vi "AO_master_DM_WFS_v3.vi"() -> ()   [LabVIEW 2018]
uses:
  <userlib>/WaveKit.lib/Controls/Image information.ctl
  <userlib>/WaveKit.lib/Controls/Image general information.ctl
  <userlib>/WaveKit.lib/Controls/Image acquisition information.ctl
  <userlib>/WaveKit.lib/Controls/Point2D.ctl
  <userlib>/WaveKit.lib/Controls/Data alignment enum.ctl
  <userlib>/WaveKit.lib/Controls/StatisticsData.ctl
  <userlib>/WaveKit.lib/Controls/Wavefront Corrector states - ONE.ctl
  Drivers and controls/ASI/ASI_VIs/ASI Library/Shared_Serial/Axis Name.ctl
  <userlib>/WaveKit.lib/Classes/Camera/Camera.lvclass
  <userlib>/WaveKit.lib/Classes/CameraSet/CameraSet.lvclass
  <userlib>/WaveKit.lib/Classes/Image/Image.lvclass
  <userlib>/WaveKit.lib/Classes/Phase/Phase.lvclass
  <userlib>/WaveKit.lib/Controls/HasoSlopes.lvclass
  <userlib>/WaveKit.lib/Controls/Pupil.lvclass
  <userlib>/WaveKit.lib/Classes/WavefrontCorrector/WavefrontCorrector.lvclass
  <userlib>/WaveKit.lib/Classes/WavefrontCorrectorSet/WavefrontCorrectorSet.lvclass
  <userlib>/WaveKit.lib/Classes/HasoEngine/HasoEngine.lvclass
  <userlib>/WaveKit.lib/Controls/SlopesEngineSetup.ctl
  <userlib>/WaveKit.lib/Controls/WavefrontReconstructionMode.ctl
  <vilib>/Utility/file.llb/Read From Spreadsheet File (DBL).vi
  <vilib>/Analysis/1siggen.llb/Ramp Pattern by Delta.vi
  <userlib>/WaveKit.lib/Classes/ModalCoef/ModalCoef.lvclass
  <vilib>/Analysis/NI_AALBase.lvlib
panel:
  in  "Device Status":enum32{"DM", "WFS", "Camera", "Others"}(tab)=enum."Camera"
  out "DM Actuator Values":sgl[](graph)
  out "Initial State":T1[](array[typedef])
  out "ActuatorsNumber":i32
  out "Initial Positions":sgl[](array[numeric])
  out "Final Positions":sgl[](array[numeric])
  in  "Coef Min":dbl=-0.5 min=1.0
  in  "Coef Max":dbl=0.5 min=1.0
  out "Zernike Measured":dbl[](graph)
  out "Phase statistics":T2
  out "Phase values":sgl[][](graph)=[[nan, nan, nan, nan, nan, nan, nan, nan, nan, nan, nan, nan, nan, nan, nan, nan, nan, nan, nan, nan, nan, nan, nan, nan, nan, nan, nan, nan, nan, nan, nan, nan, nan, nan, nan, nan, nan, nan, nan, nan], [nan, nan, nan, nan, nan, nan, nan, nan, nan, nan, nan, nan, nan, nan, nan, nan, nan, nan, nan, nan, nan, nan, nan, nan, nan, nan, nan, nan, nan, nan, nan, nan, nan, nan, nan, nan, nan, nan, nan, nan], [nan, nan, nan, nan, nan, nan, nan, nan, nan, nan, nan, nan, nan, nan, nan, nan, nan, nan, nan, nan, nan, nan, nan, nan, nan, nan, nan, nan, nan, nan, nan, nan, nan, nan, nan, nan, nan, nan, nan, nan], [nan, nan, nan, nan, nan, nan, nan, nan, nan, nan, nan, nan, nan, nan, nan, nan, nan, nan, nan, nan, nan, nan, nan, nan, nan, nan, nan, nan, nan, nan, nan, nan, nan, nan, nan, nan, nan, nan, nan, nan], [nan, nan, nan, nan, nan, nan, nan, nan, nan, nan, nan, nan, nan, nan, -0.14441992, nan, 0.1501734, 0.22490476, 0.2674259, 0.28415325, 0.2792031, 0.2552752, 0.21375881, 0.15405469, nan, nan, nan, nan, nan, nan, nan, nan, nan, nan, nan, nan, nan, nan, nan, nan], [nan, nan, nan, nan, nan, nan, nan, nan, nan, nan, nan, nan, nan, nan, 0.19143742, 0.2795512, 0.33646506, 0.37099743, 0.3877919, 0.3894302, 0.37774685, 0.35447162, 0.3212538, 0.27904776, 0.22675864, 0.15897867, nan, nan, nan, nan, nan, nan, nan, nan, nan, nan, nan, nan, nan, nan], [nan, nan, nan, nan, nan, nan, nan, nan, nan, nan, nan, nan, nan, 0.22618562, 0.290776, 0.33285964, 0.36044422, 0.3767934, 0.38285175, 0.37884915, 0.3652757, 0.3433441, 0.3149789, 0.28229773, 0.2464756, 0.20580466, 0.15268901, 0.06923797, nan, nan, nan, nan, nan, nan, nan, nan, nan, nan, nan, nan], [nan, nan, nan, nan, nan, nan, nan, nan, nan, nan, nan, nan, 0.19992779, 0.24616541, 0.27565512, 0.29675642, 0.31222007, 0.32191983, 0.32467726, 0.31943765, 0.30597392, 0.2852214, 0.25927368, 0.2309889, 0.20308714, 0.17653626, 0.14795627, 0.10568966, 0.024115691, nan, nan, nan, nan, nan, nan, nan, nan, nan, nan, nan], [nan, nan, nan, nan, nan, nan, nan, nan, nan, nan, nan, 0.14862825, 0.18219855, 0.20114602, 0.21551609, 0.22862102, 0.24014233, 0.24817906, 0.2505626, 0.24567793, 0.23295718, 0.21313797, 0.18829979, 0.16161954, 0.1367108, 0.11633411, 0.10019377, 0.081457645, 0.04156301, -0.057204023, nan, nan, nan, nan, nan, nan, nan, nan, nan, nan], [nan, nan, nan, nan, nan, nan, nan, nan, nan, nan, 0.08899155, 0.117771566, 0.12948777, 0.13732892, 0.14631097, 0.15688494, 0.16728252, 0.17497937, 0.17758016, 0.17335457, 0.16157834, 0.14275661, 0.11873307, 0.09261118, 0.06834036, 0.04974218, 0.038678437, 0.031985473, 0.016725859, -0.03676957, nan, nan, nan, nan, nan, nan, nan, nan, nan, nan], [nan, nan, nan, nan, nan, nan, nan, nan, nan, nan, 0.058377307, 0.069048055, 0.0725615, 0.07683456, 0.0840318, 0.09335055, 0.10271386, 0.1097376, 0.11226265, 0.10867052, 0.09812171, 0.08078306, 0.058033932, 0.032565817, 0.008214329, -0.010712444, -0.020921554, -0.022825297, -0.02489755, -0.05023362, -0.14592764, nan, nan, nan, nan, nan, nan, nan, nan, nan], [nan, nan, nan, nan, nan, nan, nan, nan, nan, -0.0018393314, 0.018310271, 0.023098737, 0.024714457, 0.027986258, 0.033823933, 0.041292578, 0.048749834, 0.054400377, 0.056548227, 0.05374936, 0.04499338, 0.029967438, 0.009379062, -0.014759185, -0.03905803, -0.059140373, -0.070816256, -0.0724436, -0.06894927, -0.07806298, -0.1393881, nan, nan, nan, nan, nan, nan, nan, nan, nan], [nan, nan, nan, nan, nan, nan, nan, nan, nan, -0.03322208, -0.017045017, -0.0123043535, -0.010394985, -0.007970343, -0.0042642877, 0.0003761826, 0.005164365, 0.009095938, 0.010986101, 0.009512841, 0.0033822758, -0.008344227, -0.02579559, -0.047820807, -0.071688615, -0.09321856, -0.107681155, -0.11187886, -0.10789668, -0.10908524, -0.14891545, -0.29341945, nan, nan, nan, nan, nan, nan, nan, nan], [nan, nan, nan, nan, nan, nan, nan, nan, nan, nan, -0.043187555, -0.03622458, -0.033755217, -0.03278728, -0.03198469, -0.030707732, -0.028716512, -0.026208155, -0.023933899, -0.023217455, -0.025771504, -0.03328519, -0.04682974, -0.06620631, -0.08943447, -0.1126552, -0.13079928, -0.13944486, -0.13836564, -0.13734597, -0.16491348, -0.2807172, nan, nan, nan, nan, nan, nan, nan, nan], [nan, nan, nan, nan, nan, nan, nan, nan, -0.13038255, -0.08328184, -0.060542934, -0.050779276, -0.048053104, -0.048984695, -0.05126809, -0.053124577, -0.05330209, -0.051303368, -0.04760214, -0.04368073, -0.041799206, -0.04448101, -0.05377527, -0.07043236, -0.09320336, -0.118551016, -0.14113419, -0.15550357, -0.15952203, -0.16009864, -0.18189941, -0.27977645, nan, nan, nan, nan, nan, nan, nan, nan], [nan, nan, nan, nan, nan, nan, nan, nan, -0.15416794, -0.09987456, -0.07151361, -0.05893044, -0.056102008, -0.058817875, -0.063637674, -0.067669004, -0.06878706, -0.06599128, -0.059670344, -0.051622536, -0.044753395, -0.042448726, -0.04769562, -0.062100213, -0.08502676, -0.11315687, -0.14084403, -0.16171429, -0.1720384, -0.17647736, -0.19687745, -0.284868, -0.53908885, -1.12795, nan, nan, nan, nan, nan, nan], [nan, nan, nan, nan, nan, nan, nan, nan, -0.17633308, -0.1131372, -0.07876157, -0.06330658, -0.060116876, -0.063924976, -0.07015394, -0.07493687, -0.07548633, -0.07052183, -0.060539607, -0.047784284, -0.035856243, -0.028966732, -0.030924596, -0.044017438, -0.06802279, -0.099662215, -0.13288532, -0.16044727, -0.17731819, -0.18653797, -0.20820689, -0.29237592, -0.5366785, nan, nan, nan, nan, nan, nan, nan], [nan, nan, nan, nan, nan, nan, nan, nan, -0.19826387, -0.12505035, -0.08430402, -0.06564974, -0.061443567, -0.06527472, -0.07152294, -0.07554153, -0.07411167, -0.0658889, -0.05163869, -0.034133032, -0.017655006, -0.0071354215, -0.007018423, -0.020031396, -0.046107426, -0.08178567, -0.12048963, -0.15415914, -0.17678727, -0.19048853, -0.21480094, -0.2999987, -0.54526997, nan, nan, nan, nan, nan, nan, nan], [nan, nan, nan, nan, nan, nan, nan, nan, -0.2214154, -0.13693352, -0.08914254, -0.06661926, -0.06048554, -0.06317037, -0.0681367, -0.07015528, -0.065784656, -0.053790003, -0.035310905, -0.013662348, 0.0062713036, 0.01901285, 0.01972933, 0.005542416, -0.023349542, -0.06307545, -0.10643376, -0.14466219, -0.17119798, -0.18806857, -0.21562657, -0.30642, -0.5640642, nan, nan, nan, nan, nan, nan, nan], [nan, nan, nan, nan, nan, nan, nan, nan, -0.24718054, -0.14940841, -0.093277775, -0.0658183, -0.056708053, -0.05720259, -0.059951056, -0.05929426, -0.051715773, -0.036192447, -0.014265999, 0.010266874, 0.032073133, 0.04536258, 0.04520398, 0.028878966, -0.0030008797, -0.045963787, -0.092160165, -0.13235793, -0.16002774, -0.17817038, -0.20961209, -0.31157303, -0.5953845, nan, nan, nan, nan, nan, nan, nan], [nan, nan, nan, nan, nan, nan, nan, nan, -0.27748746, -0.16290864, -0.09610232, -0.062047683, -0.048735943, -0.04617936, -0.046241976, -0.042900223, -0.03261665, -0.014586102, 0.009311387, 0.03494107, 0.05674191, 0.068891875, 0.0666744, 0.04783368, 0.0136316735, -0.030755527, -0.0769404, -0.115639456, -0.14119013, -0.15893419, -0.19620675, -0.31774768, nan, nan, nan, nan, nan, nan, nan, nan], [nan, nan, nan, nan, nan, nan, nan, nan, -0.31623095, -0.17884897, -0.09729818, -0.0539262, -0.03469713, -0.028198741, -0.025418447, -0.019910373, -0.008048305, 0.010862423, 0.034768496, 0.05942371, 0.07931873, 0.0889112, 0.08400761, 0.06307276, 0.028166434, -0.014867521, -0.057410896, -0.09080534, -0.111413695, -0.12868427, -0.17697167, -0.3319423, nan, nan, nan, nan, nan, nan, nan, nan], [nan, nan, nan, nan, nan, nan, nan, nan, nan, -0.20170604, -0.09850275, -0.0411539, -0.0131010795, -0.0011654077, 0.0047943285, 0.01185911, 0.023955166, 0.041901454, 0.06374147, 0.08542206, 0.1018104, 0.10796184, 0.10047772, 0.0787158, 0.04554086, 0.007227666, -0.027947046, -0.052963093, -0.06777905, -0.08820889, -0.15871821, nan, nan, nan, nan, nan, nan, nan, nan, nan], [nan, nan, nan, nan, nan, nan, nan, nan, nan, -0.24239759, -0.10614249, -0.026831074, 0.015322472, 0.03581071, 0.046350636, 0.05505173, 0.06651187, 0.08204405, 0.10016226, 0.11737824, 0.12928592, 0.13183476, 0.12261822, 0.10192663, 0.073240966, 0.042765103, 0.017522467, 0.0014635092, -0.0110412, -0.045025453, -0.15884721, nan, nan, nan, nan, nan, nan, nan, nan, nan], [nan, nan, nan, nan, nan, nan, nan, nan, nan, nan, -0.13597216, -0.021381527, 0.04426403, 0.07956008, 0.09847209, 0.110732496, 0.122154154, 0.13505057, 0.14887714, 0.16113368, 0.16849175, 0.16803522, 0.1584293, 0.14075197, 0.118653886, 0.09743117, 0.0815231, 0.06987105, 0.048498146, -0.020404778, nan, nan, nan, nan, nan, nan, nan, nan, nan, nan], [nan, nan, nan, nan, nan, nan, nan, nan, nan, nan, nan, -0.04876471, 0.05625415, 0.117832564, 0.15310521, 0.17423762, 0.18897903, 0.20128381, 0.21210447, 0.22038196, 0.22418612, 0.221881, 0.21311647, 0.19937092, 0.1836943, 0.16922635, 0.15598845, 0.13537171, 0.081669986, nan, nan, nan, nan, nan, nan, nan, nan, nan, nan, nan], [nan, nan, nan, nan, nan, nan, nan, nan, nan, nan, nan, nan, 0.014031529, 0.121263236, 0.18738765, 0.22803904, 0.25380248, 0.2710389, 0.28282017, 0.2899857, 0.29225817, 0.2892868, 0.28139976, 0.26978248, 0.25571787, 0.23844866, 0.21115, 0.15442081, nan, nan, nan, nan, nan, nan, nan, nan, nan, nan, nan, nan], [nan, nan, nan, nan, nan, nan, nan, nan, nan, nan, nan, nan, nan, nan, 0.15212902, 0.2306162, 0.28129596, 0.31381333, 0.33402625, 0.3450995, 0.34855807, 0.34515002, 0.33529556, 0.31882071, 0.29360068, 0.25266168, nan, nan, nan, nan, nan, nan, nan, nan, nan, nan, nan, nan, nan, nan], [nan, nan, nan, nan, nan, nan, nan, nan, nan, nan, nan, nan, nan, nan, nan, nan, 0.1979487, 0.2623494, 0.30271748, 0.32490522, 0.33223343, 0.3261181, 0.30614072, 0.26925305, nan, nan, nan, nan, nan, nan, nan, nan, nan, nan, nan, nan, nan, nan, nan, nan], [nan, nan, nan, nan, nan, nan, nan, nan, nan, nan, nan, nan, nan, nan, nan, nan, nan, nan, nan, nan, nan, nan, nan, nan, nan, nan, nan, nan, nan, nan, nan, nan, nan, nan, nan, nan, nan, nan, nan, nan], [nan, nan, nan, nan, nan, nan, nan, nan, nan, nan, nan, nan, nan, nan, nan, nan, nan, nan, nan, nan, nan, nan, nan, nan, nan, nan, nan, nan, nan, nan, nan, nan, nan, nan, nan, nan, nan, nan, nan, nan], [nan, nan, nan, nan, nan, nan, nan, nan, nan, nan, nan, nan, nan, nan, nan, nan, nan, nan, nan, nan, nan, nan, nan, nan, nan, nan, nan, nan, nan, nan, nan, nan, nan, nan, nan, nan, nan, nan, nan, nan]] caption="Wavefront"
  out "HASO intensity":u32[][](graph)
  out "Intensity Graph":i32[][](graph)
  in  "Intensity Max":dbl=10000.0 min=1.0
  in  "Intensity Min":dbl=200.0 min=1.0
  in  "Auto Scale":bool=TRUE caption="PD Correction"
  out "Detector X Pixels":i32
  out "Detector Y Pixels":i32
  out "Current Temp":i32
  out "FOV X Pixels":i32
  out "FOV Y Pixels":i32
  out "Running Status":T3(ring) caption="Camera FOV"
  out "EMCCD Status":bool
  out "Return from Start Acquisition":u32
  out "Return from GetAcquiredData":u32
  out "Return from SetSpool":i32=1
  out "Return from GetStatus":u32
  out "Get Exposure Time":sgl format="%.4f"
  out "Return from CheckTimings":u32
  out "Get Accum Time":sgl format="%.4f"
  out "Get Kinetic Time":sgl format="%.4f"
  out "Get EMCCD Gain":i32=1
  out "Get Kinetic Num":i32=1
  out "Return from CheckProcess":u32
  in  "error in (no error)":errorcluster
  out "Current error":errorcluster
  out "AO output":path=path "D:/Data"
  out "nb_images (get)":u32=10
  out "exposure_duration_us (get)":u32
  out "Base Path":path=path "D:/Data"
  out "EMCCD output":path=path "D:/Data"
  out "Current status":string="Test1"
  out "HASO ready":bool
  in  "Live Wavefront":bool
  in  "Update DM":bool
  in  "Tab Control":T4(tab)
  in  "EMCCD trigger port":tag="Dev1/port0/line0"
  in  "strPalette":string="C:\\Program Files\\Andor SOLIS\\GREY.PAL"
  in  "Initial haso file":path=path "D:/SystemAlignment/system_aberration_residual_20220406.has"
  in  "interaction matrix file":path=path "D:/SystemAlignment/IM_20220706_1p5sx2_0p5um.aomi"
  in  "DM configuration file":path=path "C:/Program Files (x86)/Imagine Optic/Configuration Files/WaveFrontCorrector_mirao52-e_0326.dat"
  in  "Haso configuration file":path=path "C:/Program Files (x86)/Imagine Optic/Configuration Files/HASO3_first_7364.dat"
  in  "Main Path":path=path "D:/Data"
  in  "Folder Name":string="Test"
  in  "Z Offset (um)":dbl
  in  "Abort":bool
  in  "Snap":bool
  in  "Acquire":bool
  in  "Enable EMCCD":bool caption="PD Correction"
  in  "TurnOFFCooler":bool caption="PD Correction"
  in  "Shutdown EMCCD when exit":bool caption="PD Correction"
  in  "VISA Stage":refnum<visa-resource-name>="COM5"
  in  "Update FOV":bool
  in  "Yend":i32=1002
  in  "Xend":i32=1004
  in  "Ystart":i32=2
  in  "Xstart":i32=2
  in  "Ybin":i32=1
  in  "Xbin":i32=1
  in  "Camera FOV":T5(ring)=enum."Full FOV"
  in  "Update AcqSetting":bool
  in  "Exposure time (s)":dbl=0.02
  in  "Kinetic Num":u32=1
  in  "Accum Num":u32=1
  in  "Aquisition Mode":T6(ring)=enum."Single Scan" caption="Camera FOV"
  in  "Trigger Mode":enum16{"Internal", "External"}(ring) caption="Camera FOV"
  in  "Gain Value":sgl=20.0 format="%.2f"
  in  "Gain On":bool=TRUE caption="Cameras Live Display"
  in  "488 shutter":refnum<k7>(container)
  in  "Live EMCCD":bool
  in  "Initialize EMCCD":bool=TRUE caption="PD Correction"
  in  "CoolToTargetTemp":bool=TRUE caption="PD Correction"
  in  "Set Temp":i32=-60
  in  "Subfolder EMCCD":string="test"
  in  "File Name":string="test"
  in  "Z Step Num":i32=9
  in  "Z Step Size (um)":dbl=0.4
  in  "right":bool
  in  "left":bool
  in  "front":bool
  in  "back":bool
  in  "XY step":dbl=1.0
  in  "down":bool
  in  "up":bool
  in  "Z step":dbl=1.0
  in  "flip mirror button":bool
  out "Response:":string="0\r"
  out "Position (um)":dbl[](array[numeric])=[0.0, 0.0, 0.0, -92.0, nan, nan] format="%#.1f"
  in  "Axis":T7[](array[typedef])=[enum."X", enum."Y", enum."Z", enum."Z", enum."F", enum."V"]
  in  "Command":string="W X"
  in  "Get Position":bool
  in  "Send":bool
  in  "Record Batch Actuator PD":bool
  in  "Record Batch Actuator":bool
  in  "Coef value":dbl=0.5 min=1.0
  in  "Idx end":u32=20 min=1
  in  "Idx start":u32=1 min=1
  in  "Subfolder":string="Test1"
  in  "Net Rp":bool
  in  "Input type":T8(ring)=enum."Zernike Coef"
  in  "Additional Command":bool=TRUE
  in  "Offset command file":path=path "D:/SystemAlignment/system_aberration_20220720.dat"
  in  "Initial offset":bool=TRUE
  in  "Additional file":path=path "D:/SystemAlignment/system_aberration_20191029.dat"
  out "Coef out":sgl[](array[numeric])
  out "Index out":i32[](array[numeric])
  in  "Zern/DM index in":i32[](array[numeric])
  in  "Zern/DM coef in":sgl[](array[numeric])
  in  "idxType":enum16{"Wyant", "ANSI"}(ring)=enum."ANSI"
  in  "Filter":u8[](array[numeric])
  in  "exposure_duration_s (set)":dbl=1.0 min=1.0
  in  "nb_images (set)":u32=1 min=1
  in  "Save File":bool
  in  "File Base Name":string="Test"
  in  "Record Response":bool
  in  "Record Batch Zern":bool
  out "Acquisition information":T9={"Image general information"={"Camera serial number"="", "Smearing removed"=FALSE, "Background image removed"=FALSE, "Time Stamp"=timestamp(0 s since 1904-01-01), "Comment"="", "Camera_MAX_Level"=0}, "Acquisition information"={"Exposure duration (us)"=0, "Exposure duration specified (us)"=0, "Gain"=0.0, "Number of summed images"=0, "Trigger type"=""}, "Number of pixels"={"X"=0, "Y"=0}, "Number of bits"=enum."16"}
  in  "Init":bool
  in  "Reset error":bool
  in  "Exit":bool
  in  "Stop HASO":bool
  in  "Start HASO":bool
  # "AO_master_DM_WFS_v2.vi: (last update: 20220425)\nControl deformable mirror and wavefront sensor, check DM response, EMCCD preview and acquisition\n1, EMCCD control: stack acquisition (by moving to absolute Z position);\n2,  Current bugs: 1) error --> shut down devices; 2) exit --> next initialization fails\na) DM ocuppied due to last unnormal exit; b) wavefront measure error: no laser, wrong slopes;"
  # "um"
  # "Available only if \"Live Wavefront\" is OFF"
  # "Not work well"
  # "Sample Stage"
  # "It takes some time to cool down the camera before it shutdowns"
  # "Button defined by camera coordinates"
  # "WF switch"
  # "x: +"
  # "z: +"
  # "C"
  # "y: -"
  # "1um = 10"
  # "Acquisition Settings"
  # "WFS no tilt: X502, Y520 @EMCCD"
  # "HASO Parameters"
  # "Check DM Response"
  # "Need to turn OFF live wavefront"
  # "Batch Range"
  # "Show in Wyant convention"
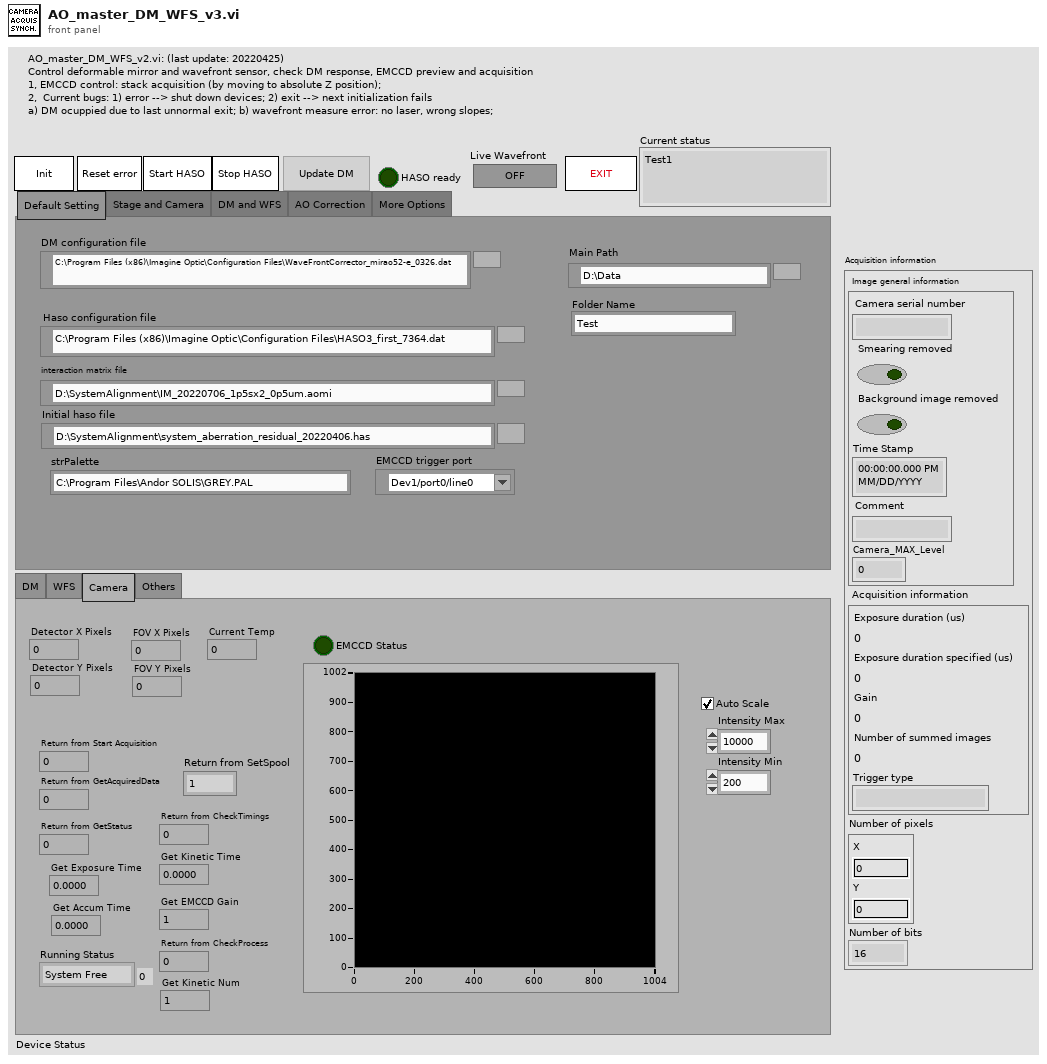
[diagram p1: front panel]
types:
  T1 = typedef "Wavefront Corrector states - ONE.ctl" = cluster{"Max":sgl, "Min":sgl, "Validity":enum16{"valid", "fixed", "invalid"}, "Fixed_Position":sgl}
  T2 = typedef "StatisticsData.ctl" = cluster{"PV":sgl, "RMS":dbl, "Max":sgl, "Min":sgl}
  T3 = enum16{"System Free", "Live Preview", "Snap", " Acquisition", ""}
  T4 = enum32{"Default Setting", "Stage and Camera", "DM and WFS", "AO Correction", "More Options"}
  T5 = enum16{"Custom FOV", "Full FOV", "FOV: 768x768", "FOV: 512x512", "FOV: 320x320", "FOV: 256x256", ""}
  T6 = enum16{"None", "Single Scan", "Accumulate", "Kinetics", "Fast Kinetics", "Run till abort"}
  T7 = typedef "Axis Name.ctl" = enum8{"undefined", "A", "B", "C", "D", "E", "F", "G", "H", "I", "J", "K", "L", "M", "N", "O", "P", "Q", "R", "S", "T", "U", "V", "W", "X", "Y", "Z"}
  T8 = enum16{"Zero Input", "Command File", "Zernike Coef", "Zernike File", "DM actuators"}
  T9 = typedef "Image information.ctl" = cluster{"Image general information":T10, "Acquisition information":T11, "Number of pixels":T12, "Number of bits":T13}
  T10 = typedef "Image general information.ctl" = cluster{"Camera serial number":string, "Smearing removed":bool, "Background image removed":bool, "Time Stamp":timestamp, "Comment":string, "Camera_MAX_Level":i32}
  T11 = typedef "Image acquisition information.ctl" = cluster{"Exposure duration (us)":i32, "Exposure duration specified (us)":i32, "Gain":sgl, "Number of summed images":i32, "Trigger type":string}
  T12 = typedef "Point2D.ctl" = cluster{"X":u32, "Y":u32}
  T13 = typedef "Data alignment enum.ctl" = enum16{"8", "16", "32"}
  T14 = typedef "SlopesEngineSetup.ctl" = cluster{"Start sub-aperture":T12, "Pupil average":dbl}
  T15 = typedef "CameraSpecifications.ctl" = cluster{"Grabber name":string, "Camera name":string, "Camera sn":string, "Pixels_um":T16, "Maximum level":u32, "Data alignment":T13, "Is signed":bool, "Acquisition start":T12, "Acquisition length":T12, "MaxFrameRate_Hz":sgl, "Chip type":enum16{"Progressive scan", "Frame transfert"}}
  T16 = typedef "General dimensions definition.ctl" = cluster{"Size":T12, "Step":T17}
  T17 = typedef "Point2Df.ctl" = cluster{"X":sgl, "Y":sgl}
  T18 = typedef "Wavefront Corrector Position.ctl" = sgl[]
  T19 = typedef "WavefrontReconstructionMode.ctl" = enum16{"None", "Modal_Legendre", "Modal_Zernike", "Zonal", "Modal_Zonal_Zernike", "Modal_Zonal_Legendre"}
  T20 = typedef "Error Code Enum typedef.ctl" = enum32{"N/A (0)", "DRV_ERROR_CODES", "DRV_SUCCESS", "DRV_VXDNOTINSTALLED", "DRV_ERROR_SCAN", "DRV_ERROR_CHECK_SUM", "DRV_ERROR_FILELOAD", "DRV_UNKNOWN_FUNC", "DRV_ERROR_VXD_INIT", "DRV_ERROR_ADDRESS", "DRV_ERROR_PAGELOCK", "DRV_ERROR_PAGEUNLOCK", "DRV_ERROR_BOARDTEST", "DRV_ERROR_ACK", "DRV_ERROR_UP_FIFO", "DRV_ERROR_PATTERN", "N/A (16)", "DRV_ACQUISITION_ERRORS", "DRV_ACQ_BUFFER", "DRV_ACQ_DOWNFIFO_FULL", "DRV_PROC_UNKONWN_INSTRUCTION", "DRV_ILLEGAL_OP_CODE", "DRV_KINETIC_TIME_NOT_MET", "DRV_ACCUM_TIME_NOT_MET", "DRV_NO_NEW_DATA", "N/A (25)", "DRV_SPOOLERROR", "N/A (27)", "N/A (28)", "N/A (29)", "N/A (30)", "N/A (31)", "N/A (32)", "DRV_TEMPERATURE_CODES", "DRV_TEMPERATURE_OFF", "DRV_TEMPERATURE_NOT_STABILIZED", "DRV_TEMPERATURE_STABILIZED", "DRV_TEMPERATURE_NOT_REACHED", "DRV_TEMPERATURE_OUT_RANGE", "DRV_TEMPERATURE_NOT_SUPPORTED", "DRV_TEMPERATURE_DRIFT", "N/A (41)", "N/A (42)", "N/A (43)", "N/A (44)", "N/A (45)", "N/A (46)", "N/A (47)", "N/A (48)", "DRV_GENERAL_ERRORS", "DRV_INVALID_AUX", "DRV_COF_NOTLOADED", "DRV_FPGAPROG", "DRV_FLEXERROR", "DRV_GPIBERROR", "N/A (55)", "N/A (56)", "N/A (57)", "N/A (58)", "N/A (59)", "N/A (60)", "N/A (61)", "N/A (62)", "N/A (63)", "DRV_DATATYPE", "DRV_DRIVER_ERRORS", "DRV_P1INVALID", "DRV_P2INVALID", "DRV_P3INVALID", "DRV_P4INVALID", "DRV_INIERROR", "DRV_COFERROR", "DRV_ACQUIRING", "DRV_IDLE", "DRV_TEMPCYCLE", "DRV_NOT_INITIALIZED", "DRV_P5INVALID", "DRV_P6INVALID", "DRV_INVALID_MODE", "DRV_INVALID_FILTER", "DRV_I2CERRORS", "DRV_I2CDEVNOTFOUND", "DRV_I2CTIMEOUT", "DRV_P7INVALID", "N/A (84)", "N/A (85)", "N/A (86)", "N/A (87)", "N/A (88)", "N/A (89)", "DRV_IOCERROR", "DRV_VRMVERSIONERROR"}
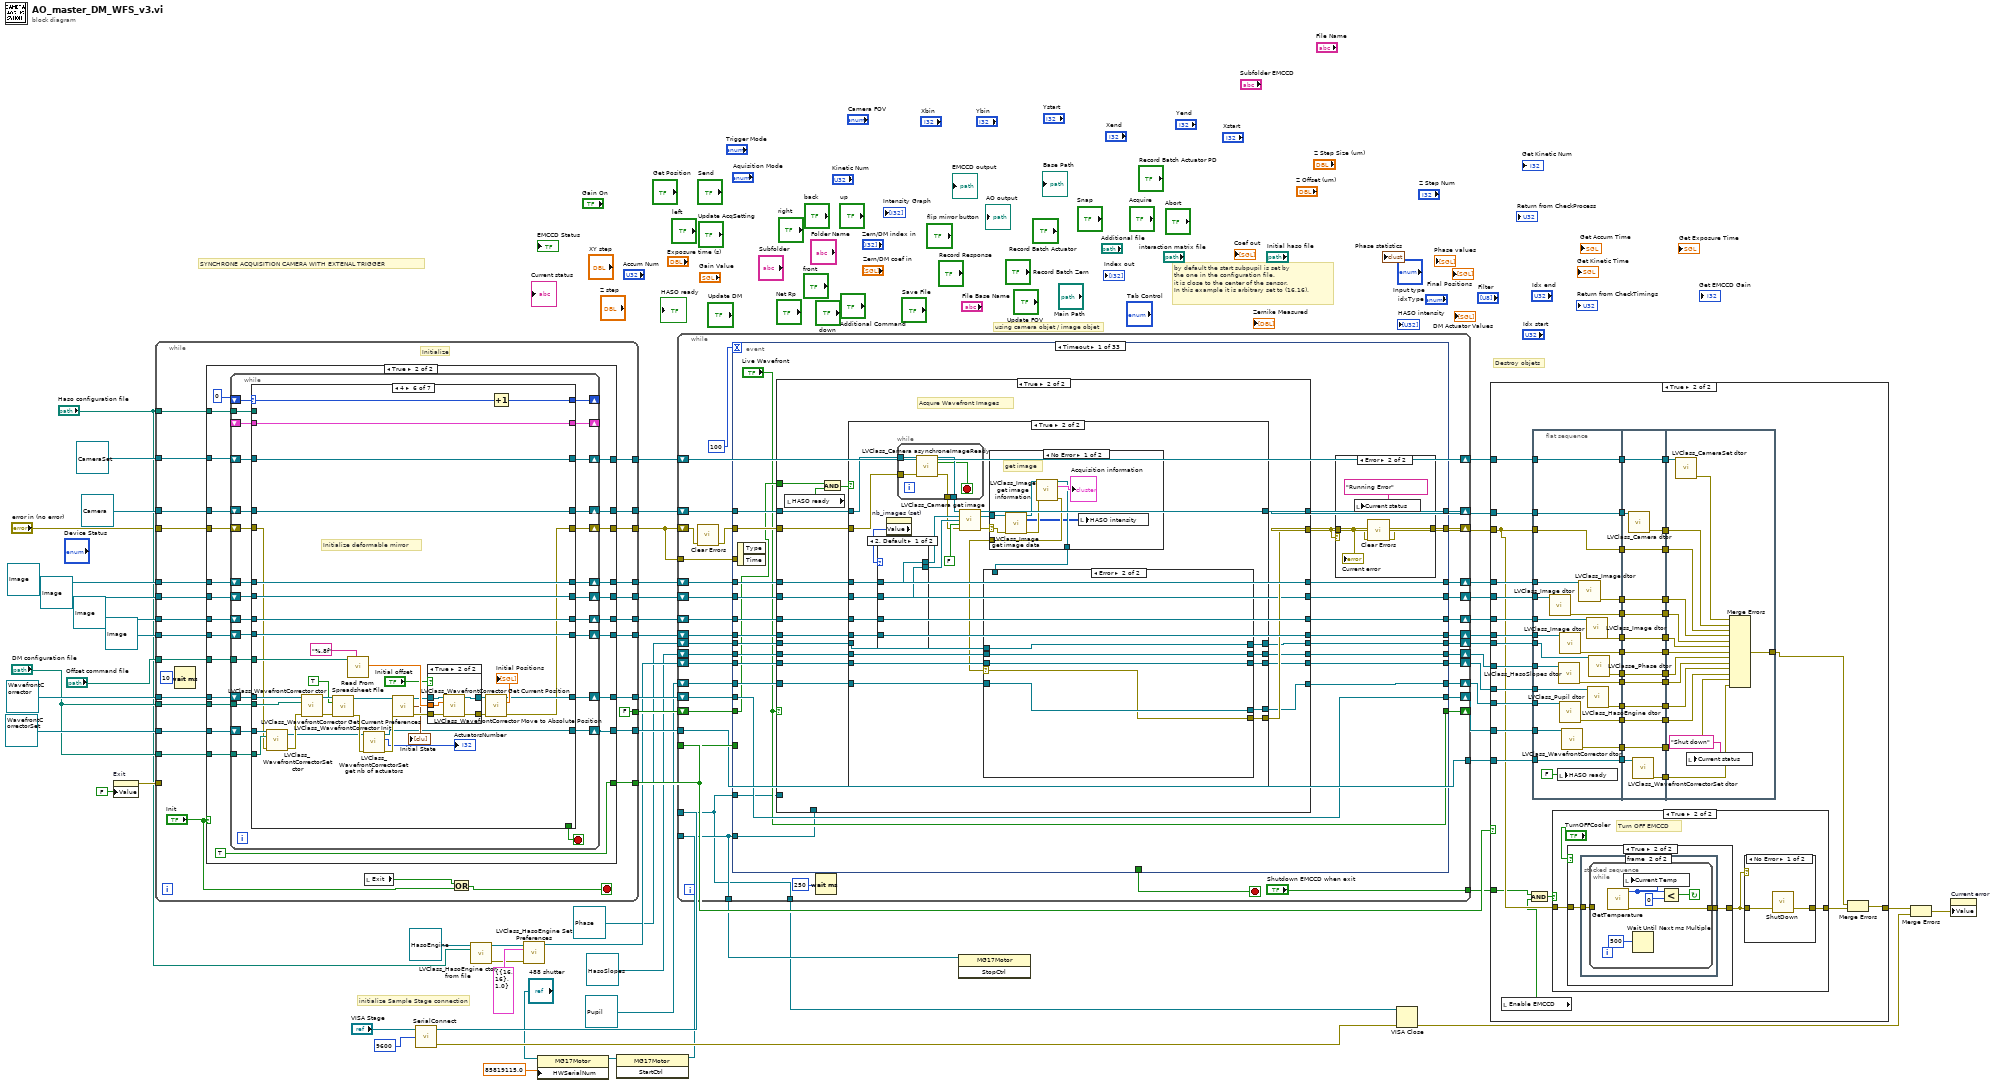
[diagram p0: block diagram]
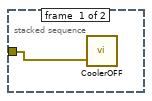
[diagram p5: hidden frame]
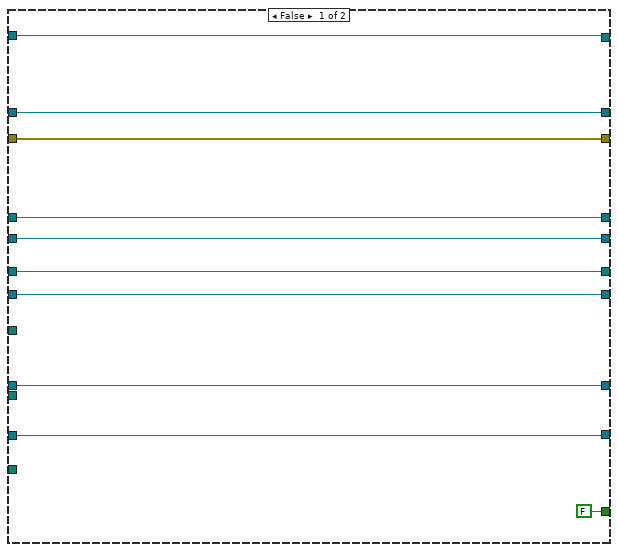
[diagram p7: hidden frame]
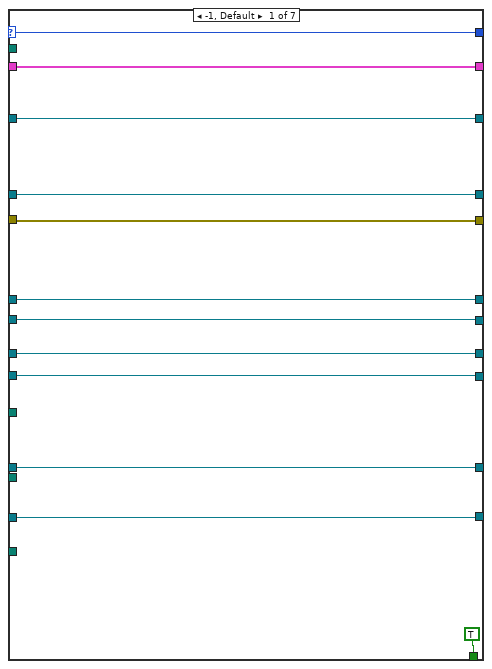
[diagram p8: hidden frame]
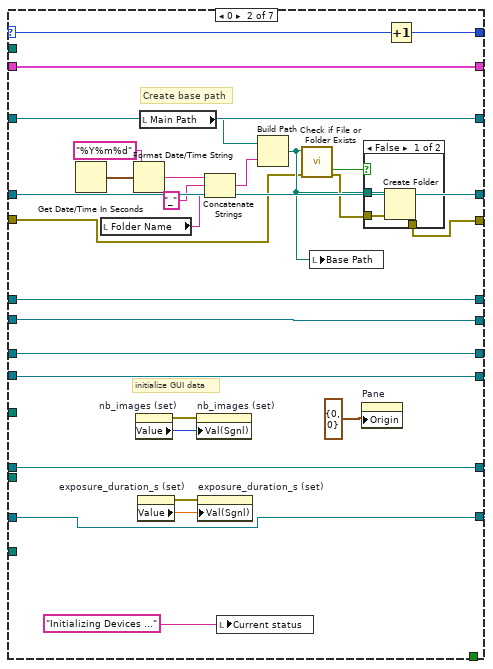
[diagram p9: hidden frame]
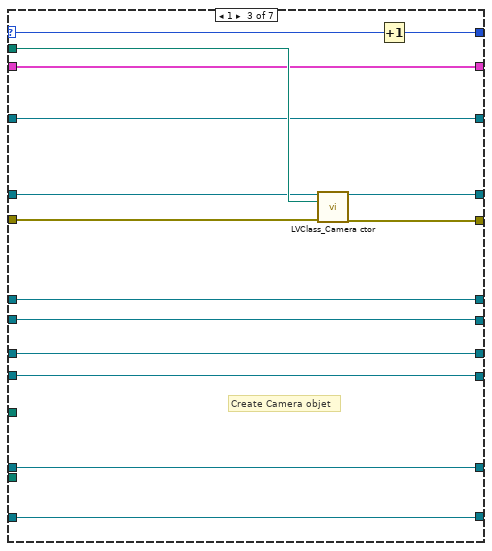
[diagram p11: hidden frame]
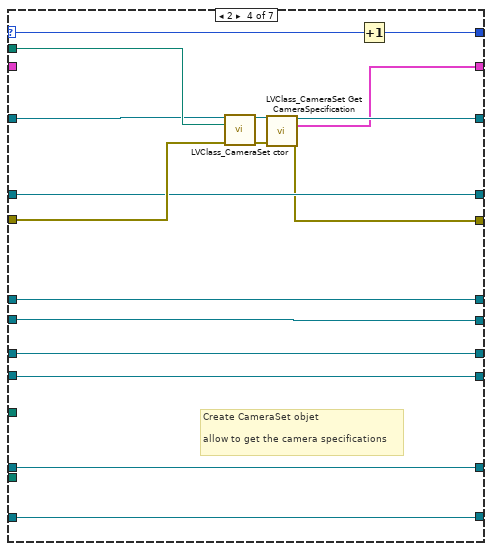
[diagram p12: hidden frame]
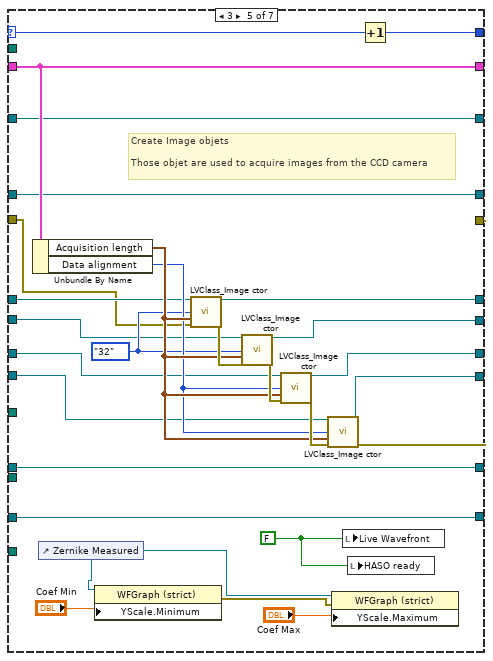
[diagram p13: hidden frame]
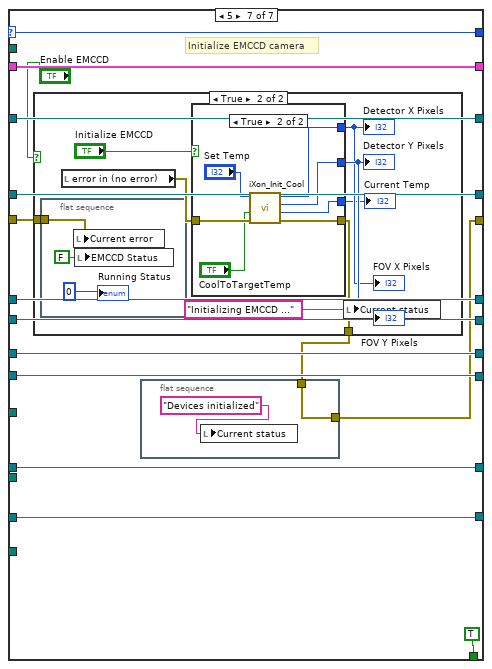
[diagram p15: hidden frame]
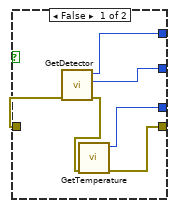
[diagram p17: hidden frame]
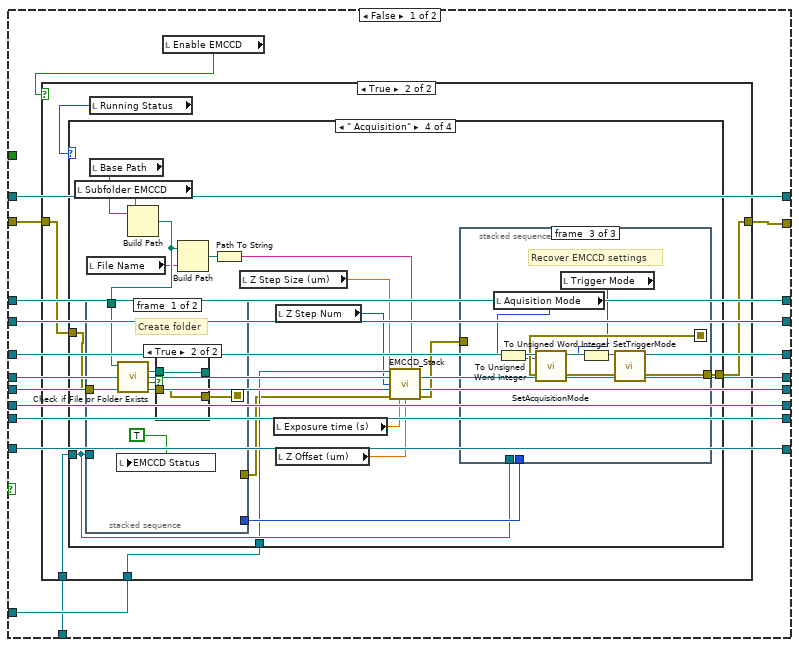
[diagram p19: hidden frame]
diagram:
  # "initialize Sample Stage connection"
  # "by default the start subpupil is set by \nthe one in the configuration file. \nit is close to the center of the sensor.\nIn this example it is arbitrary set to (16,16)."
  # "Destroy objets"
  # "using camera objet / image objet"
  # "SYNCHRONE ACQUISITION CAMERA WITH EXTENAL TRIGGER"
  n1 = property on="Exit" class="Bool (strict)"("Value"=FALSE ("Exit")) -> (error out=w37:errorcluster)  [unwired: 2 in, 1 out]
  n2 = while {
    tunnel: [FALSE] -> w53
    tunnel: [w87] -> w52
    tunnel: [w86] -> w51
    tunnel: [w85] -> w50
    tunnel: [w84] -> w49
    tunnel: [w83] -> w48
    tunnel: [w82] -> w47
    tunnel: refnum<class "Camera.lvclass"> refnum ("Camera.lvclass") -> [w81]
    tunnel: refnum<class "CameraSet.lvclass"> refnum ("CameraSet.lvclass") -> [w80]
    tunnel: refnum<class "Image.lvclass"> refnum ("Image in") -> [w79]
    tunnel: refnum<class "Image.lvclass"> refnum ("Image in") -> [w78]
    tunnel: refnum<class "Image.lvclass"> refnum ("Image in") -> [w77]
    tunnel: refnum<class "Image.lvclass"> refnum ("Image in") -> [w76]
    tunnel: "error in (no error)" -> [w75]
    tunnel: [w74] -> w40
    tunnel: [w72] -> w39
    tunnel: w37 -> [_]
    tunnel: "Haso configuration file" -> [w68]
    tunnel: "Offset command file" -> [w67]
    tunnel: refnum<class "WavefrontCorrectorSet.lvclass"> refnum ("WavefrontCorrectorSet in") -> [w66]
    tunnel: "DM configuration file" -> [w65]
    tunnel: refnum<class "WavefrontCorrector.lvclass"> refnum ("WavefrontCorrector in") -> [w64]
    tunnel: "DM configuration file" -> [w63]
    tunnel: [w62] -> w32
    tunnel: [w61] -> w31
    stop <- w69 stop-if-true
    # "Initialize"
    n3 = Wait (ms)(milliseconds to wait=u32 10) -> ()  [unwired: 1 out]
    n4 = case shown="True" "Init" {
      tunnel: [w98 w122] -> w87
      tunnel: [w97 w121] -> w86
      tunnel: [w95 w120] -> w85
      tunnel: [w94 w119] -> w84
      tunnel: [w93 w118] -> w83
      tunnel: [w92 w117] -> w82
      tunnel: w81 -> [w98 w116]
      tunnel: w80 -> [w97 w114]
      tunnel: w79 -> [w95 w113]
      tunnel: w78 -> [w94 w112]
      tunnel: w77 -> [w93 w111]
      tunnel: w76 -> [w92 w110]
      tunnel: w75 -> [w96 w109]
      tunnel: [w96 w108] -> w74
      tunnel: [FALSE TRUE] -> w72
      tunnel: w68 -> [_ w106]
      tunnel: w67 -> [_ w105]
      tunnel: w66 -> [w89 w99]
      tunnel: w65 -> [_ w104]
      tunnel: w64 -> [w90 w100]
      tunnel: w63 -> [_ w103]
      tunnel: [w90 w102] -> w62
      tunnel: [w89 w101] -> w61
      frame False {
      }
      frame True {
        n5 = while {
          tunnel: w106 -> [w147]
          shift-right: [w149] -> w122
          shift-left: w116 -> [w141]
          shift-right: [w131] -> _
          shift-left: 0 -> [w130]
          shift-right: [w148] -> w121
          shift-left: w114 -> [w140]
          shift-right: [w139] -> _
          shift-left: _ -> [w137]
          shift-right: [w146] -> w120
          shift-left: w113 -> [w138]
          shift-right: [w145] -> w119
          shift-left: w112 -> [w136]
          shift-right: [w144] -> w118
          shift-left: w111 -> [w134]
          shift-right: [w143] -> w117
          shift-left: w110 -> [w135]
          shift-right: [w142] -> w108
          shift-left: w109 -> [w132]
          tunnel: w105 -> [w129]
          tunnel: w104 -> [w128]
          tunnel: w103 -> [w127]
          shift-right: [w126] -> w102
          shift-left: w100 -> [w124]
          shift-right: [w125] -> w101
          shift-left: w99 -> [w123]
          stop <- w133 stop-if-true
          n6 = case shown="4" w130 {
            tunnel: [w161 w177 w209 w219 w241 w290 w312] -> w149
            tunnel: w147 -> [_ _ w208 w223 _ _ _]
            tunnel: [w160 w181 w206 w224 w242 w289 w311] -> w148
            tunnel: [w153 w182 w200 w214 w248 w284 w305] -> w146
            tunnel: [w154 w183 w201 w215 w247 w285 w306] -> w145
            tunnel: [w155 w184 w202 w216 w246 w286 w307] -> w144
            tunnel: [w156 w185 w203 w217 w245 w287 w308] -> w143
            tunnel: [w157 w163 w205 w218 w244 w258 w298] -> w142
            selector: w130 -> [w152 w179 w198 w213 w236 w256 w304]
            tunnel: w141 -> [w161 w177 w207 w219 w241 w290 w312]
            tunnel: w140 -> [w160 w181 w206 w222 w242 w289 w311]
            tunnel: [w158 w178 w204 w221 w243 w288 w309] -> w139
            tunnel: w138 -> [w153 w182 w200 w214 w240 w284 w305]
            tunnel: w137 -> [w158 w178 w204 _ w243 w288 w309]
            tunnel: w136 -> [w154 w183 w201 w215 w239 w285 w306]
            tunnel: w135 -> [w156 w185 w203 w217 w238 w287 w308]
            tunnel: w134 -> [w155 w184 w202 w216 w237 w286 w307]
            tunnel: [TRUE _ _ _ _ _ TRUE] -> w133
            tunnel: w132 -> [w157 w164 w197 w220 w234 w259 w301]
            tunnel: [w152 w180 w199 w212 w235 w255 w304] -> w131
            tunnel: w129 -> [_ _ _ _ _ w266 _]
            tunnel: w123 -> [w150 w175 w195 w210 w232 w264 w302]
            tunnel: w128 -> [_ _ _ _ _ w263 _]
            tunnel: w124 -> [w151 w176 w196 w211 w233 w262 w303]
            tunnel: w127 -> [_ _ _ _ _ w261 _]
            tunnel: [w151 w176 w196 w211 w233 w260 w303] -> w126
            tunnel: [w150 w175 w195 w210 w232 w257 w302] -> w125
            frame -1, Default {
            }
            frame 0 {
              # "Create base path"
              # "initialize GUI data"
              n7 = Get Date/Time In Seconds() -> (seconds since 1Jan1904=w169:timestamp)
              n8 = local read "Folder Name"() -> (w173:string)
              n9 = Format Date/Time String(time format string (%c)="%Y%m%d", seconds (now)=w169) -> (date/time string=w170:string)  [unwired: 1 in]
              n10 = property on="nb_images (set)" class="DigNum (strict)"() -> (error out=w190:errorcluster, "Value"=w189:u32)  [unwired: 2 in, 1 out]
              n11 = property on="exposure_duration_s (set)" class="DigNum (strict)"() -> (error out=w186:errorcluster, "Value"=w188:dbl)  [unwired: 2 in, 1 out]
              n12 = local read "Main Path"() -> (w172:path)
              n13 = property on="nb_images (set)" class="DigNum (strict)"(error in=w190, "Val(Sgnl)"=w189) -> ()  [unwired: 1 in, 2 out]
              n14 = property on="exposure_duration_s (set)" class="DigNum (strict)"(error in=w186, "Val(Sgnl)"=w188) -> ()  [unwired: 1 in, 2 out]
              n15 = Concatenate Strings(w170, "_", w173) -> (w171:string)
              n16 = local write "Current status"("Initializing Devices ...") -> ()
              n17 = Build Path(base path=w172, name or relative path=w171) -> (appended path=w165:path)
              n18 = call <vilib>:"Check if File or Folder Exists.vi"("error in (no error)"=w164, "path"=w165) -> ("error out"=w174:errorcluster, "file or folder exists?"=w168:bool)  [unwired: 7 in, 1 out]
              n19 = local write "Base Path"(w165) -> ()
              n20 = property on="Pane" class="Pane"("Origin"=cluster{"Horizontal":i16, "Vertical":i16} {"Horizontal"=0, "Vertical"=0} ("Front Panel Window:Origin")) -> ()  [unwired: 2 in, 2 out]
              n21 = case shown="False" w168 {
                tunnel: w165 -> [w193 _]
                tunnel: w174 -> [w192 w194]
                tunnel: [w191 w194] -> w163
                frame False {
                  n22 = Create Folder(path (use dialog)=w193, error in=w192) -> (error out=w191:errorcluster)  [unwired: 1 in, 2 out]
                }
                frame True {
                }
              }
              n23 = Increment(x=w179) -> (x+1=w180:i32)
            }
            frame 1 {
              # "Create Camera objet"
              n24 = call <userlib>:"LVClass_Camera ctor.vi"("Camera"=w207, "Configuration file path"=w208, "error in (no error)"=w197) -> ("Camera (new)"=w209:refnum<class "Camera.lvclass">, "error out"=w205:errorcluster)  [unwired: 11 in]
              n25 = Increment(x=w198) -> (x+1=w199:i32)
            }
            frame 2 {
              # "Create CameraSet objet\n\nallow to get the camera specifications"
              n26 = call <userlib>:"LVClass_CameraSet ctor.vi"("CameraSet.lvclass"=w222, "Configuration file path"=w223, "error in (no error)"=w220) -> ("CameraSet.lvclass"=w226:refnum<class "CameraSet.lvclass">, "error out"=w225:errorcluster)  [unwired: 11 in]
              n27 = call <userlib>:"LVClass_CameraSet Get CameraSpecification.vi"("CameraSet.lvclass"=w226, "error in (no error)"=w225) -> ("CameraSet.lvclass"=w224:refnum<class "CameraSet.lvclass">, "Camera Config"=w221:T15, "error out"=w218:errorcluster)  [unwired: 11 in]
              n28 = Increment(x=w213) -> (x+1=w212:i32)
            }
            frame 3 {
              w231 = FALSE
              w249 = Data_alignment_enum."32" ("Data alignment")
              # "Create Image objets\n\nThose objet are used to acquire images from the CCD camera"
              n29 = Unbundle By Name(w243) -> ("Acquisition length"=w251:T12, "Data alignment"=w250:T13)
              n30 = control-ref of="Zernike Measured"() -> (w228:refnum<vi>)
              n31 = property on="Property Node" class="WFGraph (strict)"(reference=w228, "YScale.Minimum"="Coef Min") -> (error out=w227:errorcluster)  [unwired: 1 in, 1 out]
              n32 = call <userlib>:"LVClass_Image ctor.vi"("Image in"=w240, "Data alignment"=w249, "Size"=w251, "error in (no error)"=w234) -> ("Image out"=w248:refnum<class "Image.lvclass">, "error out"=w252:errorcluster)  [unwired: 10 in]
              n33 = call <userlib>:"LVClass_Image ctor.vi"("Image in"=w239, "Data alignment"=w249, "Size"=w251, "error in (no error)"=w252) -> ("Image out"=w247:refnum<class "Image.lvclass">, "error out"=w253:errorcluster)  [unwired: 10 in]
              n34 = call <userlib>:"LVClass_Image ctor.vi"("Image in"=w237, "Data alignment"=w250, "Size"=w251, "error in (no error)"=w253) -> ("Image out"=w246:refnum<class "Image.lvclass">, "error out"=w254:errorcluster)  [unwired: 10 in]
              n35 = call <userlib>:"LVClass_Image ctor.vi"("Image in"=w238, "Data alignment"=w250, "Size"=w251, "error in (no error)"=w254) -> ("Image out"=w245:refnum<class "Image.lvclass">, "error out"=w244:errorcluster)  [unwired: 10 in]
              n36 = property on="Property Node" class="WFGraph (strict)"(reference=w228, error in=w227, "YScale.Maximum"="Coef Max") -> ()  [unwired: 2 out]
              n37 = local write "Live Wavefront"(w231) -> ()
              n38 = local write "HASO ready"(w231) -> ()
              n39 = Increment(x=w236) -> (x+1=w235:i32)
            }
            frame 4 {
              (unwired) "DM "
              (unwired) "DM "
              # "Initialize deformable mirror"
              n40 = call <userlib>:"LVClass_WavefrontCorrectorSet ctor.vi"("WavefrontCorrectorSet in"=w264, "PathToWavefrontCorrectorSetupFile"=w263, "error in (no error)"=w259) -> ("WavefrontCorrectorSet out"=w271:refnum<class "WavefrontCorrectorSet.lvclass">, "error out"=w280:errorcluster)  [unwired: 11 in]
              n41 = call <userlib>:"LVClass_WavefrontCorrector ctor.vi"("WavefrontCorrector in"=w262, "PathToWavefrontCorrectorSetupFile"=w261, "error in (no error)"=w280) -> ("WavefrontCorrector out"=w268:refnum<class "WavefrontCorrector.lvclass">, "error out"=w269:errorcluster)  [unwired: 11 in]
              n42 = call <userlib>:"LVClass_WavefrontCorrector Init.vi"("WavefrontCorrector in"=w268, "set_init_state_from_config_file"=TRUE, "error in (no error)"=w269) -> ("WavefrontCorrector out"=w272:refnum<class "WavefrontCorrector.lvclass">, "error out"=w281:errorcluster)  [unwired: 11 in]
              n43 = call-poly <vilib>:"Read From Spreadsheet File.vi"("format (%.3f)"="%.8f", "file path (dialog if empty)"=w266) -> ("first row"=w283:dbl[])  [unwired: 5 in, 4 out]
              n44 = call <userlib>:"LVClass_WavefrontCorrectorSet get nb of actuators.vi"("WavefrontCorrectorSet in"=w271, "error in (no error)"=w281) -> ("WavefrontCorrectorSet out"=w257:refnum<class "WavefrontCorrectorSet.lvclass">, "ActuatorsNumber"=→"ActuatorsNumber":i32, "error out"=w282:errorcluster)  [unwired: 11 in]
              n45 = call <userlib>:"LVClass_WavefrontCorrector Get Current Preferences.vi"("WavefrontCorrector in"=w272, "error in (no error)"=w282) -> ("WavefrontCorrector out"=w277:refnum<class "WavefrontCorrector.lvclass">, "Mirror preferences.Wavefront Corrector State"=→"Initial State":T1[], "error out"=w278:errorcluster)  [unwired: 10 in, 1 out]
              n46 = case shown="True" "Initial offset" {
                tunnel: w283 -> [_ w297]
                tunnel: [w292 w296] -> w275
                tunnel: [w291 w295] -> w276
                tunnel: w277 -> [w292 w294]
                tunnel: w278 -> [w291 w293]
                frame False {
                }
                frame True {
                  n47 = call <userlib>:"LVClass_WavefrontCorrector Move to Absolute Position.vi"("WavefrontCorrector in"=w294, "Absolute Positions"=w297, "error in (no error)"=w293) -> ("WavefrontCorrector out"=w296:refnum<class "WavefrontCorrector.lvclass">, "error out"=w295:errorcluster)  [unwired: 11 in]
                }
              }
              n48 = call <userlib>:"LVClass_WavefrontCorrector Get Current Position.vi"("WavefrontCorrector in"=w275, "error in (no error)"=w276) -> ("WavefrontCorrector out"=w260:refnum<class "WavefrontCorrector.lvclass">, "Wavefront Corrector Position"=→"Initial Positions":T18, "error out"=w258:errorcluster)  [unwired: 11 in]
              n49 = Increment(x=w256) -> (x+1=w255:i32)
            }
            frame 5 {
              # "Initialize EMCCD camera"
              n50 = case shown="True" "Enable EMCCD" {
                tunnel: w301 -> [w315 w319]
                tunnel: [w315 w317] -> w299
                frame False {
                }
                frame True {
                  n51 = flat-sequence {
                    tunnel: w319 -> [w326]
                    frame #0 {
                      n52 = local write "Current error"(w326) -> ()
                      n53 = local write "EMCCD Status"(FALSE) -> ()
                      "Running Status" <- u16 0
                    }
                  }
                  n54 = local read "error in (no error)"() -> (w316:errorcluster)
                  n55 = case shown="True" "Initialize EMCCD" {
                    tunnel: w316 -> [w331 w338]
                    tunnel: [w329 w336] -> w322
                    tunnel: [w328 w335] -> w323
                    tunnel: [w332 w334] -> w321
                    tunnel: [w327 w333] -> w317
                    frame False {
                      n56 = call <userlib>:"GetDetector.vi"("error in (no error)"=w331) -> ("error out"=w330:errorcluster, "ypixels"=w328:i32, "xpixels"=w329:i32)  [unwired: 3 in, 1 out]
                      n57 = call <userlib>:"GetTemperature.vi"("error in (no error)"=w330) -> ("error out"=w327:errorcluster, "temperature"=w332:i32)  [unwired: 3 in, 2 out]
                    }
                    frame True {
                      n58 = call "iXon_Init_Cool.vi"("error in (no error)"=w338, "CoolToTargetTemp"="CoolToTargetTemp", "Set Temp"="Set Temp") -> ("error out"=w333:errorcluster, "Current Temp"=w334:i32, "Detector Y Pixels"=w335:i32, "Detector X Pixels"=w336:i32)  [unwired: 5 in]
                    }
                  }
                  "Detector X Pixels" <- w322
                  "Detector Y Pixels" <- w323
                  "Current Temp" <- w321
                  "FOV X Pixels" <- w322
                  "FOV Y Pixels" <- w323
                  n59 = local write "Current status"("Initializing EMCCD ...") -> ()
                }
              }
              n60 = flat-sequence {
                tunnel: w299 -> [w313]
                tunnel: [w313] -> w298
                frame #0 {
                  n61 = local write "Current status"("Devices initialized") -> ()
                }
              }
            }
          }
        }
      }
    }
    n62 = local read "Exit"() -> (w71:bool)
    n63 = Or(x=w71, y="Init") -> (x .or. y?=w69:bool)
  }
  n64 = call "SerialConnect.vi"("baud rate (9600)"=9600, "VISA resource name"="VISA Stage") -> ("error out"=w6:errorcluster, "VISA out"=w12:refnum<visa-resource-name>)  [unwired: 1 in, 1 out]
  n65 = call <userlib>:"LVClass_HasoEngine ctor from file.vi"("HasoEngine in"=refnum<class "HasoEngine.lvclass"> refnum, "Configuration file path"="Haso configuration file") -> ("HasoEngine out"=w28:refnum<class "HasoEngine.lvclass">, "error out"=w29:errorcluster)  [unwired: 12 in]
  n66 = call <userlib>:"LVClass_HasoEngine Set Preferences.vi"("HasoEngine in"=w28, "Slopes_HasoEngine_Setup"=T14 {"Start sub-aperture"={"X"=16, "Y"=16}, "Pupil average"=1.0}, "error in (no error)"=w29) -> ("HasoEngine out"=w25:refnum<class "HasoEngine.lvclass">)  [unwired: 11 in, 1 out]
  n67 = property class="MG17Motor"(reference="488 shutter", "HWSerialNum"=85819115.0) -> (reference out=w4:refnum<k7>)  [unwired: 1 in, 1 out]
  n68 = invoke class="MG17Motor" method="StartCtrl"(reference=w4) -> (reference out=w1:refnum<k7>)  [unwired: 2 in, 2 out]
  n69 = while {
    shift-right: [w372] -> w60
    shift-left: w40 -> [w341]
    shift-right: [w370] -> w59
    shift-left: w52 -> [w371]
    shift-right: [w364] -> w58
    shift-left: w50 -> [w369]
    shift-right: [w363] -> w57
    shift-left: w49 -> [w368]
    shift-right: [w362] -> w56
    shift-left: w48 -> [w367]
    shift-right: [w361] -> w55
    shift-left: w47 -> [w366]
    shift-right: [w360] -> _
    shift-left: w53 -> [w365]
    shift-right: [w359] -> w54
    shift-left: w51 -> [w359]
    tunnel: w40 -> [w358]
    tunnel: w39 -> [w357]
    tunnel: w31 -> [w346]
    shift-right: [w354] -> w24
    shift-left: refnum<class "HasoSlopes.lvclass"> refnum ("HasoSlopes in") -> [w353]
    shift-right: [w352] -> w19
    shift-left: w25 -> [w355]
    shift-right: [w349] -> w20
    shift-left: refnum<class "Phase.lvclass"> refnum ("Phase in") -> [w351]
    shift-right: [w348] -> w18
    shift-left: refnum<class "Pupil.lvclass"> refnum ("Pupil in") -> [w350]
    tunnel: [w346] -> w17
    shift-right: [w345] -> w16
    shift-left: w32 -> [w347]
    tunnel: w12 -> [w343]
    tunnel: w1 -> [w344]
    tunnel: [w344] -> w11
    tunnel: [w343] -> w10
    tunnel: ["Shutdown EMCCD when exit"] -> w5
    stop <- w373 stop-if-true
    n70 = call <vilib>:"Clear Errors.vi"("error in (no error)"=w341) -> ("error out"=w340:errorcluster)  [unwired: 5 in, 1 out]
    n71 = event shown="[0] Timeout" {
      selector: _ -> [_ _ _ _ _ _ _ _ _ _ _ _ _ _ _ _ _ _ _ _ _ _ _ _ _ _ _ _ _ _ _ _ _]
      dyn-events: _ -> [_ _ _ _ _ _ _ _ _ _ _ _ _ _ _ _ _ _ _ _ _ _ _ _ _ _ _ _ _ _ _ _ _]
      timeout: 100 -> [_ _ _ _ _ _ _ _ _ _ _ _ _ _ _ _ _ _ _ _ _ _ _ _ _ _ _ _ _ _ _ _ _]
      tunnel: w340 -> [w392 w704 w707 w720 _ w768 w784 w795 w829 w948 w990 w1103 w1124 w1132 w1140 w1148 w1156 w1164 w1173 w1187 w1201 w1215 w1229 w1243 w1256 w1286 w1299 w1327 w1884 w2413 w3167 _ w3482]
      tunnel: [_ _ _ _ _ _ _ _ _ _ _ _ _ _ _ _ _ _ _ _ _ _ _ _ _ _ _ w1328 w1885 w2414 w3168 "Exit" TRUE ("Exit")] -> w373
      tunnel: [w376 w702 w707 w720 w732 w763 w782 w795 w828 w947 w991 w1102 w1124 w1132 w1140 w1148 w1156 w1164 w1172 w1186 w1200 w1214 w1228 w1242 w1255 w1285 w1298 w1326 w1883 w2412 w3166 w3466 w3487] -> w372
      tunnel: w371 -> [w397 w703 w708 w721 w741 w767 w785 w808 w824 w946 w1012 w1101 w1126 w1134 w1142 w1150 w1158 w1166 w1176 w1190 w1204 w1218 w1232 w1246 w1263 w1292 w1305 w1315 w1872 w2401 w3157 w3467 w3489]
      tunnel: [w396 w701 w708 w721 w741 w764 w783 w809 w824 w946 w1012 w1101 w1126 w1134 w1142 w1150 w1158 w1166 w1176 w1190 w1204 w1218 w1232 w1246 w1263 w1292 w1305 w1315 w1872 w2401 w3157 w3465 w3488] -> w370
      tunnel: w369 -> [w400 w694 w715 w728 w743 w757 w781 w804 w839 w971 w1017 w1111 w1130 w1138 w1146 w1154 w1162 w1170 w1184 w1198 w1212 w1226 w1240 w1254 w1267 w1296 w1309 w1322 w1879 w2408 w3162 w3461 w3483]
      tunnel: w368 -> [w399 w695 w716 w729 w744 w758 w780 w805 w838 w970 w1016 w1110 w1129 w1137 w1145 w1153 w1161 w1169 w1183 w1197 w1211 w1225 w1239 w1253 w1266 w1295 w1308 w1321 w1878 w2407 w3161 w3462 w3484]
      tunnel: w367 -> [w398 w696 w717 w730 w745 w759 w779 w806 w837 w969 w1015 w1109 w1128 w1136 w1144 w1152 w1160 w1168 w1182 w1196 w1210 w1224 w1238 w1252 w1265 w1294 w1307 w1320 w1877 w2406 w3160 w3463 w3485]
      tunnel: w366 -> [w393 w697 w718 w731 w746 w760 w778 w807 w836 w968 w1014 w1108 w1127 w1135 w1143 w1151 w1159 w1167 w1181 w1195 w1209 w1223 w1237 w1251 w1264 w1293 w1306 w1319 w1876 w2405 w3159 w3464 w3486]
      tunnel: w365 -> [w380 w693 w714 w727 w742 w756 w770 w796 w825 w945 w1013 w1100 w1125 w1133 w1141 w1149 w1157 w1165 w1174 w1188 w1202 w1216 w1230 w1244 w1262 w1291 w1304 w1324 w1881 w2410 w3164 _ _]
      tunnel: [w395 w694 w715 w728 w743 w757 w781 w804 w839 w971 w1017 w1111 w1130 w1138 w1146 w1154 w1162 w1170 w1184 w1198 w1212 w1226 w1240 w1254 w1267 w1296 w1309 w1322 w1879 w2408 w3162 w3461 w3483] -> w364
      tunnel: [w394 w695 w716 w729 w744 w758 w780 w805 w838 w970 w1016 w1110 w1129 w1137 w1145 w1153 w1161 w1169 w1183 w1197 w1211 w1225 w1239 w1253 w1266 w1295 w1308 w1321 w1878 w2407 w3161 w3462 w3484] -> w363
      tunnel: [w391 w696 w717 w730 w745 w759 w779 w806 w837 w969 w1015 w1109 w1128 w1136 w1144 w1152 w1160 w1168 w1182 w1196 w1210 w1224 w1238 w1252 w1265 w1294 w1307 w1320 w1877 w2406 w3160 w3463 w3485] -> w362
      tunnel: [w390 w697 w718 w731 w746 w760 w778 w807 w836 w968 w1014 w1108 w1127 w1135 w1143 w1151 w1159 w1167 w1181 w1195 w1209 w1223 w1237 w1251 w1264 w1293 w1306 w1319 w1876 w2405 w3159 w3464 w3486] -> w361
      tunnel: ["Live Wavefront" w693 w714 w727 w742 w756 w770 w796 w825 w945 w1013 w1100 w1125 w1133 w1141 w1149 w1157 w1165 w1174 w1188 w1202 w1216 w1230 w1244 w1262 w1291 w1304 w1324 w1881 w2410 w3164 FALSE FALSE] -> w360
      tunnel: w358 -> [_ _ _ _ w739 _ _ _ _ _ _ _ _ _ _ _ _ _ _ _ _ _ _ _ _ _ _ _ _ _ _ _ _]
      tunnel: w357 -> [_ _ _ _ _ _ _ _ _ _ _ _ _ _ _ _ _ _ _ _ _ _ _ _ _ _ _ _ _ _ _ w3459 _]
      tunnel: w353 -> [w389 w691 w712 w725 w737 w750 w776 w802 w821 _ _ _ _ _ _ _ _ _ _ _ _ _ _ _ _ _ _ w1317 w1874 w2403 w3142 w3457 w3479]
      tunnel: w355 -> [w388 w690 w711 w724 w736 w749 w775 w801 w820 _ _ _ _ _ _ _ _ _ _ _ _ _ _ _ _ _ _ w1316 w1873 w2402 w3158 w3456 w3478]
      tunnel: [w387 w691 w712 w725 w737 w750 w776 w802 w821 _ _ _ _ _ _ _ _ _ _ _ _ _ _ _ _ _ _ w1314 w1871 w2400 w3142 w3457 w3479] -> w354
      tunnel: [w386 w690 w711 w724 w736 w749 w775 w801 w820 _ _ _ _ _ _ _ _ _ _ _ _ _ _ _ _ _ _ w1316 w1873 w2402 w3158 w3456 w3478] -> w352
      tunnel: w351 -> [w385 w692 w713 w726 w738 w751 w777 w803 w822 _ _ _ _ _ _ _ _ _ _ _ _ _ _ _ _ _ _ w1318 w1875 w2404 w3143 w3458 w3480]
      tunnel: w350 -> [w384 w689 w710 w723 w735 w748 w774 w800 w819 _ _ _ _ _ _ _ _ _ _ _ _ _ _ _ _ _ _ w1312 w1869 w2398 w3141 w3455 w3477]
      tunnel: [w383 w692 w713 w726 w738 w751 w777 w803 w822 _ _ _ _ _ _ _ _ _ _ _ _ _ _ _ _ _ _ w1313 w1870 w2399 w3143 w3458 w3480] -> w349
      tunnel: [w382 w689 w710 w723 w735 w748 w774 w800 w819 _ _ _ _ _ _ _ _ _ _ _ _ _ _ _ _ _ _ w1311 w1868 w2397 w3141 w3455 w3477] -> w348
      tunnel: w347 -> [w381 w688 w709 w722 w734 w747 w773 w799 w827 _ _ _ _ _ _ _ _ _ _ _ _ _ _ _ _ _ _ w1325 w1882 w2411 w3165 w3454 w3476]
      tunnel: [w381 w688 w709 w722 w734 w747 w773 w799 w823 _ _ _ _ _ _ _ _ _ _ _ _ _ _ _ _ _ _ w1323 w1880 w2409 w3163 w3454 w3476] -> w345
      tunnel: w343 -> [w378 _ _ _ _ _ _ _ _ _ _ _ _ _ _ _ _ _ w1175 w1189 w1203 w1217 w1231 w1245 _ w1284 w1297 _ _ _ w3139 _ _]
      tunnel: w344 -> [w377 _ _ _ _ _ _ _ _ _ _ _ _ _ _ _ _ _ _ _ _ _ _ _ _ _ _ _ _ _ w3140 _ _]
      event Timeout {
        n72 = event-data() -> ()  [unwired: 1 in, 2 out]
        n73 = case shown="True" "Live Wavefront" {
          tunnel: [w407 w588] -> w375
          tunnel: w400 -> [w418 w591]
          tunnel: [w418 w591] -> w395
          tunnel: [w414 w587] -> w394
          tunnel: w398 -> [w417 w590]
          tunnel: w393 -> [w416 w589]
          tunnel: [w417 w590] -> w391
          tunnel: [w416 w589] -> w390
          tunnel: w399 -> [w414 w587]
          tunnel: w397 -> [w415 w585]
          tunnel: [w415 w586] -> w396
          tunnel: w392 -> [w408 w584]
          tunnel: w389 -> [w412 w583]
          tunnel: w388 -> [w411 w582]
          tunnel: [w412 w581] -> w387
          tunnel: [w411 w580] -> w386
          tunnel: w385 -> [w413 w579]
          tunnel: w384 -> [w410 w578]
          tunnel: [w413 w577] -> w383
          tunnel: [w410 w576] -> w382
          tunnel: w380 -> [_ w573]
          tunnel: w378 -> [w406 _]
          tunnel: w377 -> [w405 _]
          frame False {
            n74 = local read "Enable EMCCD"() -> (w409:bool)
            n75 = case shown="True" w409 {
              tunnel: w408 -> [w419 w423]
              tunnel: [w419 w420] -> w407
              tunnel: w406 -> [_ w422]
              tunnel: w405 -> [_ w421]
              frame False {
              }
              frame True {
                n76 = local read "Running Status"() -> (w424:T3)
                n77 = case shown="\" Acquisition\"" w424 {
                  tunnel: w423 -> [w426 w430 w465 w539]
                  tunnel: w422 -> [_ _ _ w532]
                  tunnel: w421 -> [_ _ _ w533]
                  tunnel: [w425 w428 w457 w524] -> w420
                  frame "System Free", Default {
                    n78 = call <userlib>:"GetTemperature.vi"("error in (no error)"=w426) -> ("error out"=w425:errorcluster, "temperature"=w427:i32)  [unwired: 3 in, 2 out]
                    n79 = local write "Current Temp"(w427) -> ()
                  }
                  frame "Live Preview" {
                    n80 = stacked-sequence {
                      seq-local: [w433 _ _] -> [_ w438 _]
                      seq-local: [_ w437 _] -> [_ _ w452]
                      seq-local: [w432 _ _] -> [_ w436 _]
                      tunnel: w430 -> [w434 _ _]
                      tunnel: [_ _ w451] -> w428
                      frame #0 {
                        w435 = 20002  # DRV_SUCCESS
                        n81 = call <userlib>:"StartAcquisition.vi"("error in (no error)"=w434) -> ("error out"=w433:errorcluster, "DLL error code"=w431:u32)  [unwired: 1 in]
                        "Return from Start Acquisition" <- w431
                        n82 = Equal?(x=w435, y=w431) -> (x = y?=w432:bool)
                      }
                      frame #1 {
                        n83 = case shown="False" w436 {
                          tunnel: w438 -> [w439 w441]
                          tunnel: [w439 w440] -> w437
                          frame False {
                          }
                          frame True {
                            n84 = while {
                              tunnel: w441 -> [w443]
                              tunnel: [w442] -> w440
                              stop <- w444 continue-if-true
                              w446 = u16 72  # DRV ACQUIRING
                              n85 = call <userlib>:"GetStatus.vi"("error in (no error)"=w443) -> ("error out"=w442:errorcluster, "status"=w445:T20)  [unwired: 2 in, 1 out]
                              n86 = Equal?(x=w445, y=w446) -> (x = y?=w444:bool)
                            }
                          }
                        }
                      }
                      frame #2 {
                        n87 = local read "FOV X Pixels"() -> (w455:i32)
                        n88 = local read "FOV Y Pixels"() -> (w454:i32)
                        n89 = Multiply(x=w454, y=w455) -> (x*y=w456:i32)
                        n90 = call <userlib>:"GetAcquiredData.vi"("error in (no error)"=w452, "size"=w456) -> ("error out"=w451:errorcluster, "DLL error code"=→"Return from GetAcquiredData":u32, "array"=w447:i32[])  [unwired: 1 in]
                        n91 = Multiply(x=1, y=w447) -> (x*y=w448:i32[])
                        n92 = Reshape Array(w448, w454, w455) -> (w453:i32[][])
                        n93 = local write "Intensity Graph"(w453) -> ()
                      }
                    }
                    n94 = local write "EMCCD Status"(TRUE) -> ()
                  }
                  frame "Snap" {
                    n95 = flat-sequence {
                      tunnel: [w511] -> w467
                      tunnel: w465 -> [w513]
                      tunnel: w466 -> [w514]
                      frame #0 {
                        # "Create folder"
                        n96 = local write "EMCCD Status"(TRUE) -> ()
                        n97 = call <vilib>:"Check if File or Folder Exists.vi"("error in (no error)"=w513, "path"=w514) -> ("error out"=w512:errorcluster, "file or folder exists?"=w516:bool, "dup path"=w515:path)  [unwired: 7 in]
                        n98 = case shown="False" w516 {
                          tunnel: w515 -> [w521 w523]
                          tunnel: [w520 w523] -> _
                          tunnel: w512 -> [w519 w522]
                          tunnel: [w518 w522] -> w511
                          frame False {
                            n99 = Create Folder(path (use dialog)=w521, error in=w519) -> (created path=w520:path, error out=w518:errorcluster)  [unwired: 1 in, 1 out]
                          }
                          frame True {
                          }
                        }
                      }
                    }
                    n100 = local read "File Name"() -> (w458:string)
                    n101 = local read "Base Path"() -> (w460:path)
                    n102 = local read "Subfolder EMCCD"() -> (w459:string)
                    n103 = Build Path(base path=w460, name or relative path=w459) -> (appended path=w466:path)
                    n104 = Build Path(base path=w466, name or relative path=w458) -> (appended path=w464:path)
                    n105 = Path To String(path=w464) -> (string=w463:string)
                    n106 = local read "Kinetic Num"() -> (w462:u32)
                    n107 = stacked-sequence {
                      seq-local: [_ w477 _ _ _] -> [_ _ w480 _ _]
                      seq-local: [_ _ w479 _ _] -> [_ _ _ w486 _]
                      seq-local: [w472 _ _ _ _] -> [_ w476 _ _ _]
                      seq-local: [_ _ _ w487 _] -> [_ _ _ _ w506]
                      tunnel: w467 -> [w473 _ _ _ _]
                      tunnel: w463 -> [w474 _ _ w488 w504]
                      tunnel: w462 -> [_ _ _ _ w507]
                      tunnel: [_ _ _ _ w505] -> w461
                      frame #0 {
                        # "Set Spool"
                        n108 = call <userlib>:"SetSpool.vi"("active"=TRUE, "method"=2, "name"=w474, "framebuffersize (10)"=20, "error in (no error)"=w473) -> ("DLL error code"=→"Return from SetSpool":u32, "error out"=w472:errorcluster)  [unwired: 9 in]
                      }
                      frame #1 {
                        w478 = 20002  # DRV_SUCCESS
                        n109 = call <userlib>:"StartAcquisition.vi"("error in (no error)"=w476) -> ("error out"=w477:errorcluster, "DLL error code"=w475:u32)  [unwired: 1 in]
                        n110 = local write "Return from Start Acquisition"(w475) -> ()
                        n111 = Equal?(x=w478, y=w475) -> ()  [unwired: 1 out]
                      }
                      frame #2 {
                        n112 = while {
                          tunnel: w480 -> [w483]
                          tunnel: [w482] -> w479
                          stop <- w484 continue-if-true
                          w485 = u16 72  # DRV ACQUIRING
                          n113 = call <userlib>:"GetStatus.vi"("error in (no error)"=w483) -> ("error out"=w482:errorcluster, "status"=w481:T20)  [unwired: 2 in, 1 out]
                          "Return from GetStatus" <- w481
                          n114 = Equal?(x=w481, y=w485) -> (x = y?=w484:bool)
                        }
                      }
                      frame #3 {
                        # "Save acquisition"
                        n115 = case shown="\"TIFF\", Default" enum16{"TIFF", "Sif"}."TIFF" ("File Type") {
                          tunnel: "C:\\Program Files\\Andor SOLIS\\GREY.PAL" -> [w494 _]
                          tunnel: w488 -> [w497 w503]
                          tunnel: w486 -> [w495 w500]
                          tunnel: [w496 w499] -> w487
                          frame "TIFF", Default {
                            w491 = 1
                            n116 = Concatenate Strings(w497, ".tif") -> (w493:string)
                            n117 = call <userlib>:"SaveAsTiffEx.vi"("path"=w493, "palette"=w494, "position"=0, "type"=w491, "mode"=w491, "error in (no error)"=w495) -> ("error out"=w496:errorcluster)  [unwired: 12 in, 1 out]
                          }
                          frame "Sif" {
                            n118 = Concatenate Strings(w503, ".sif") -> (w501:string)
                            n119 = call <userlib>:"SaveAsSif.vi"("error in (no error)"=w500, "path"=w501) -> ("error out"=w499:errorcluster)  [unwired: 1 out]
                          }
                        }
                      }
                      frame #4 {
                        # "Clearn Spool Files"
                        n120 = call "cleanSpool.vi"("error in (no error)"=w506, "Total Img Num"=w507, "strPath"=w504) -> ("error out"=w505:errorcluster)  [unwired: 8 in]
                      }
                    }
                    n121 = flat-sequence {
                      tunnel: w461 -> [w508]
                      tunnel: [w508] -> w457
                      frame #0 {
                        n122 = local write "EMCCD Status"(FALSE) -> ()
                        n123 = local write "Running Status"(0) -> ()
                      }
                    }
                  }
                  frame " Acquisition" {
                    n124 = local read "Subfolder EMCCD"() -> (w536:string)
                    n125 = local read "File Name"() -> (w535:string)
                    n126 = local read "Base Path"() -> (w537:path)
                    n127 = Build Path(base path=w537, name or relative path=w536) -> (appended path=w540:path)
                    n128 = stacked-sequence {
                      seq-local: [w554 _] -> [_ w567]
                      tunnel: w539 -> [w556 _]
                      tunnel: w540 -> [w557 _]
                      tunnel: [_ w570] -> w529
                      tunnel: w533 -> [_ w571]
                      tunnel: [_ w569] -> w534
                      frame #0 {
                        # "Create folder"
                        n129 = local write "EMCCD Status"(TRUE) -> ()
                        n130 = call <vilib>:"Check if File or Folder Exists.vi"("error in (no error)"=w556, "path"=w557) -> ("error out"=w555:errorcluster, "file or folder exists?"=w559:bool, "dup path"=w558:path)  [unwired: 7 in]
                        n131 = case shown="True" w559 {
                          tunnel: w558 -> [w564 w566]
                          tunnel: [w563 w566] -> _
                          tunnel: w555 -> [w562 w565]
                          tunnel: [w561 w565] -> w554
                          frame False {
                            n132 = Create Folder(path (use dialog)=w564, error in=w562) -> (created path=w563:path, error out=w561:errorcluster)  [unwired: 1 in, 1 out]
                          }
                          frame True {
                          }
                        }
                      }
                      frame #1 {
                        # "Turn on laser"
                        n133 = invoke class="MG17Motor" method="SC_Enable"(reference=w571, error in=w567, "lChanID"=0) -> (error out=w570:errorcluster, "lChanID"=w569:i32)  [unwired: 1 in, 2 out]
                        n134 = Wait (ms)(milliseconds to wait=u32 1000) -> ()  [unwired: 1 out]
                      }
                    }
                    n135 = Build Path(base path=w540, name or relative path=w535) -> (appended path=w538:path)
                    n136 = Path To String(path=w538) -> (string=w525:string)
                    n137 = local read "Z Step Size (um)"() -> (w531:dbl)
                    n138 = local read "Exposure time (s)"() -> (w527:dbl)
                    n139 = local read "Z Step Num"() -> (w530:i32)
                    n140 = local read "Z Offset (um)"() -> (w526:dbl)
                    n141 = call "EMCCD_Stack.vi"("VISA Stage"=w532, "strPath"=w525, "Z Step Size (um)"=w531, "Step Num"=w530, "error in (no error)"=w529, "Exposure time (s)"=w527, "Offset"=w526) -> ("error out"=w528:errorcluster)  [unwired: 8 in]
                    n142 = stacked-sequence {
                      seq-local: [_ w543 _] -> [_ _ w552]
                      tunnel: w528 -> [_ w544 _]
                      tunnel: w534 -> [_ w546 _]
                      tunnel: w533 -> [_ w545 _]
                      tunnel: [_ _ w547] -> w524
                      frame #0 {
                        n143 = local write "EMCCD Status"(FALSE) -> ()
                        n144 = local write "Running Status"(0) -> ()
                      }
                      frame #1 {
                        # "Turn off laser"
                        n145 = invoke class="MG17Motor" method="SC_Disable"(reference=w545, error in=w544, "lChanID"=w546) -> (error out=w543:errorcluster)  [unwired: 1 in, 3 out]
                      }
                      frame #2 {
                        # "Recover EMCCD settings"
                        n146 = local read "Aquisition Mode"() -> (w550:T6)
                        n147 = To Unsigned Word Integer(number=w550) -> (unsigned 16bit integer=w551:u16)
                        n148 = call <userlib>:"SetAcquisitionMode.vi"("error in (no error)"=w552, "mode"=w551) -> ("error out"=w553:errorcluster)  [unwired: 1 out]
                        n149 = local read "Trigger Mode"() -> (w548:enum16{"Internal", "External"})
                        n150 = To Unsigned Word Integer(number=w548) -> (unsigned 16bit integer=w549:u16)
                        n151 = call <userlib>:"SetTriggerMode.vi"("error in (no error)"=w553, "mode"=w549) -> ("error out"=w547:errorcluster)  [unwired: 1 out]
                      }
                    }
                  }
                }
              }
            }
          }
          frame True {
            # "Acqure Wavefront Images"
            n152 = local read "HASO ready"() -> (w574:bool)
            n153 = And(x=w573, y=w574) -> (x .and. y?=w575:bool)
            n154 = case shown="True" w575 {
              tunnel: w591 -> [_ w621]
              tunnel: w590 -> [_ w620]
              tunnel: w589 -> [_ w619]
              tunnel: [w592 w616] -> w588
              tunnel: w587 -> [_ w613]
              tunnel: [w597 w612] -> w586
              tunnel: w585 -> [w597 w598]
              tunnel: w584 -> [w592 w599]
              tunnel: w583 -> [w595 w611]
              tunnel: w582 -> [w594 w610]
              tunnel: [w595 w609] -> w581
              tunnel: [w594 w608] -> w580
              tunnel: w579 -> [w596 w607]
              tunnel: w578 -> [w593 w606]
              tunnel: [w596 w605] -> w577
              tunnel: [w593 w604] -> w576
              frame False {
              }
              frame True {
                n155 = property on="nb_images (set)" class="DigNum (strict)"() -> ("Value"=w622:u32)  [unwired: 2 in, 2 out]
                n156 = case shown="2, Default" w622 {
                  tunnel: [w685 w687] -> w623
                  tunnel: w613 -> [w684 _]
                  tunnel: w621 -> [w685 _]
                  tunnel: [w684 w686] -> w618
                  tunnel: w620 -> [_ w687]
                  tunnel: w619 -> [_ w686]
                  frame 2, Default {
                  }
                  frame 1 {
                  }
                }
                n157 = while {
                  tunnel: w598 -> [w628]
                  tunnel: [w627] -> w600
                  tunnel: w599 -> [w625]
                  tunnel: [w624] -> w601
                  stop <- w626 stop-if-true
                  n158 = call <userlib>:"LVClass_Camera asynchroneImageReady.vi"("Camera in"=w628, "error in (no error)"=w625) -> ("Camera out"=w627:refnum<class "Camera.lvclass">, "ready"=w626:bool, "error out"=w624:errorcluster)  [unwired: 11 in]
                }
                n159 = call <userlib>:"LVClass_Camera get image.vi"("Camera in"=w600, "Image"=w623, "Image RAW"=w618, "remove_background"=FALSE, "error in (no error)"=w601) -> ("Camera out"=w612:refnum<class "Camera.lvclass">, "Image (dup)"=w617:refnum<class "Image.lvclass">, "error out"=w614:errorcluster)  [unwired: 7 in, 1 out]
                n160 = case shown="No Error" w614 {
                  selector: w614 -> [w681 w682]
                  tunnel: w617 -> [w678 w683]
                  tunnel: [w676 w683] -> w603
                  tunnel: [w675 w682] -> w602
                  frame No Error {
                    # "get image"
                    n161 = call <userlib>:"LVClass_Image get image data.vi"("Image in"=w678, "error in (no error)"=w681) -> ("Image out"=w680:refnum<class "Image.lvclass">, "Image data out"=w674:u32[][], "error out"=w679:errorcluster)  [unwired: 11 in]
                    n162 = call <userlib>:"LVClass_Image get image information.vi"("Image in"=w680, "error in (no error)"=w679) -> ("Image out"=w676:refnum<class "Image.lvclass">, "Acquisition information"=→"Acquisition information":T9, "error out"=w675:errorcluster)  [unwired: 11 in]
                    n163 = local write "HASO intensity"(w674) -> ()
                  }
                  frame Error {
                  }
                }
                n164 = case shown="Error" w602 {
                  selector: w602 -> [w638 w669]
                  tunnel: [w641 w669] -> w616
                  tunnel: w603 -> [w637 _]
                  tunnel: [w640 w670] -> w604
                  tunnel: [w639 w673] -> w605
                  tunnel: w611 -> [w636 w672]
                  tunnel: w610 -> [w635 w671]
                  tunnel: [w630 w672] -> w609
                  tunnel: [w634 w671] -> w608
                  tunnel: w607 -> [w633 w673]
                  tunnel: w606 -> [w632 w670]
                  frame No Error {
                    n165 = call "image2slopes.vi"("error in (no error)"=w638, "Image in"=w637, "HasoEngine in"=w635, "HasoSlopes in"=w636) -> ("error out"=w629:errorcluster, "HasoEngine out"=w634:refnum<class "HasoEngine.lvclass">, "HasoSlopes out"=w631:refnum<class "HasoSlopes.lvclass">)  [unwired: 4 in, 1 out]
                    n166 = case shown="Error" w629 {
                      tunnel: [w663 w665] -> w641
                      tunnel: [w661 w666] -> w640
                      tunnel: [w660 w668] -> w639
                      tunnel: w629 -> [w655 w665]
                      tunnel: w633 -> [w654 w668]
                      tunnel: w632 -> [w652 w666]
                      tunnel: w631 -> [w648 w667]
                      tunnel: [w646 w667] -> w630
                      frame No Error {
                        # "phase display"
                        n167 = local read "Filter"() -> (w651:u8[])
                        n168 = call "slopes2phase.vi"("TypePhase"=WavefrontReconstructionMode."Modal_Zernike", "Number of coefficients"=u8 32, "error in (no error)"=w655, "Filter"=w651, "HasoSlopes in"=w648, "Phase in"=w654) -> ("error out"=w645:errorcluster, "HasoSlopes out"=w647:refnum<class "HasoSlopes.lvclass">, "Phase out"=w653:refnum<class "Phase.lvclass">)  [unwired: 3 in]
                        n169 = local read "idxType"() -> (w642:enum16{"Wyant", "ANSI"})
                        n170 = call "slopes2zern.vi"("HasoSlopes in"=w647, "error in (no error)"=w645, "idxType"=w642) -> ("HasoSlopes out"=w646:refnum<class "HasoSlopes.lvclass">, "Zernike Coefficients"=w643:dbl[], "error out"=w644:errorcluster)  [unwired: 3 in, 2 out]
                        n171 = call <userlib>:"LVClass_Pupil ctor from HasoSlopes.vi"("Pupil in"=w652, "HasoSlopes.lvclass"=w648, "error in (no error)"=w644) -> ("Pupil out"=w658:refnum<class "Pupil.lvclass">, "error out"=w659:errorcluster)  [unwired: 11 in]
                        n172 = call <userlib>:"LVClasse_Phase GetStatisticDatas.vi"("Phase in"=w653, "error in (no error)"=w659) -> ("Phase out"=w664:refnum<class "Phase.lvclass">, "StatisticsData"=w649:T2, "error out"=w662:errorcluster)  [unwired: 11 in]
                        n173 = local write "Phase statistics"(w649) -> ()
                        n174 = local write "Zernike Measured"(w643) -> ()
                        n175 = call <userlib>:"LVClasse_Phase Get Data.vi"("Phase in"=w664, "Pupil"=w658, "error in (no error)"=w662) -> ("Phase out"=w660:refnum<class "Phase.lvclass">, "data"=w650:sgl[][], "Pupil (dup)"=w661:refnum<class "Pupil.lvclass">, "error out"=w663:errorcluster)  [unwired: 9 in]
                        n176 = local write "Phase values"(w650) -> ()
                      }
                      frame Error {
                      }
                    }
                  }
                  frame Error {
                  }
                }
              }
            }
          }
        }
        n177 = case shown="Error" w375 {
          tunnel: [w401 w404] -> w376
          tunnel: w375 -> [w401 w403]
          frame No Error {
          }
          frame Error {
            n178 = local write "Current status"("Running Error") -> ()
            n179 = call <vilib>:"Clear Errors.vi"("error in (no error)"=w403) -> ("error out"=w404:errorcluster)  [unwired: 5 in, 1 out]
            "Current error" <- w403
          }
        }
      }
      event "nb_images (set)": Value Change {
        # "SET IMAGE NUMBER"
        n180 = event-data() -> ("NewVal"=w705:u32)  [unwired: 1 in]
        n181 = call <userlib>:"LVClass_Camera set nbImagesToSum.vi"("Camera in"=w703, "nb_image"=w705, "error in (no error)"=w704) -> ("Camera out"=w700:refnum<class "Camera.lvclass">, "error out"=w699:errorcluster)  [unwired: 11 in]
        n182 = call <userlib>:"LVClass_Camera get nbImagesToSum.vi"("Camera in"=w700, "error in (no error)"=w699) -> ("Camera out"=w701:refnum<class "Camera.lvclass">, "nb_image"=→"nb_images (get)":u32, "error out"=w702:errorcluster)  [unwired: 11 in]
      }
      event "Coef Min": Value Change {
        # "Set coeff display scale: min"
        n183 = event-data() -> ()  [unwired: 1 in, 1 out]
        n184 = local read "Coef Min"() -> (w706:dbl)
        n185 = property on="Zernike Measured" class="WFGraph (strict)"("YScale.Minimum"=w706) -> ()  [unwired: 2 in, 2 out]
      }
      event "Coef Max": Value Change {
        # "Set coeff display scale: min"
        n186 = event-data() -> ()  [unwired: 1 in, 1 out]
        n187 = local read "Coef Max"() -> (w719:dbl)
        n188 = property on="Zernike Measured" class="WFGraph (strict)"("YScale.Maximum"=w719) -> ()  [unwired: 2 in, 2 out]
      }
      event "Reset error": Mouse Up {
        n189 = event-data() -> ()  [unwired: 1 in, 8 out]
        n190 = Select(t=w739, s=w739, f=errorcluster {"status"=FALSE, "code"=0, "source"=""} ("error out")) -> (s? t:f=w732:errorcluster)
        n191 = local write "Current error"(w732) -> ()
        n192 = local write "Current status"("Error cleared") -> ()
      }
      event "exposure_duration_s (set)": Value Change {
        # "CHANGE EXPOSURE DURATION"
        n193 = event-data() -> ()  [unwired: 1 in, 1 out]
        n194 = Multiply(x=1000000.0, y="exposure_duration_s (set)") -> (x*y=w754:dbl)
        n195 = To Unsigned Long Integer(number=w754) -> (unsigned 32bit integer=w753:u32)
        n196 = call <userlib>:"LVClass_Camera set Parameter Int.vi"("Camera in"=w767, "parameter_name"="exposure_duration_us", "value"=w753, "error in (no error)"=w768) -> ("Camera out"=w766:refnum<class "Camera.lvclass">, "error out"=w765:errorcluster)  [unwired: 10 in]
        n197 = call <userlib>:"LVClass_Camera get Parameter Int.vi"("Camera in"=w766, "parameter_name"="exposure_duration_us", "error in (no error)"=w765) -> ("Camera out"=w764:refnum<class "Camera.lvclass">, "value"=→"exposure_duration_us (get)":i32, "error out"=w763:errorcluster)  [unwired: 10 in]
      }
      event "Start HASO": Mouse Up {
        # "Start acquisition in SYNCRHONOUS mode\n\nonly one acquisition mode is available :\nLast image"
        n198 = event-data() -> ()  [unwired: 1 in, 8 out]
        n199 = flat-sequence {
          tunnel: w785 -> [w791]
          tunnel: w784 -> [w790]
          tunnel: [w789] -> w772
          tunnel: [w788] -> w771
          tunnel: [w793] -> w782
          tunnel: [w794] -> w783
          tunnel: w772 -> [w794]
          tunnel: w771 -> [w793]
          frame #0 {
            n200 = call <userlib>:"LVClass_Camera start acquisition.vi"("Camera in"=w791, "synchronisation_mode"=enum16{"synchronous", "asynchronous"}."asynchronous", "acquisition_mode"=enum16{"last_image", "new_image"}."last_image", "error in (no error)"=w790) -> ("Camera out"=w789:refnum<class "Camera.lvclass">, "error out"=w788:errorcluster)  [unwired: 10 in]
          }
          frame #1 {
            n201 = local write "HASO ready"(TRUE) -> ()
          }
        }
      }
      event "Stop HASO": Mouse Up {
        n202 = event-data() -> ()  [unwired: 1 in, 8 out]
        n203 = flat-sequence {
          tunnel: w808 -> [w812]
          tunnel: w795 -> [w810]
          tunnel: [w813] -> w798
          tunnel: [w811] -> w797
          tunnel: [w816] -> w809
          tunnel: w798 -> [w816]
          tunnel: w797 -> [w814]
          frame #0 {
            n204 = call <userlib>:"LVClass_Camera stop acquisition.vi"("Camera in"=w812, "error in (no error)"=w810) -> ("Camera out"=w813:refnum<class "Camera.lvclass">, "error out"=w811:errorcluster)  [unwired: 12 in]
          }
          frame #1 {
            n205 = local write "Current error"(w814) -> ()
            n206 = local write "HASO ready"(FALSE) -> ()
          }
        }
      }
      event "Update DM": Mouse Up {
        n207 = event-data() -> ()  [unwired: 1 in, 8 out]
        n208 = local read "Initial offset"() -> (w826:bool)
        n209 = case shown="True" w826 {
          tunnel: [w840 w845] -> w830
          frame False {
            n210 = Initialize Array(0.0, 52) -> (w840:dbl[])
          }
          frame True {
            n211 = local read "Offset command file"() -> (w844:path)
            n212 = call-poly <vilib>:"Read From Spreadsheet File.vi"("format (%.3f)"="%.8f", "file path (dialog if empty)"=w844) -> ("first row"=w845:dbl[])  [unwired: 5 in, 4 out]
          }
        }
        n213 = local read "Additional Command"() -> (w835:bool)
        n214 = case shown="True" w835 {
          tunnel: [w847 w853] -> w831
          tunnel: [w846 w852] -> w832
          tunnel: w829 -> [w846 w851]
          frame False {
            n215 = Initialize Array(0.0, 52) -> (w847:dbl[])
          }
          frame True {
            n216 = local read "Input type"() -> (w850:T8)
            n217 = case shown="\"DM actuators\"" w850 {
              tunnel: w851 -> [w854 w859 w902 w916 w925]
              tunnel: [w855 w861 w903 w914 w927] -> w853
              tunnel: [w854 w858 w902 w913 w924] -> w852
              frame "Zero Input" {
                n218 = Initialize Array(0.0, 52) -> (w855:dbl[])
              }
              frame "DM actuators" {
                w865 = 1
                w866 = 52
                n219 = local read "Zern/DM index in"() -> (w862:i32[])
                n220 = local read "Zern/DM coef in"() -> (w860:sgl[])
                n221 = Array Size(array=w862) -> (size(s)=w870:i32)
                n222 = Initialize Array(0.0, w866) -> (w868:dbl[])
                n223 = call-poly <vilib>:"Ramp Pattern.vi"("start"=w865, "end"=w866, "delta"=w865) -> ("Ramp Pattern"=w867:dbl[])  [unwired: 6 in, 2 out]
                n224 = Less Or Equal?(x=w870, y=w866) -> (x <= y?=w869:bool)
                n225 = case shown="True" w869 {
                  tunnel: w870 -> [_ w881]
                  tunnel: w868 -> [w874 w880]
                  tunnel: [w874 w879] -> w861
                  tunnel: w862 -> [_ w878]
                  tunnel: w860 -> [_ w877]
                  tunnel: [w871 w875] -> w858
                  tunnel: w866 -> [_ w876]
                  tunnel: w859 -> [w873 w875]
                  frame False {
                    n226 = Merge Errors(w873, errorcluster {"status"=FALSE, "code"=0, "source"="Wrong Zern index size"} ("error out")) -> (w871:errorcluster)
                  }
                  frame True {
                    n227 = for {
                      N: w881 -> [_]
                      shift-right: [w894] -> w879
                      shift-left: w880 -> [w895]
                      tunnel: w878 -> [w891] mode=indexing
                      tunnel: w877 -> [w885] mode=indexing
                      tunnel: w876 -> [w892]
                      n228 = Greater Than 0?(x=w891) -> (x > 0?=w890:bool)
                      n229 = Less Or Equal?(x=w891, y=w892) -> (x <= y?=w882:bool)
                      n230 = And(x=w890, y=w882) -> (x .and. y?=w889:bool)
                      n231 = In Range and Coerce(upper limit=0.8, x=w885, lower limit=-0.8) -> (coerced(x)=w886:dbl, In Range?=w888:bool)
                      n232 = And(x=w889, y=w888) -> (x .and. y?=w887:bool)
                      n233 = Decrement(x=w891) -> (x-1=w893:i32)
                      n234 = case shown="True" w887 {
                        tunnel: w893 -> [_ w900]
                        tunnel: w895 -> [w896 w899]
                        tunnel: [w896 w898] -> w894
                        tunnel: w886 -> [_ w897]
                        frame False {
                        }
                        frame True {
                          n235 = Replace Array Subset(array=w899, new element=w897, index=w900) -> (w898:dbl[])
                        }
                      }
                    }
                  }
                }
                n236 = local write "Coef out"(w861) -> ()
                n237 = To Long Integer(number=w867) -> (32bit integer=w863:i32[])
                n238 = local write "Index out"(w863) -> ()
              }
              frame "Command File" {
                n239 = local read "Additional file"() -> (w901:path)
                n240 = call-poly <vilib>:"Read From Spreadsheet File.vi"("format (%.3f)"="%.8f", "file path (dialog if empty)"=w901) -> ("first row"=w903:dbl[])  [unwired: 5 in, 4 out]
              }
              frame "Zernike Coef", Default {
                n241 = local read "Zern/DM index in"() -> (w905:i32[])
                n242 = local read "Zern/DM coef in"() -> (w906:sgl[])
                n243 = local read "idxType"() -> (w912:enum16{"Wyant", "ANSI"})
                n244 = local read "Initial haso file"() -> (w910:path)
                n245 = local read "Haso configuration file"() -> (w911:path)
                n246 = local read "interaction matrix file"() -> (w909:path)
                n247 = call "zern2command.vi"("Haso configuration file"=w911, "idxType"=w912, "interaction matrix file"=w909, "error in (no error)"=w916, "Zern coef in"=w906, "Zern index in"=w905, "Initial haso file"=w910) -> ("error out"=w915:errorcluster, "Offset Positions"=w914:sgl[], "Zern pupil out"=w917:refnum<class "Pupil.lvclass">, "ModalCoef out"=w918:refnum<class "ModalCoef.lvclass">)  [unwired: 1 in]
                n248 = call <userlib>:"LVClass_ModalCoef GetData.vi"("ModalCoef in"=w918, "Pupil.lvclass"=w917, "error in (no error)"=w915) -> ("ModalCoef out"=w922:refnum<class "ModalCoef.lvclass">, "coef"=w908:sgl[], "index"=w907:u32[], "Pupil.lvclass (dup)"=w921:refnum<class "Pupil.lvclass">, "error out"=w920:errorcluster)  [unwired: 8 in]
                n249 = local write "Index out"(w907) -> ()
                n250 = call <userlib>:"LVClass_Pupil dtor.vi"("Pupil in"=w921, "error in (no error)"=w920) -> ("error out"=w919:errorcluster)  [unwired: 12 in, 1 out]
                n251 = local write "Coef out"(w908) -> ()
                n252 = call <userlib>:"LVClass_ModalCoef dtor.vi"("ModalCoef in"=w922, "error in (no error)"=w919) -> ("error out"=w913:errorcluster)  [unwired: 12 in, 1 out]
              }
              frame "Zernike File" {
                w930 = 1
                n253 = local read "interaction matrix file"() -> (w934:path)
                n254 = local read "Initial haso file"() -> (w932:path)
                n255 = local read "Haso configuration file"() -> (w933:path)
                n256 = local read "Additional file"() -> (w943:path)
                n257 = call-poly <vilib>:"Ramp Pattern.vi"("start"=w930, "end"=32, "delta"=w930) -> ("Ramp Pattern"=w931:dbl[])  [unwired: 6 in, 2 out]
                n258 = To Long Integer(number=w931) -> (32bit integer=w928:i32[])
                n259 = local read "idxType"() -> (w923:enum16{"Wyant", "ANSI"})
                n260 = call-poly <vilib>:"Read From Spreadsheet File.vi"("format (%.3f)"="%.8f", "file path (dialog if empty)"=w943) -> ("first row"=w935:dbl[])  [unwired: 5 in, 4 out]
                n261 = call "zern2command.vi"("Haso configuration file"=w933, "idxType"=w923, "interaction matrix file"=w934, "Zern coef in"=w935, "Zern index in"=w928, "Initial haso file"=w932) -> ("error out"=w936:errorcluster, "Offset Positions"=w927:sgl[], "Zern pupil out"=w937:refnum<class "Pupil.lvclass">, "ModalCoef out"=w938:refnum<class "ModalCoef.lvclass">)  [unwired: 2 in]
                n262 = call <userlib>:"LVClass_ModalCoef GetData.vi"("ModalCoef in"=w938, "Pupil.lvclass"=w937, "error in (no error)"=w936) -> ("ModalCoef out"=w942:refnum<class "ModalCoef.lvclass">, "Pupil.lvclass (dup)"=w941:refnum<class "Pupil.lvclass">, "error out"=w940:errorcluster)  [unwired: 8 in, 2 out]
                n263 = call <userlib>:"LVClass_Pupil dtor.vi"("Pupil in"=w941, "error in (no error)"=w940) -> ("error out"=w939:errorcluster)  [unwired: 12 in, 1 out]
                n264 = call <userlib>:"LVClass_ModalCoef dtor.vi"("ModalCoef in"=w942, "error in (no error)"=w939) -> ("error out"=w926:errorcluster)  [unwired: 12 in, 1 out]
                n265 = Merge Errors(w926, w925) -> (w924:errorcluster)
              }
            }
          }
        }
        n266 = local write "Initial Positions"(w830) -> ()
        n267 = Add(x=w831, y=w830) -> (x+y=w817:dbl[])
        n268 = call <userlib>:"LVClass_WavefrontCorrector Move to Absolute Position.vi"("WavefrontCorrector in"=w827, "Absolute Positions"=w817, "error in (no error)"=w832) -> ("WavefrontCorrector out"=w833:refnum<class "WavefrontCorrector.lvclass">, "error out"=w834:errorcluster)  [unwired: 11 in]
        n269 = call <userlib>:"LVClass_WavefrontCorrector Get Current Position.vi"("WavefrontCorrector in"=w833, "error in (no error)"=w834) -> ("WavefrontCorrector out"=w823:refnum<class "WavefrontCorrector.lvclass">, "Wavefront Corrector Position"=w818:T18, "error out"=w828:errorcluster)  [unwired: 11 in]
        n270 = local write "Final Positions"(w817) -> ()
        n271 = local write "DM Actuator Values"(w818) -> ()
      }
      event "Update AcqSetting": Mouse Up {
        n272 = event-data() -> ()  [unwired: 1 in, 8 out]
        n273 = local read "Gain On"() -> (w964:bool)
        n274 = local read "Aquisition Mode"() -> (w955:T6)
        n275 = local read "Accum Num"() -> (w954:u32)
        n276 = To Unsigned Word Integer(number=w955) -> (unsigned 16bit integer=w949:u16)
        n277 = local read "Kinetic Num"() -> (w966:u32)
        n278 = local read "Trigger Mode"() -> (w956:enum16{"Internal", "External"})
        n279 = call <userlib>:"SetAcquisitionMode.vi"("error in (no error)"=w948, "mode"=w949) -> ("error out"=w950:errorcluster)  [unwired: 1 out]
        n280 = To Unsigned Word Integer(number=w956) -> (unsigned 16bit integer=w951:u16)
        n281 = local read "Exposure time (s)"() -> (w957:dbl)
        n282 = call <userlib>:"SetTriggerMode.vi"("error in (no error)"=w950, "mode"=w951) -> ("error out"=w952:errorcluster)  [unwired: 1 out]
        n283 = call <userlib>:"SetExposureTime.vi"("error in (no error)"=w952, "time"=w957) -> ("error out"=w953:errorcluster)  [unwired: 1 out]
        n284 = case shown="\"None\", Default" w955 {
          tunnel: w954 -> [_ _ w984 w989]
          tunnel: w953 -> [w980 w981 w983 w988]
          tunnel: [w980 w981 w982 w986] -> w967
          tunnel: w966 -> [_ _ _ w985]
          frame "None", Default {
          }
          frame "Single Scan" {
          }
          frame "Accumulate" {
            n285 = call <userlib>:"SetNumberAccumulations.vi"("error in (no error)"=w983, "number"=w984) -> ("error out"=w982:errorcluster)  [unwired: 1 out]
          }
          frame "Kinetics" {
            n286 = call <userlib>:"SetNumberAccumulations.vi"("error in (no error)"=w988, "number"=w989) -> ("error out"=w987:errorcluster)  [unwired: 1 out]
            n287 = call <userlib>:"SetNumberKinetics.vi"("error in (no error)"=w987, "number"=w985) -> ("error out"=w986:errorcluster)  [unwired: 1 out]
          }
        }
        n288 = case shown="False" w964 {
          tunnel: w967 -> [w973 w979]
          tunnel: [w972 w976] -> w965
          frame False {
            n289 = call <userlib>:"SetEMCCDGain.vi"("error in (no error)"=w973, "gain"=0) -> ("error out"=w972:errorcluster)  [unwired: 1 out]
          }
          frame True {
            # "0-255"
            n290 = call <userlib>:"SetEMGainMode.vi"("error in (no error)"=w979, "mode"=0) -> ("error out"=w977:errorcluster)  [unwired: 1 out]
            n291 = local read "Gain Value"() -> (w975:sgl)
            n292 = call <userlib>:"SetEMCCDGain.vi"("error in (no error)"=w977, "gain"=w975) -> ("error out"=w976:errorcluster)  [unwired: 1 out]
          }
        }
        n293 = call <userlib>:"GetEMCCDGain.vi"("error in (no error)"=w965) -> ("error out"=w962:errorcluster, "gain"=w963:u32)  [unwired: 2 in, 1 out]
        n294 = local write "Get EMCCD Gain"(w963) -> ()
        n295 = call <userlib>:"GetAcquisitionTimings.vi"("error in (no error)"=w962) -> ("exposure"=w958:sgl, "accumulate"=w960:sgl, "kinetic"=w961:sgl, "DLL error code"=w959:u32, "error out"=w947:errorcluster)  [unwired: 10 in]
        n296 = local write "Return from CheckTimings"(w959) -> ()
        n297 = local write "Get Exposure Time"(w958) -> ()
        n298 = local write "Get Kinetic Time"(w961) -> ()
        n299 = local write "Get Accum Time"(w960) -> ()
      }
      event "Update FOV": Mouse Up {
        n300 = event-data() -> ()  [unwired: 1 in, 8 out]
        n301 = local read "Detector Y Pixels"() -> (w992:i32)
        n302 = local read "Detector X Pixels"() -> (w1011:i32)
        n303 = local read "Camera FOV"() -> (w1010:T5)
        n304 = case shown="\"Custom FOV\"" w1010 {
          tunnel: [w1023 w1047 w1063 w1079 w1095 w1098] -> w996
          tunnel: [w1022 w1047 w1063 w1079 w1095 w1098] -> w995
          tunnel: [w1021 w1037 w1053 w1069 w1085 w1098] -> w994
          tunnel: [w1020 w1034 w1050 w1066 w1082 w1096] -> w993
          tunnel: [w1018 w1036 w1052 w1068 w1084 w1098] -> w997
          tunnel: [w1019 w1033 w1049 w1065 w1081 w1097] -> w998
          tunnel: w1011 -> [_ w1046 w1062 w1078 w1094 w1096]
          tunnel: w992 -> [_ w1045 w1061 w1077 w1093 w1097]
          tunnel: [w1024 w1032 w1048 w1064 w1080 w1097] -> w1000
          tunnel: [w1026 w1032 w1048 w1064 w1080 w1096] -> w999
          frame "Custom FOV" {
            n305 = local read "Xstart"() -> (w1021:i32)
            n306 = local read "Xend"() -> (w1020:i32)
            n307 = local read "Xstart"() -> (w1018:i32)
            n308 = local read "Yend"() -> (w1019:i32)
            n309 = Subtract(x=w1019, y=w1018) -> (x-y=w1030:i32)
            n310 = Subtract(x=w1020, y=w1021) -> (x-y=w1031:i32)
            n311 = local read "Xbin"() -> (w1023:i32)
            n312 = local read "Ybin"() -> (w1022:i32)
            n313 = Increment(x=w1030) -> (x+1=w1029:i32)
            n314 = Increment(x=w1031) -> (x+1=w1028:i32)
            n315 = Divide(x=w1029, y=w1022) -> (x/y=w1025:dbl)
            n316 = Divide(x=w1028, y=w1023) -> (x/y=w1027:dbl)
            n317 = To Long Integer(number=w1025) -> (32bit integer=w1024:i32)
            n318 = To Long Integer(number=w1027) -> (32bit integer=w1026:i32)
          }
          frame "FOV: 768x768" {
            w1032 = 768
            w1042 = 2.0
            w1047 = 1
            n319 = Subtract(x=w1046, y=w1032) -> (x-y=w1044:i32)
            n320 = Subtract(x=w1045, y=w1032) -> (x-y=w1043:i32)
            n321 = Divide(x=w1043, y=w1042) -> (x/y=w1040:dbl)
            n322 = Divide(x=w1044, y=w1042) -> (x/y=w1041:dbl)
            n323 = Decrement(x=w1032) -> (x-1=w1035:i32)
            n324 = Round To Nearest(number=w1041) -> (nearest integer value=w1039:dbl)
            n325 = Round To Nearest(number=w1040) -> (nearest integer value=w1038:dbl)
            n326 = To Long Integer(number=w1039) -> (32bit integer=w1037:i32)
            n327 = To Long Integer(number=w1038) -> (32bit integer=w1036:i32)
            n328 = Add(x=w1035, y=w1037) -> (x+y=w1034:i32)
            n329 = Add(x=w1035, y=w1036) -> (x+y=w1033:i32)
          }
          frame "FOV: 512x512" {
            w1048 = 512
            w1058 = 2.0
            w1063 = 1
            n330 = Subtract(x=w1062, y=w1048) -> (x-y=w1060:i32)
            n331 = Subtract(x=w1061, y=w1048) -> (x-y=w1059:i32)
            n332 = Divide(x=w1059, y=w1058) -> (x/y=w1056:dbl)
            n333 = Divide(x=w1060, y=w1058) -> (x/y=w1057:dbl)
            n334 = Decrement(x=w1048) -> (x-1=w1051:i32)
            n335 = Round To Nearest(number=w1057) -> (nearest integer value=w1055:dbl)
            n336 = Round To Nearest(number=w1056) -> (nearest integer value=w1054:dbl)
            n337 = To Long Integer(number=w1055) -> (32bit integer=w1053:i32)
            n338 = To Long Integer(number=w1054) -> (32bit integer=w1052:i32)
            n339 = Add(x=w1051, y=w1053) -> (x+y=w1050:i32)
            n340 = Add(x=w1051, y=w1052) -> (x+y=w1049:i32)
          }
          frame "FOV: 320x320" {
            w1064 = 320
            w1074 = 2.0
            w1079 = 1
            n341 = Subtract(x=w1078, y=w1064) -> (x-y=w1076:i32)
            n342 = Subtract(x=w1077, y=w1064) -> (x-y=w1075:i32)
            n343 = Divide(x=w1075, y=w1074) -> (x/y=w1072:dbl)
            n344 = Divide(x=w1076, y=w1074) -> (x/y=w1073:dbl)
            n345 = Decrement(x=w1064) -> (x-1=w1067:i32)
            n346 = Round To Nearest(number=w1073) -> (nearest integer value=w1071:dbl)
            n347 = Round To Nearest(number=w1072) -> (nearest integer value=w1070:dbl)
            n348 = To Long Integer(number=w1071) -> (32bit integer=w1069:i32)
            n349 = To Long Integer(number=w1070) -> (32bit integer=w1068:i32)
            n350 = Add(x=w1067, y=w1069) -> (x+y=w1066:i32)
            n351 = Add(x=w1067, y=w1068) -> (x+y=w1065:i32)
          }
          frame "FOV: 256x256" {
            w1080 = 256
            w1090 = 2.0
            w1095 = 1
            n352 = Subtract(x=w1094, y=w1080) -> (x-y=w1092:i32)
            n353 = Subtract(x=w1093, y=w1080) -> (x-y=w1091:i32)
            n354 = Divide(x=w1091, y=w1090) -> (x/y=w1088:dbl)
            n355 = Divide(x=w1092, y=w1090) -> (x/y=w1089:dbl)
            n356 = Decrement(x=w1080) -> (x-1=w1083:i32)
            n357 = Round To Nearest(number=w1089) -> (nearest integer value=w1087:dbl)
            n358 = Round To Nearest(number=w1088) -> (nearest integer value=w1086:dbl)
            n359 = To Long Integer(number=w1087) -> (32bit integer=w1085:i32)
            n360 = To Long Integer(number=w1086) -> (32bit integer=w1084:i32)
            n361 = Add(x=w1083, y=w1085) -> (x+y=w1082:i32)
            n362 = Add(x=w1083, y=w1084) -> (x+y=w1081:i32)
          }
          frame "Full FOV", Default {
            w1098 = 1
          }
        }
        n363 = local write "FOV X Pixels"(w999) -> ()
        n364 = local write "FOV Y Pixels"(w1000) -> ()
        n365 = call <userlib>:"SetImage.vi"("hbin"=w996, "vbin"=w995, "hstart"=w994, "hend"=w993, "vstart"=w997, "vend"=w998, "error in (no error)"=w990) -> ("error out"=w1001:errorcluster)  [unwired: 19 in, 1 out]
        n366 = call <userlib>:"GetAcquisitionTimings.vi"("error in (no error)"=w1001) -> ("exposure"=w1003:sgl, "accumulate"=w1004:sgl, "kinetic"=w1005:sgl, "DLL error code"=w1006:u32, "error out"=w1002:errorcluster)  [unwired: 10 in]
        n367 = call <userlib>:"GetAcquisitionProgress.vi"("error in (no error)"=w1002) -> ("error out"=w991:errorcluster, "DLL error code"=w1009:u32, "series"=w1008:i32, "accum"=w1007:i32)  [unwired: 3 in]
        n368 = local write "Get Exposure Time"(w1003) -> ()
        n369 = local write "Get Accum Time"(w1004) -> ()
        n370 = local write "Get Kinetic Time"(w1005) -> ()
        n371 = local write "Return from CheckTimings"(w1006) -> ()
        n372 = local write "Return from CheckProcess"(w1009) -> ()
        n373 = local write "Get Kinetic Num"(w1007) -> ()
        n374 = local write "Get Kinetic Num"(w1008) -> ()
      }
      event "Live EMCCD": Value Change {
        # "Set Acquisition Mode: Single Scan or original"
        n375 = event-data() -> ()  [unwired: 1 in, 6 out]
        n376 = case shown="True" "Live EMCCD" {
          tunnel: [0 w1114] -> w1106
          tunnel: [w1112 w1114] -> w1099
          frame False {
            n377 = local read "Aquisition Mode"() -> (w1112:T6)
          }
          frame True {
            w1114 = 1
          }
        }
        n378 = flat-sequence {
          tunnel: w1103 -> [w1116]
          tunnel: [w1116] -> w1107
          tunnel: w1106 -> [w1115]
          tunnel: w1107 -> [w1120]
          tunnel: [w1119] -> w1105
          tunnel: w1099 -> [w1117]
          tunnel: [w1122] -> w1102
          tunnel: w1105 -> [w1122]
          tunnel: "Live EMCCD" -> [w1121]
          frame #0 {
            n379 = local write "Running Status"(w1115) -> ()
          }
          frame #1 {
            n380 = To Unsigned Word Integer(number=w1117) -> (unsigned 16bit integer=w1118:u16)
            n381 = call <userlib>:"SetAcquisitionMode.vi"("error in (no error)"=w1120, "mode"=w1118) -> ("error out"=w1119:errorcluster)  [unwired: 1 out]
          }
          frame #2 {
            n382 = local write "EMCCD Status"(w1121) -> ()
          }
        }
      }
      event "Snap": Mouse Up {
        n383 = event-data() -> ()  [unwired: 1 in, 8 out]
        n384 = local write "Running Status"(2) -> ()
      }
      event "Acquire": Mouse Up {
        n385 = event-data() -> ()  [unwired: 1 in, 8 out]
        n386 = local write "Running Status"(3) -> ()
      }
      event "Abort": Mouse Up {
        n387 = event-data() -> ()  [unwired: 1 in, 8 out]
        n388 = local write "Running Status"(0) -> ()
      }
      event "Intensity Min": Value Change {
        n389 = event-data() -> ()  [unwired: 1 in, 6 out]
        n390 = property on="Intensity Graph" class="IntGraph (strict)"("ZScale.Minimum"="Intensity Min") -> ()  [unwired: 2 in, 2 out]
      }
      event "Intensity Max": Value Change {
        n391 = event-data() -> ()  [unwired: 1 in, 6 out]
        n392 = property on="Intensity Graph" class="IntGraph (strict)"("ZScale.Maximum"="Intensity Max") -> ()  [unwired: 2 in, 2 out]
      }
      event "Auto Scale": Value Change {
        n393 = event-data() -> ()  [unwired: 1 in, 6 out]
        n394 = property on="Intensity Graph" class="IntGraph (strict)"("ZScale.LooseFit"="Auto Scale") -> ()  [unwired: 2 in, 2 out]
      }
      event "left": Mouse Up {
        n395 = event-data() -> ()  [unwired: 1 in, 8 out]
        n396 = local read "XY step"() -> (w1171:dbl)
        n397 = Number To Fractional String(number=w1171, precision (6)=1) -> (F-format string=w1177:string)  [unwired: 2 in]
        n398 = Concatenate Strings("movrel y=-", w1177) -> (w1179:string)
        n399 = call "WriteCmd.vi"("error IO"=w1173, "Command"=w1179, "VISA resource name"=w1175) -> ("error"=w1172:errorcluster)  [unwired: 1 out]
      }
      event "right": Mouse Up {
        n400 = event-data() -> ()  [unwired: 1 in, 8 out]
        n401 = local read "XY step"() -> (w1185:dbl)
        n402 = Number To Fractional String(number=w1185, precision (6)=1) -> (F-format string=w1191:string)  [unwired: 2 in]
        n403 = Concatenate Strings("movrel y=", w1191) -> (w1193:string)
        n404 = call "WriteCmd.vi"("error IO"=w1187, "Command"=w1193, "VISA resource name"=w1189) -> ("error"=w1186:errorcluster)  [unwired: 1 out]
      }
      event "front": Mouse Up {
        n405 = event-data() -> ()  [unwired: 1 in, 8 out]
        n406 = local read "XY step"() -> (w1199:dbl)
        n407 = Number To Fractional String(number=w1199, precision (6)=1) -> (F-format string=w1205:string)  [unwired: 2 in]
        n408 = Concatenate Strings("movrel x=-", w1205) -> (w1207:string)
        n409 = call "WriteCmd.vi"("error IO"=w1201, "Command"=w1207, "VISA resource name"=w1203) -> ("error"=w1200:errorcluster)  [unwired: 1 out]
      }
      event "back": Mouse Up {
        n410 = event-data() -> ()  [unwired: 1 in, 8 out]
        n411 = local read "XY step"() -> (w1213:dbl)
        n412 = Number To Fractional String(number=w1213, precision (6)=1) -> (F-format string=w1219:string)  [unwired: 2 in]
        n413 = Concatenate Strings("movrel x=", w1219) -> (w1221:string)
        n414 = call "WriteCmd.vi"("error IO"=w1215, "Command"=w1221, "VISA resource name"=w1217) -> ("error"=w1214:errorcluster)  [unwired: 1 out]
      }
      event "up": Mouse Up {
        n415 = event-data() -> ()  [unwired: 1 in, 8 out]
        n416 = local read "Z step"() -> (w1227:dbl)
        n417 = Number To Fractional String(number=w1227, precision (6)=1) -> (F-format string=w1233:string)  [unwired: 2 in]
        n418 = Concatenate Strings("movrel z=", w1233) -> (w1235:string)
        n419 = call "WriteCmd.vi"("error IO"=w1229, "Command"=w1235, "VISA resource name"=w1231) -> ("error"=w1228:errorcluster)  [unwired: 1 out]
      }
      event "down": Mouse Up {
        n420 = event-data() -> ()  [unwired: 1 in, 8 out]
        n421 = local read "Z step"() -> (w1241:dbl)
        n422 = Number To Fractional String(number=w1241, precision (6)=1) -> (F-format string=w1247:string)  [unwired: 2 in]
        n423 = Concatenate Strings("movrel z=-", w1247) -> (w1249:string)
        n424 = call "WriteCmd.vi"("error IO"=w1243, "Command"=w1249, "VISA resource name"=w1245) -> ("error"=w1242:errorcluster)  [unwired: 1 out]
      }
      event "flip mirror button": Mouse Up {
        w1257 = tag "Dev1/ao5" ("physical channels")
        n425 = event-data() -> ()  [unwired: 1 in, 8 out]
        n426 = flat-sequence {
          tunnel: [w1271] -> w1261
          tunnel: w1257 -> [w1269]
          tunnel: w1256 -> [w1268]
          tunnel: [w1272] -> w1260
          tunnel: w1261 -> [w1272]
          tunnel: w1260 -> [w1276]
          tunnel: [w1275] -> w1259
          tunnel: w1257 -> [w1274]
          tunnel: [w1278] -> w1258
          tunnel: w1259 -> [w1278]
          tunnel: w1258 -> [w1282]
          tunnel: w1257 -> [w1281]
          tunnel: [w1280] -> w1255
          frame #0 {
            n427 = call "AO single value.vi"("error in"=w1268, "data"=0.0, "physical channels"=w1269) -> ("error out"=w1271:errorcluster)
          }
          frame #1 {
            n428 = Wait (ms)(milliseconds to wait=u32 100) -> ()  [unwired: 1 out]
          }
          frame #2 {
            n429 = call "AO single value.vi"("error in"=w1276, "data"=5.0, "physical channels"=w1274) -> ("error out"=w1275:errorcluster)
          }
          frame #3 {
            n430 = Wait (ms)(milliseconds to wait=u32 100) -> ()  [unwired: 1 out]
          }
          frame #4 {
            n431 = call "AO single value.vi"("error in"=w1282, "data"=0.0, "physical channels"=w1281) -> ("error out"=w1280:errorcluster)
          }
        }
      }
      event "Send": Mouse Up {
        n432 = event-data() -> ()  [unwired: 1 in, 8 out]
        n433 = call "WriteCmd.vi"("error IO"=w1286, "Command"="Command", "VISA resource name"=w1284) -> ("error"=w1288:errorcluster)  [unwired: 1 out]
        n434 = VISA Read(VISA resource name=w1284, byte count=u32 4096, error in (no error)=w1288) -> (read buffer=→"Response:":string, error out=w1285:errorcluster)  [unwired: 2 out]
      }
      event "Get Position": Mouse Up {
        n435 = event-data() -> ()  [unwired: 1 in, 8 out]
        n436 = call "Get Current Position.vi"("error in (no error)"=w1299, "Array of axes"="Axis", "VISA in"=w1297) -> ("error out"=w1298:errorcluster, "Array of positions [internal units]"=w1301:dbl[])  [unwired: 6 in, 1 out]
        n437 = Multiply(x=w1301, y=0.1) -> (x*y=→"Position (um)":dbl[])
      }
      event "Record Response": Mouse Up {
        n438 = event-data() -> ()  [unwired: 1 in, 8 out]
        n439 = local read "Net Rp"() -> (w1310:bool)
        n440 = stacked-sequence {
          seq-local: [_ _ _ w1682 _] -> [_ _ _ _ w1707]
          seq-local: [_ _ w1549 _ _] -> [_ _ _ w1681 _]
          seq-local: [_ w1344 _ _ _] -> [_ _ w1550 _ _]
          seq-local: [_ _ w1548 _ _] -> [_ _ _ _ w1703]
          tunnel: [_ _ _ _ w1706] -> w1328
          tunnel: w1327 -> [_ w1357 _ _ _]
          tunnel: [_ _ _ _ w1705] -> w1326
          tunnel: w1325 -> [_ w1356 _ w1683 _]
          tunnel: [_ w1354 _ _ _] -> w1323
          tunnel: w1322 -> [_ _ w1562 _ w1715]
          tunnel: w1321 -> [_ _ w1561 _ w1714]
          tunnel: w1320 -> [_ _ w1560 _ w1713]
          tunnel: w1319 -> [_ _ w1559 _ w1712]
          tunnel: w1318 -> [_ _ w1558 _ w1711]
          tunnel: w1317 -> [_ _ w1557 _ _]
          tunnel: w1316 -> [_ _ w1556 _ w1710]
          tunnel: w1312 -> [_ _ w1555 _ w1709]
          tunnel: w1315 -> [_ _ w1554 _ w1708]
          tunnel: [_ _ _ _ w1702] -> w1314
          tunnel: [_ _ w1552 _ _] -> w1313
          tunnel: [_ _ w1551 _ _] -> w1311
          tunnel: w1310 -> [_ _ _ w1680 w1704]
          frame #0 {
            # "Create output folder path"
            n441 = local read "Base Path"() -> (w1329:path)
            n442 = local read "Subfolder"() -> (w1332:string)
            n443 = local write "Current status"("Check single response") -> ()
            n444 = Build Path(base path=w1329, name or relative path=w1332) -> (appended path=w1331:path)
            n445 = call <vilib>:"Check if File or Folder Exists.vi"("path"=w1331) -> ("error out"=w1333:errorcluster, "file or folder exists?"=w1334:bool)  [unwired: 8 in, 1 out]
            n446 = case shown="True" w1334 {
              tunnel: w1331 -> [w1337 w1342]
              tunnel: w1333 -> [w1336 w1343]
              tunnel: [w1335 w1338] -> _
              frame False {
                n447 = Create Folder(path (use dialog)=w1337, error in=w1336) -> (error out=w1335:errorcluster)  [unwired: 1 in, 2 out]
              }
              frame True {
                n448 = Delete(path (use dialog)=w1342, entire hierarchy (F)=TRUE, error in=w1343) -> (deleted path=w1340:path, error out=w1339:errorcluster)  [unwired: 2 in, 1 out]
                n449 = Create Folder(path (use dialog)=w1340, error in=w1339) -> (error out=w1338:errorcluster)  [unwired: 1 in, 2 out]
              }
            }
            n450 = local write "AO output"(w1331) -> ()
          }
          frame #1 {
            # "Delay for DM response"
            # "Apply command to DM"
            n451 = local read "Initial offset"() -> (w1355:bool)
            n452 = case shown="True" w1355 {
              tunnel: [w1443 w1448] -> w1346
              frame False {
                n453 = Initialize Array(0.0, 52) -> (w1443:dbl[])
              }
              frame True {
                n454 = local read "Offset command file"() -> (w1447:path)
                n455 = call-poly <vilib>:"Read From Spreadsheet File.vi"("format (%.3f)"="%.8f", "file path (dialog if empty)"=w1447) -> ("first row"=w1448:dbl[])  [unwired: 5 in, 4 out]
              }
            }
            n456 = local read "Additional Command"() -> (w1361:bool)
            n457 = case shown="True" w1361 {
              tunnel: [w1450 w1456] -> w1347
              tunnel: [w1449 w1455] -> w1358
              tunnel: w1357 -> [w1449 w1454]
              frame False {
                n458 = Initialize Array(0.0, 52) -> (w1450:dbl[])
              }
              frame True {
                n459 = local read "Input type"() -> (w1453:T8)
                n460 = case shown="\"DM actuators\"" w1453 {
                  tunnel: w1454 -> [w1457 w1463 w1505 w1519 w1528]
                  tunnel: [w1458 w1461 w1506 w1517 w1530] -> w1456
                  tunnel: [w1457 w1462 w1505 w1516 w1527] -> w1455
                  frame "Zero Input" {
                    n461 = Initialize Array(0.0, 52) -> (w1458:dbl[])
                  }
                  frame "DM actuators" {
                    w1465 = 1
                    w1466 = 52
                    n462 = local read "Zern/DM index in"() -> (w1472:i32[])
                    n463 = local read "Zern/DM coef in"() -> (w1473:sgl[])
                    n464 = Array Size(array=w1472) -> (size(s)=w1467:i32)
                    n465 = Initialize Array(0.0, w1466) -> (w1469:dbl[])
                    n466 = call-poly <vilib>:"Ramp Pattern.vi"("start"=w1465, "end"=w1466, "delta"=w1465) -> ("Ramp Pattern"=w1470:dbl[])  [unwired: 6 in, 2 out]
                    n467 = Less Or Equal?(x=w1467, y=w1466) -> (x <= y?=w1468:bool)
                    n468 = case shown="True" w1468 {
                      tunnel: w1467 -> [_ w1484]
                      tunnel: w1469 -> [w1477 w1483]
                      tunnel: [w1477 w1482] -> w1461
                      tunnel: w1472 -> [_ w1481]
                      tunnel: w1473 -> [_ w1480]
                      tunnel: [w1474 w1478] -> w1462
                      tunnel: w1466 -> [_ w1479]
                      tunnel: w1463 -> [w1476 w1478]
                      frame False {
                        n469 = Merge Errors(w1476, errorcluster {"status"=FALSE, "code"=0, "source"="Wrong Zern index size"} ("error out")) -> (w1474:errorcluster)
                      }
                      frame True {
                        n470 = for {
                          N: w1484 -> [_]
                          shift-right: [w1497] -> w1482
                          shift-left: w1483 -> [w1498]
                          tunnel: w1481 -> [w1494] mode=indexing
                          tunnel: w1480 -> [w1488] mode=indexing
                          tunnel: w1479 -> [w1495]
                          n471 = Greater Than 0?(x=w1494) -> (x > 0?=w1493:bool)
                          n472 = Less Or Equal?(x=w1494, y=w1495) -> (x <= y?=w1485:bool)
                          n473 = And(x=w1493, y=w1485) -> (x .and. y?=w1492:bool)
                          n474 = In Range and Coerce(upper limit=0.8, x=w1488, lower limit=-0.8) -> (coerced(x)=w1489:dbl, In Range?=w1491:bool)
                          n475 = And(x=w1492, y=w1491) -> (x .and. y?=w1490:bool)
                          n476 = Decrement(x=w1494) -> (x-1=w1496:i32)
                          n477 = case shown="True" w1490 {
                            tunnel: w1496 -> [_ w1503]
                            tunnel: w1498 -> [w1499 w1502]
                            tunnel: [w1499 w1501] -> w1497
                            tunnel: w1489 -> [_ w1500]
                            frame False {
                            }
                            frame True {
                              n478 = Replace Array Subset(array=w1502, new element=w1500, index=w1503) -> (w1501:dbl[])
                            }
                          }
                        }
                      }
                    }
                    n479 = local write "Coef out"(w1461) -> ()
                    n480 = To Long Integer(number=w1470) -> (32bit integer=w1471:i32[])
                    n481 = local write "Index out"(w1471) -> ()
                  }
                  frame "Command File" {
                    n482 = local read "Additional file"() -> (w1504:path)
                    n483 = call-poly <vilib>:"Read From Spreadsheet File.vi"("format (%.3f)"="%.8f", "file path (dialog if empty)"=w1504) -> ("first row"=w1506:dbl[])  [unwired: 5 in, 4 out]
                  }
                  frame "Zernike Coef", Default {
                    n484 = local read "Zern/DM index in"() -> (w1508:i32[])
                    n485 = local read "Zern/DM coef in"() -> (w1509:sgl[])
                    n486 = local read "idxType"() -> (w1515:enum16{"Wyant", "ANSI"})
                    n487 = local read "Initial haso file"() -> (w1513:path)
                    n488 = local read "Haso configuration file"() -> (w1514:path)
                    n489 = local read "interaction matrix file"() -> (w1512:path)
                    n490 = call "zern2command.vi"("Haso configuration file"=w1514, "idxType"=w1515, "interaction matrix file"=w1512, "error in (no error)"=w1519, "Zern coef in"=w1509, "Zern index in"=w1508, "Initial haso file"=w1513) -> ("error out"=w1518:errorcluster, "Offset Positions"=w1517:sgl[], "Zern pupil out"=w1520:refnum<class "Pupil.lvclass">, "ModalCoef out"=w1521:refnum<class "ModalCoef.lvclass">)  [unwired: 1 in]
                    n491 = call <userlib>:"LVClass_ModalCoef GetData.vi"("ModalCoef in"=w1521, "Pupil.lvclass"=w1520, "error in (no error)"=w1518) -> ("ModalCoef out"=w1525:refnum<class "ModalCoef.lvclass">, "coef"=w1511:sgl[], "index"=w1510:u32[], "Pupil.lvclass (dup)"=w1524:refnum<class "Pupil.lvclass">, "error out"=w1523:errorcluster)  [unwired: 8 in]
                    n492 = local write "Index out"(w1510) -> ()
                    n493 = call <userlib>:"LVClass_Pupil dtor.vi"("Pupil in"=w1524, "error in (no error)"=w1523) -> ("error out"=w1522:errorcluster)  [unwired: 12 in, 1 out]
                    n494 = local write "Coef out"(w1511) -> ()
                    n495 = call <userlib>:"LVClass_ModalCoef dtor.vi"("ModalCoef in"=w1525, "error in (no error)"=w1522) -> ("error out"=w1516:errorcluster)  [unwired: 12 in, 1 out]
                  }
                  frame "Zernike File" {
                    w1533 = 1
                    n496 = local read "interaction matrix file"() -> (w1537:path)
                    n497 = local read "Initial haso file"() -> (w1535:path)
                    n498 = local read "Haso configuration file"() -> (w1536:path)
                    n499 = local read "Additional file"() -> (w1546:path)
                    n500 = call-poly <vilib>:"Ramp Pattern.vi"("start"=w1533, "end"=32, "delta"=w1533) -> ("Ramp Pattern"=w1534:dbl[])  [unwired: 6 in, 2 out]
                    n501 = To Long Integer(number=w1534) -> (32bit integer=w1531:i32[])
                    n502 = local read "idxType"() -> (w1526:enum16{"Wyant", "ANSI"})
                    n503 = call-poly <vilib>:"Read From Spreadsheet File.vi"("format (%.3f)"="%.8f", "file path (dialog if empty)"=w1546) -> ("first row"=w1538:dbl[])  [unwired: 5 in, 4 out]
                    n504 = call "zern2command.vi"("Haso configuration file"=w1536, "idxType"=w1526, "interaction matrix file"=w1537, "Zern coef in"=w1538, "Zern index in"=w1531, "Initial haso file"=w1535) -> ("error out"=w1539:errorcluster, "Offset Positions"=w1530:sgl[], "Zern pupil out"=w1540:refnum<class "Pupil.lvclass">, "ModalCoef out"=w1541:refnum<class "ModalCoef.lvclass">)  [unwired: 2 in]
                    n505 = call <userlib>:"LVClass_ModalCoef GetData.vi"("ModalCoef in"=w1541, "Pupil.lvclass"=w1540, "error in (no error)"=w1539) -> ("ModalCoef out"=w1545:refnum<class "ModalCoef.lvclass">, "Pupil.lvclass (dup)"=w1544:refnum<class "Pupil.lvclass">, "error out"=w1543:errorcluster)  [unwired: 8 in, 2 out]
                    n506 = call <userlib>:"LVClass_Pupil dtor.vi"("Pupil in"=w1544, "error in (no error)"=w1543) -> ("error out"=w1542:errorcluster)  [unwired: 12 in, 1 out]
                    n507 = call <userlib>:"LVClass_ModalCoef dtor.vi"("ModalCoef in"=w1545, "error in (no error)"=w1542) -> ("error out"=w1529:errorcluster)  [unwired: 12 in, 1 out]
                    n508 = Merge Errors(w1529, w1528) -> (w1527:errorcluster)
                  }
                }
              }
            }
            n509 = local read "File Base Name"() -> (w1348:string)
            n510 = local read "AO output"() -> (w1352:path)
            n511 = local read "Input type"() -> (w1349:T8)
            n512 = local read "Save File"() -> (w1353:bool)
            n513 = local write "Initial Positions"(w1346) -> ()
            n514 = Add(x=w1347, y=w1346) -> (x+y=w1350:dbl[])
            n515 = call <userlib>:"LVClass_WavefrontCorrector Move to Absolute Position.vi"("WavefrontCorrector in"=w1356, "Absolute Positions"=w1350, "error in (no error)"=w1358) -> ("WavefrontCorrector out"=w1359:refnum<class "WavefrontCorrector.lvclass">, "error out"=w1360:errorcluster)  [unwired: 11 in]
            n516 = call <userlib>:"LVClass_WavefrontCorrector Get Current Position.vi"("WavefrontCorrector in"=w1359, "error in (no error)"=w1360) -> ("WavefrontCorrector out"=w1354:refnum<class "WavefrontCorrector.lvclass">, "Wavefront Corrector Position"=w1351:T18, "error out"=w1345:errorcluster)  [unwired: 11 in]
            n517 = case shown="True" w1353 {
              tunnel: w1352 -> [_ w1370]
              tunnel: w1348 -> [_ w1369]
              tunnel: w1346 -> [_ w1368]
              tunnel: w1347 -> [_ w1367]
              tunnel: w1350 -> [_ w1366]
              tunnel: w1349 -> [_ w1365]
              tunnel: w1351 -> [_ w1364]
              frame False {
              }
              frame True {
                n518 = stacked-sequence {
                  tunnel: w1370 -> [w1375 w1384 w1393 w1402 w1409 w1421 w1433]
                  tunnel: w1369 -> [w1373 w1382 w1391 w1400 w1408 w1420 w1432]
                  tunnel: w1368 -> [w1371 _ _ _ _ _ _]
                  tunnel: w1367 -> [_ w1380 _ _ _ _ _]
                  tunnel: w1366 -> [_ _ w1389 _ _ _ _]
                  tunnel: w1365 -> [_ _ _ _ w1407 w1419 w1431]
                  tunnel: w1364 -> [_ _ _ w1398 _ _ _]
                  frame #0 {
                    n519 = Concatenate Strings(w1373, "_cmdOffset", ".dat") -> (w1376:string)
                    n520 = Build Path(base path=w1375, name or relative path=w1376) -> (appended path=w1377:path)
                    n521 = Array To Spreadsheet String(array=w1371, 3:"%f") -> (spreadsheet string=w1378:string)  [unwired: 1 in]
                    n522 = Write to Text File(file (use dialog)=w1377, text=w1378) -> ()  [unwired: 2 in, 3 out]
                  }
                  frame #1 {
                    n523 = Concatenate Strings(w1382, "_cmdAdd", ".dat") -> (w1385:string)
                    n524 = Build Path(base path=w1384, name or relative path=w1385) -> (appended path=w1386:path)
                    n525 = Array To Spreadsheet String(array=w1380, 3:"%f") -> (spreadsheet string=w1387:string)  [unwired: 1 in]
                    n526 = Write to Text File(file (use dialog)=w1386, text=w1387) -> ()  [unwired: 2 in, 3 out]
                  }
                  frame #2 {
                    n527 = Concatenate Strings(w1391, "_cmdFinal", ".dat") -> (w1394:string)
                    n528 = Build Path(base path=w1393, name or relative path=w1394) -> (appended path=w1395:path)
                    n529 = Array To Spreadsheet String(array=w1389, 3:"%f") -> (spreadsheet string=w1396:string)  [unwired: 1 in]
                    n530 = Write to Text File(file (use dialog)=w1395, text=w1396) -> ()  [unwired: 2 in, 3 out]
                  }
                  frame #3 {
                    n531 = Concatenate Strings(w1400, "_cmdFinalMirror", ".dat") -> (w1403:string)
                    n532 = Build Path(base path=w1402, name or relative path=w1403) -> (appended path=w1404:path)
                    n533 = Array To Spreadsheet String(array=w1398, 3:"%f") -> (spreadsheet string=w1405:string)  [unwired: 1 in]
                    n534 = Write to Text File(file (use dialog)=w1404, text=w1405) -> ()  [unwired: 2 in, 3 out]
                  }
                  frame #4 {
                    n535 = case shown="\"Zero Input\"" w1407 {
                      tunnel: w1409 -> [_ w1414]
                      tunnel: w1408 -> [_ w1412]
                      frame "Zero Input" {
                      }
                      frame "Zernike Coef", Default {
                        n536 = local read "Zern/DM coef in"() -> (w1410:sgl[])
                        n537 = Concatenate Strings(w1412, "_zernCoef", ".txt") -> (w1415:string)
                        n538 = Build Path(base path=w1414, name or relative path=w1415) -> (appended path=w1416:path)
                        n539 = Array To Spreadsheet String(array=w1410, 3:"%f") -> (spreadsheet string=w1417:string)  [unwired: 1 in]
                        n540 = Write to Text File(file (use dialog)=w1416, text=w1417) -> ()  [unwired: 2 in, 3 out]
                      }
                    }
                  }
                  frame #5 {
                    n541 = case shown="\"Zernike Coef\", Default" w1419 {
                      tunnel: w1421 -> [_ w1426]
                      tunnel: w1420 -> [_ w1424]
                      frame "Zero Input" {
                      }
                      frame "Zernike Coef", Default {
                        n542 = local read "Zern/DM index in"() -> (w1422:i32[])
                        n543 = Concatenate Strings(w1424, "_zernIdx", ".txt") -> (w1427:string)
                        n544 = Build Path(base path=w1426, name or relative path=w1427) -> (appended path=w1428:path)
                        n545 = Array To Spreadsheet String(array=w1422, 3:"%d") -> (spreadsheet string=w1429:string)  [unwired: 1 in]
                        n546 = Write to Text File(file (use dialog)=w1428, text=w1429) -> ()  [unwired: 2 in, 3 out]
                      }
                    }
                  }
                  frame #6 {
                    n547 = case shown="\"Zernike Coef\", Default" w1431 {
                      tunnel: w1433 -> [_ w1438]
                      tunnel: w1432 -> [_ w1436]
                      frame "Zero Input" {
                      }
                      frame "Zernike Coef", Default {
                        n548 = Concatenate Strings(w1436, "_zernCoefWyant", ".txt") -> (w1439:string)
                        n549 = local read "Coef out"() -> (w1434:sgl[])
                        n550 = Build Path(base path=w1438, name or relative path=w1439) -> (appended path=w1440:path)
                        n551 = Array To Spreadsheet String(array=w1434, 3:"%f") -> (spreadsheet string=w1441:string)  [unwired: 1 in]
                        n552 = Write to Text File(file (use dialog)=w1440, text=w1441) -> ()  [unwired: 2 in, 3 out]
                      }
                    }
                  }
                }
              }
            }
            n553 = local write "Final Positions"(w1350) -> ()
            n554 = local write "DM Actuator Values"(w1351) -> ()
            n555 = flat-sequence {
              tunnel: [w1362] -> w1344
              tunnel: w1345 -> [w1362]
              frame #0 {
                n556 = Wait (ms)(milliseconds to wait=u32 50) -> ()  [unwired: 1 out]
              }
            }
          }
          frame #2 {
            n557 = local read "HASO ready"() -> (w1553:bool)
            n558 = case shown="True" w1553 {
              tunnel: w1562 -> [_ w1588]
              tunnel: w1560 -> [_ w1587]
              tunnel: w1559 -> [_ w1586]
              tunnel: [w1563 w1585] -> w1549
              tunnel: w1561 -> [_ w1584]
              tunnel: w1554 -> [_ w1570]
              tunnel: w1550 -> [w1563 w1571]
              tunnel: w1557 -> [w1566 w1583]
              tunnel: w1556 -> [w1565 w1582]
              tunnel: [w1566 w1581] -> w1548
              tunnel: [w1565 w1580] -> _
              tunnel: w1558 -> [w1567 w1579]
              tunnel: w1555 -> [w1564 w1578]
              tunnel: [w1567 w1577] -> w1552
              tunnel: [w1564 w1576] -> w1551
              frame False {
              }
              frame True {
                n559 = property on="nb_images (set)" class="DigNum (strict)"() -> ("Value"=w1589:u32)  [unwired: 2 in, 2 out]
                n560 = case shown="2, Default" w1589 {
                  tunnel: [w1677 w1679] -> w1572
                  tunnel: w1584 -> [w1676 _]
                  tunnel: w1588 -> [w1677 _]
                  tunnel: [w1676 w1678] -> w1573
                  tunnel: w1587 -> [_ w1679]
                  tunnel: w1586 -> [_ w1678]
                  frame 2, Default {
                  }
                  frame 1 {
                  }
                }
                n561 = stacked-sequence {
                  tunnel: w1572 -> [_ w1607]
                  tunnel: w1573 -> [_ w1606]
                  tunnel: [_ w1605] -> w1569
                  tunnel: [_ w1603] -> w1568
                  tunnel: [_ w1602] -> _
                  tunnel: w1570 -> [_ w1599]
                  tunnel: w1571 -> [_ w1598]
                  frame #0 {
                    # "Delay until MD gets stable"
                    n562 = local read "exposure_duration_s (set)"() -> (w1590:dbl)
                    n563 = local read "nb_images (set)"() -> (w1591:u32)
                    n564 = Multiply(x=w1590, y=w1591) -> (x*y=w1592:dbl)
                    n565 = Add(x=w1592, y=1.0) -> (x+y=w1593:dbl)
                    n566 = Multiply(x=w1593, y=1000.0) -> (x*y=w1597:dbl)
                    n567 = To Unsigned Long Integer(number=w1597) -> (unsigned 32bit integer=w1596:u32)
                    n568 = Wait (ms)(milliseconds to wait=w1596) -> ()  [unwired: 1 out]
                  }
                  frame #1 {
                    n569 = while {
                      tunnel: w1599 -> [w1612]
                      tunnel: [w1611] -> w1601
                      tunnel: w1598 -> [w1609]
                      tunnel: [w1608] -> w1600
                      stop <- w1610 stop-if-true
                      n570 = call <userlib>:"LVClass_Camera asynchroneImageReady.vi"("Camera in"=w1612, "error in (no error)"=w1609) -> ("Camera out"=w1611:refnum<class "Camera.lvclass">, "ready"=w1610:bool, "error out"=w1608:errorcluster)  [unwired: 11 in]
                    }
                    n571 = call <userlib>:"LVClass_Camera get image.vi"("Camera in"=w1601, "Image"=w1607, "Image RAW"=w1606, "remove_background"=FALSE, "error in (no error)"=w1600) -> ("Camera out"=w1602:refnum<class "Camera.lvclass">, "Image (dup)"=w1605:refnum<class "Image.lvclass">, "error out"=w1603:errorcluster)  [unwired: 7 in, 1 out]
                  }
                }
                n572 = case shown="No Error" w1568 {
                  selector: w1568 -> [w1673 w1674]
                  tunnel: w1569 -> [w1672 w1675]
                  tunnel: [w1669 w1675] -> w1575
                  tunnel: [w1670 w1674] -> w1574
                  frame No Error {
                    # "get image"
                    n573 = call <userlib>:"LVClass_Image get image data.vi"("Image in"=w1672, "error in (no error)"=w1673) -> ("Image out"=w1669:refnum<class "Image.lvclass">, "Image data out"=w1671:u32[][], "error out"=w1670:errorcluster)  [unwired: 11 in]
                    n574 = local write "HASO intensity"(w1671) -> ()
                  }
                  frame Error {
                  }
                }
                n575 = case shown="Error" w1574 {
                  selector: w1574 -> [w1636 w1668]
                  tunnel: [w1642 w1668] -> w1585
                  tunnel: w1575 -> [w1635 _]
                  tunnel: [w1640 w1664] -> w1576
                  tunnel: [w1639 w1667] -> w1577
                  tunnel: w1583 -> [w1632 w1666]
                  tunnel: w1582 -> [w1631 w1665]
                  tunnel: [w1619 w1666] -> w1581
                  tunnel: [w1630 w1665] -> w1580
                  tunnel: w1579 -> [w1628 w1667]
                  tunnel: w1578 -> [w1626 w1664]
                  frame No Error {
                    # "phaseout"
                    n576 = local read "File Base Name"() -> (w1617:string)
                    n577 = local read "Save File"() -> (w1618:bool)
                    n578 = local read "AO output"() -> (w1616:path)
                    n579 = call "image2slopes.vi"("error in (no error)"=w1636, "Image in"=w1635, "HasoEngine in"=w1631, "HasoSlopes in"=w1632) -> ("error out"=w1629:errorcluster, "HasoEngine out"=w1630:refnum<class "HasoEngine.lvclass">, "HasoSlopes out"=w1613:refnum<class "HasoSlopes.lvclass">)  [unwired: 4 in, 1 out]
                    n580 = local read "Filter"() -> (w1625:u8[])
                    n581 = call "slopes2phase.vi"("TypePhase"=WavefrontReconstructionMode."Modal_Zernike", "Number of coefficients"=u8 32, "error in (no error)"=w1629, "Filter"=w1625, "HasoSlopes in"=w1613, "Phase in"=w1628) -> ("error out"=w1621:errorcluster, "HasoSlopes out"=w1622:refnum<class "HasoSlopes.lvclass">, "Phase out"=w1627:refnum<class "Phase.lvclass">)  [unwired: 3 in]
                    n582 = local read "idxType"() -> (w1615:enum16{"Wyant", "ANSI"})
                    n583 = call "slopes2zern.vi"("HasoSlopes in"=w1622, "error in (no error)"=w1621, "idxType"=w1615) -> ("HasoSlopes out"=w1619:refnum<class "HasoSlopes.lvclass">, "Zernike Coefficients"=w1614:dbl[], "error out"=w1620:errorcluster)  [unwired: 3 in, 2 out]
                    n584 = call <userlib>:"LVClass_Pupil ctor from HasoSlopes.vi"("Pupil in"=w1626, "HasoSlopes.lvclass"=w1613, "error in (no error)"=w1620) -> ("Pupil out"=w1637:refnum<class "Pupil.lvclass">, "error out"=w1638:errorcluster)  [unwired: 11 in]
                    n585 = case shown="True" w1618 {
                      tunnel: w1617 -> [_ w1647]
                      tunnel: w1616 -> [_ w1646]
                      tunnel: w1614 -> [_ w1645]
                      tunnel: w1613 -> [_ w1644]
                      frame False {
                      }
                      frame True {
                        n586 = stacked-sequence {
                          tunnel: w1647 -> [w1651 w1657]
                          tunnel: w1646 -> [w1650 w1656]
                          tunnel: w1645 -> [_ w1655]
                          tunnel: w1644 -> [w1648 _]
                          frame #0 {
                            n587 = Concatenate Strings(w1651, "_slopesMeas", ".has") -> (w1654:string)
                            n588 = Build Path(base path=w1650, name or relative path=w1654) -> (appended path=w1649:path)
                            n589 = call <userlib>:"LVClass_HasoSlopes Save.vi"("HasoSlopes in"=w1648, "path"=w1649) -> ()  [unwired: 12 in, 2 out]
                          }
                          frame #1 {
                            n590 = Concatenate Strings(w1657, "_zernCoefMeas", ".txt") -> (w1660:string)
                            n591 = Build Path(base path=w1656, name or relative path=w1660) -> (appended path=w1661:path)
                            n592 = Array To Spreadsheet String(array=w1655, 3:"%f") -> (spreadsheet string=w1662:string)  [unwired: 1 in]
                            n593 = Write to Text File(file (use dialog)=w1661, text=w1662) -> ()  [unwired: 2 in, 3 out]
                          }
                        }
                      }
                    }
                    n594 = call <userlib>:"LVClasse_Phase GetStatisticDatas.vi"("Phase in"=w1627, "error in (no error)"=w1638) -> ("Phase out"=w1643:refnum<class "Phase.lvclass">, "StatisticsData"=w1623:T2, "error out"=w1641:errorcluster)  [unwired: 11 in]
                    n595 = local write "Phase statistics"(w1623) -> ()
                    n596 = call <userlib>:"LVClasse_Phase Get Data.vi"("Phase in"=w1643, "Pupil"=w1637, "error in (no error)"=w1641) -> ("Phase out"=w1639:refnum<class "Phase.lvclass">, "data"=w1624:sgl[][], "Pupil (dup)"=w1640:refnum<class "Pupil.lvclass">, "error out"=w1642:errorcluster)  [unwired: 9 in]
                    n597 = local write "Zernike Measured"(w1614) -> ()
                    n598 = local write "Phase values"(w1624) -> ()
                  }
                  frame Error {
                  }
                }
              }
            }
          }
          frame #3 {
            # "Apply offset to DM"
            n599 = case shown="True" w1680 {
              tunnel: w1683 -> [_ w1691]
              tunnel: [w1684 w1685] -> w1682
              tunnel: w1681 -> [w1684 w1687]
              frame False {
              }
              frame True {
                # "Delay for DM response"
                n600 = local read "Initial offset"() -> (w1690:bool)
                n601 = case shown="True" w1690 {
                  tunnel: [w1696 w1701] -> w1688
                  frame False {
                    n602 = Initialize Array(0.0, 52) -> (w1696:dbl[])
                  }
                  frame True {
                    n603 = local read "Offset command file"() -> (w1700:path)
                    n604 = call-poly <vilib>:"Read From Spreadsheet File.vi"("format (%.3f)"="%.8f", "file path (dialog if empty)"=w1700) -> ("first row"=w1701:dbl[])  [unwired: 5 in, 4 out]
                  }
                }
                n605 = local write "Initial Positions"(w1688) -> ()
                n606 = call <userlib>:"LVClass_WavefrontCorrector Move to Absolute Position.vi"("WavefrontCorrector in"=w1691, "Absolute Positions"=w1688, "error in (no error)"=w1687) -> ("WavefrontCorrector out"=w1692:refnum<class "WavefrontCorrector.lvclass">, "error out"=w1693:errorcluster)  [unwired: 11 in]
                n607 = call <userlib>:"LVClass_WavefrontCorrector Get Current Position.vi"("WavefrontCorrector in"=w1692, "error in (no error)"=w1693) -> ("Wavefront Corrector Position"=w1689:T18, "error out"=w1686:errorcluster)  [unwired: 11 in, 1 out]
                n608 = local write "Initial Positions"(w1689) -> ()
                n609 = flat-sequence {
                  tunnel: [w1694] -> w1685
                  tunnel: w1686 -> [w1694]
                  frame #0 {
                    n610 = Wait (ms)(milliseconds to wait=u32 50) -> ()  [unwired: 1 out]
                  }
                }
              }
            }
          }
          frame #4 {
            n611 = case shown="True" w1704 {
              tunnel: w1715 -> [_ w1730]
              tunnel: w1714 -> [_ w1729]
              tunnel: w1713 -> [_ w1728]
              tunnel: w1712 -> [_ w1727]
              tunnel: w1711 -> [_ w1726]
              tunnel: w1703 -> [w1716 w1725]
              tunnel: w1710 -> [_ w1724]
              tunnel: w1709 -> [_ w1723]
              tunnel: w1708 -> [_ w1722]
              tunnel: w1707 -> [w1717 w1720]
              tunnel: [w1717 w1719] -> w1705
              tunnel: [w1716 w1718] -> w1702
              frame False {
              }
              frame True {
                n612 = local read "HASO ready"() -> (w1721:bool)
                n613 = case shown="True" w1721 {
                  tunnel: w1730 -> [_ w1758]
                  tunnel: w1728 -> [_ w1757]
                  tunnel: w1727 -> [_ w1756]
                  tunnel: [w1731 w1755] -> w1719
                  tunnel: w1729 -> [_ w1754]
                  tunnel: w1722 -> [_ w1738]
                  tunnel: w1720 -> [w1731 w1737]
                  tunnel: w1725 -> [w1734 w1742]
                  tunnel: w1724 -> [w1733 w1753]
                  tunnel: [w1734 w1744] -> w1718
                  tunnel: [w1733 w1752] -> _
                  tunnel: w1726 -> [w1735 w1751]
                  tunnel: w1723 -> [w1732 w1750]
                  tunnel: [w1735 w1749] -> _
                  tunnel: [w1732 w1748] -> _
                  frame False {
                  }
                  frame True {
                    n614 = property on="nb_images (set)" class="DigNum (strict)"() -> ("Value"=w1759:u32)  [unwired: 2 in, 2 out]
                    n615 = case shown="2, Default" w1759 {
                      tunnel: [w1861 w1863] -> w1740
                      tunnel: w1754 -> [w1860 _]
                      tunnel: w1758 -> [w1861 _]
                      tunnel: [w1860 w1862] -> w1739
                      tunnel: w1757 -> [_ w1863]
                      tunnel: w1756 -> [_ w1862]
                      frame 2, Default {
                      }
                      frame 1 {
                      }
                    }
                    n616 = stacked-sequence {
                      tunnel: w1740 -> [_ w1777]
                      tunnel: w1739 -> [_ w1776]
                      tunnel: [_ w1775] -> w1741
                      tunnel: [_ w1773] -> w1736
                      tunnel: [_ w1772] -> _
                      tunnel: w1738 -> [_ w1769]
                      tunnel: w1737 -> [_ w1768]
                      frame #0 {
                        # "Delay until MD gets stable"
                        n617 = local read "exposure_duration_s (set)"() -> (w1760:dbl)
                        n618 = local read "nb_images (set)"() -> (w1761:u32)
                        n619 = Multiply(x=w1760, y=w1761) -> (x*y=w1762:dbl)
                        n620 = Add(x=w1762, y=1.0) -> (x+y=w1763:dbl)
                        n621 = Multiply(x=w1763, y=1000.0) -> (x*y=w1767:dbl)
                        n622 = To Unsigned Long Integer(number=w1767) -> (unsigned 32bit integer=w1766:u32)
                        n623 = Wait (ms)(milliseconds to wait=w1766) -> ()  [unwired: 1 out]
                      }
                      frame #1 {
                        n624 = while {
                          tunnel: w1769 -> [w1782]
                          tunnel: [w1781] -> w1771
                          tunnel: w1768 -> [w1779]
                          tunnel: [w1778] -> w1770
                          stop <- w1780 stop-if-true
                          n625 = call <userlib>:"LVClass_Camera asynchroneImageReady.vi"("Camera in"=w1782, "error in (no error)"=w1779) -> ("Camera out"=w1781:refnum<class "Camera.lvclass">, "ready"=w1780:bool, "error out"=w1778:errorcluster)  [unwired: 11 in]
                        }
                        n626 = call <userlib>:"LVClass_Camera get image.vi"("Camera in"=w1771, "Image"=w1777, "Image RAW"=w1776, "remove_background"=FALSE, "error in (no error)"=w1770) -> ("Camera out"=w1772:refnum<class "Camera.lvclass">, "Image (dup)"=w1775:refnum<class "Image.lvclass">, "error out"=w1773:errorcluster)  [unwired: 7 in, 1 out]
                      }
                    }
                    n627 = case shown="No Error" w1736 {
                      selector: w1736 -> [w1857 w1858]
                      tunnel: w1741 -> [w1854 w1859]
                      tunnel: [w1853 w1859] -> w1747
                      tunnel: [w1852 w1858] -> w1746
                      frame No Error {
                        # "get image"
                        n628 = call <userlib>:"LVClass_Image get image data.vi"("Image in"=w1854, "error in (no error)"=w1857) -> ("Image out"=w1856:refnum<class "Image.lvclass">, "Image data out"=w1851:u32[][], "error out"=w1855:errorcluster)  [unwired: 11 in]
                        n629 = call <userlib>:"LVClass_Image get image information.vi"("Image in"=w1856, "error in (no error)"=w1855) -> ("Image out"=w1853:refnum<class "Image.lvclass">, "error out"=w1852:errorcluster)  [unwired: 11 in, 1 out]
                        n630 = local write "HASO intensity"(w1851) -> ()
                      }
                      frame Error {
                      }
                    }
                    n631 = case shown="No Error" w1746 {
                      selector: w1746 -> [w1809 w1850]
                      tunnel: [w1815 w1850] -> w1755
                      tunnel: w1747 -> [w1808 _]
                      tunnel: [w1813 w1847] -> w1748
                      tunnel: [w1812 w1849] -> w1749
                      tunnel: refnum<class "HasoSlopes.lvclass"> refnum ("HasoSlopes in") -> [w1805 w1846]
                      tunnel: w1753 -> [w1804 w1848]
                      tunnel: [w1803 w1848] -> w1752
                      tunnel: w1751 -> [w1802 w1849]
                      tunnel: w1750 -> [w1800 w1847]
                      tunnel: [w1785 w1845] -> w1744
                      tunnel: [w1783 w1846] -> w1743
                      tunnel: w1742 -> [w1784 w1845]
                      frame No Error {
                        # "phaseout"
                        n632 = local read "File Base Name"() -> (w1792:string)
                        n633 = local read "Save File"() -> (w1793:bool)
                        n634 = local read "AO output"() -> (w1791:path)
                        n635 = call "image2slopes.vi"("error in (no error)"=w1809, "Image in"=w1808, "HasoEngine in"=w1804, "HasoSlopes in"=w1805) -> ("error out"=w1787:errorcluster, "HasoEngine out"=w1803:refnum<class "HasoEngine.lvclass">, "HasoSlopes out"=w1783:refnum<class "HasoSlopes.lvclass">)  [unwired: 4 in, 1 out]
                        n636 = local read "Filter"() -> (w1799:u8[])
                        n637 = call <userlib>:"LVClass_HasoSlopes Apply Substractor.vi"("HasoSlopes in"=w1784, "HasoSlopes to substract"=w1783, "error in (no error)"=w1787) -> ("HasoSlopes out"=w1788:refnum<class "HasoSlopes.lvclass">, "error out"=w1786:errorcluster)  [unwired: 11 in]
                        n638 = call "slopes2phase.vi"("TypePhase"=WavefrontReconstructionMode."Modal_Zernike", "Number of coefficients"=u8 32, "error in (no error)"=w1786, "Filter"=w1799, "HasoSlopes in"=w1788, "Phase in"=w1802) -> ("error out"=w1795:errorcluster, "HasoSlopes out"=w1796:refnum<class "HasoSlopes.lvclass">, "Phase out"=w1801:refnum<class "Phase.lvclass">)  [unwired: 3 in]
                        n639 = local read "idxType"() -> (w1790:enum16{"Wyant", "ANSI"})
                        n640 = call "slopes2zern.vi"("HasoSlopes in"=w1796, "error in (no error)"=w1795, "idxType"=w1790) -> ("HasoSlopes out"=w1785:refnum<class "HasoSlopes.lvclass">, "Zernike Coefficients"=w1789:dbl[], "error out"=w1794:errorcluster)  [unwired: 3 in, 2 out]
                        n641 = call <userlib>:"LVClass_Pupil ctor from HasoSlopes.vi"("Pupil in"=w1800, "HasoSlopes.lvclass"=w1788, "error in (no error)"=w1794) -> ("Pupil out"=w1810:refnum<class "Pupil.lvclass">, "error out"=w1811:errorcluster)  [unwired: 11 in]
                        n642 = case shown="True" w1793 {
                          tunnel: w1792 -> [_ w1821]
                          tunnel: w1791 -> [_ w1820]
                          tunnel: w1789 -> [_ w1819]
                          tunnel: w1788 -> [_ w1817]
                          tunnel: w1783 -> [_ w1818]
                          frame False {
                          }
                          frame True {
                            n643 = stacked-sequence {
                              tunnel: w1821 -> [w1825 w1832 w1838]
                              tunnel: w1820 -> [w1824 w1831 w1837]
                              tunnel: w1819 -> [_ _ w1836]
                              tunnel: w1818 -> [w1822 _ _]
                              tunnel: w1817 -> [_ w1829 _]
                              frame #0 {
                                n644 = Concatenate Strings(w1825, "_slopesOffset", ".has") -> (w1828:string)
                                n645 = Build Path(base path=w1824, name or relative path=w1828) -> (appended path=w1823:path)
                                n646 = call <userlib>:"LVClass_HasoSlopes Save.vi"("HasoSlopes in"=w1822, "path"=w1823) -> ()  [unwired: 12 in, 2 out]
                              }
                              frame #1 {
                                n647 = Concatenate Strings(w1832, "_slopesNet", ".has") -> (w1835:string)
                                n648 = Build Path(base path=w1831, name or relative path=w1835) -> (appended path=w1830:path)
                                n649 = call <userlib>:"LVClass_HasoSlopes Save.vi"("HasoSlopes in"=w1829, "path"=w1830) -> ()  [unwired: 12 in, 2 out]
                              }
                              frame #2 {
                                n650 = Concatenate Strings(w1838, "_zernCoefNet", ".txt") -> (w1841:string)
                                n651 = Build Path(base path=w1837, name or relative path=w1841) -> (appended path=w1842:path)
                                n652 = Array To Spreadsheet String(array=w1836, 3:"%f") -> (spreadsheet string=w1843:string)  [unwired: 1 in]
                                n653 = Write to Text File(file (use dialog)=w1842, text=w1843) -> ()  [unwired: 2 in, 3 out]
                              }
                            }
                          }
                        }
                        n654 = call <userlib>:"LVClasse_Phase GetStatisticDatas.vi"("Phase in"=w1801, "error in (no error)"=w1811) -> ("Phase out"=w1816:refnum<class "Phase.lvclass">, "StatisticsData"=w1797:T2, "error out"=w1814:errorcluster)  [unwired: 11 in]
                        n655 = local write "Phase statistics"(w1797) -> ()
                        n656 = call <userlib>:"LVClasse_Phase Get Data.vi"("Phase in"=w1816, "Pupil"=w1810, "error in (no error)"=w1814) -> ("Phase out"=w1812:refnum<class "Phase.lvclass">, "data"=w1798:sgl[][], "Pupil (dup)"=w1813:refnum<class "Pupil.lvclass">, "error out"=w1815:errorcluster)  [unwired: 9 in]
                        n657 = local write "Zernike Measured"(w1789) -> ()
                        n658 = local write "Phase values"(w1798) -> ()
                      }
                      frame Error {
                      }
                    }
                    n659 = call <userlib>:"LVClass_HasoSlopes dtor.vi"("HasoSlopes in"=w1743) -> ()  [unwired: 13 in, 2 out]
                  }
                }
              }
            }
            n660 = Unbundle By Name(w1705) -> ("status"=w1706:bool)
          }
        }
      }
      event "Record Batch Zern": Mouse Up {
        n661 = event-data() -> ()  [unwired: 1 in, 8 out]
        n662 = local read "Idx start"() -> (w1864:u32)
        n663 = local read "Idx end"() -> (w1865:u32)
        n664 = Subtract(x=w1865, y=w1864) -> (x-y=w1866:u32)
        n665 = Increment(x=w1866) -> (x+1=w1867:u32)
        n666 = for {
          N: w1867 -> [_]
          tunnel: [w1906] -> w1885
          tunnel: w1879 -> [w1901]
          tunnel: w1878 -> [w1900]
          tunnel: w1877 -> [w1899]
          tunnel: w1876 -> [w1898]
          tunnel: w1873 -> [w1895]
          tunnel: w1872 -> [w1894]
          shift-right: [w1904] -> w1883
          shift-left: w1884 -> [w1905]
          shift-right: [w1902] -> w1880
          shift-left: w1882 -> [w1903]
          shift-right: [w1892] -> w1870
          shift-left: w1875 -> [w1897]
          shift-right: [w1893] -> w1871
          shift-left: w1874 -> [w1896]
          shift-right: [w1890] -> w1868
          shift-left: w1869 -> [w1891]
          tunnel: w1864 -> [w1887]
          i -> [w1888]
          n667 = Add(x=w1887, y=w1888) -> (x+y=w1886:u32)
          n668 = local read "Net Rp"() -> (w1889:bool)
          n669 = stacked-sequence {
            seq-local: [_ _ _ w2202 _] -> [_ _ _ _ w2227]
            seq-local: [_ _ w2067 _ _] -> [_ _ _ w2201 _]
            seq-local: [_ w1936 _ _ _] -> [_ _ w2068 _ _]
            seq-local: [_ _ w2066 _ _] -> [_ _ _ _ w2223]
            tunnel: [_ _ _ _ w2226] -> w1906
            tunnel: w1905 -> [_ w1949 _ _ _]
            tunnel: [_ _ _ _ w2225] -> w1904
            tunnel: w1903 -> [_ w1948 _ w2203 _]
            tunnel: [_ w1946 _ _ _] -> w1902
            tunnel: w1901 -> [_ _ w2080 _ w2235]
            tunnel: w1900 -> [_ _ w2079 _ w2234]
            tunnel: w1899 -> [_ _ w2078 _ w2233]
            tunnel: w1898 -> [_ _ w2077 _ w2232]
            tunnel: w1897 -> [_ _ w2076 _ w2231]
            tunnel: w1896 -> [_ _ w2075 _ _]
            tunnel: w1895 -> [_ _ w2074 _ w2230]
            tunnel: w1891 -> [_ _ w2073 _ w2229]
            tunnel: w1894 -> [_ _ w2072 _ w2228]
            tunnel: [_ _ _ _ w2222] -> w1893
            tunnel: [_ _ w2070 _ _] -> w1892
            tunnel: [_ _ w2069 _ _] -> w1890
            tunnel: w1889 -> [_ _ _ w2200 w2224]
            tunnel: w1886 -> [w1909 w1937 _ _ _]
            frame #0 {
              # "Create output folder path"
              n670 = local read "idxType"() -> (w1913:enum16{"Wyant", "ANSI"})
              n671 = Number To Decimal String(number=w1909) -> (decimal integer string=w1910:string)  [unwired: 1 in]
              n672 = local read "Base Path"() -> (w1907:path)
              n673 = case shown="\"ANSI\"" w1913 {
                tunnel: ["Wyant" "ANSI"] -> w1912
                frame "Wyant", Default {
                }
                frame "ANSI" {
                }
              }
              n674 = local read "Subfolder"() -> (w1919:string)
              n675 = Concatenate Strings(w1912, "_idx_", w1910) -> (w1908:string)
              n676 = Build Path(base path=w1907, name or relative path=w1919) -> (appended path=w1917:path)
              n677 = Build Path(base path=w1917, name or relative path=w1908) -> (appended path=w1914:path)
              n678 = local write "Current status"(w1908) -> ()
              n679 = call <vilib>:"Check if File or Folder Exists.vi"("path"=w1917) -> ("error out"=w1916:errorcluster, "file or folder exists?"=w1918:bool)  [unwired: 8 in, 1 out]
              n680 = case shown="True" w1918 {
                tunnel: w1917 -> [w1926 _]
                tunnel: w1916 -> [w1925 w1927]
                tunnel: [w1924 w1927] -> w1915
                frame False {
                  n681 = Create Folder(path (use dialog)=w1926, error in=w1925) -> (error out=w1924:errorcluster)  [unwired: 1 in, 2 out]
                }
                frame True {
                }
              }
              n682 = call <vilib>:"Check if File or Folder Exists.vi"("error in (no error)"=w1915, "path"=w1914) -> ("error out"=w1920:errorcluster, "file or folder exists?"=w1921:bool)  [unwired: 7 in, 1 out]
              n683 = case shown="False" w1921 {
                tunnel: w1914 -> [w1929 w1933]
                tunnel: w1920 -> [w1928 w1934]
                frame False {
                  n684 = Create Folder(path (use dialog)=w1929, error in=w1928) -> ()  [unwired: 1 in, 3 out]
                }
                frame True {
                  n685 = Delete(path (use dialog)=w1933, entire hierarchy (F)=TRUE, error in=w1934) -> (deleted path=w1931:path, error out=w1930:errorcluster)  [unwired: 2 in, 1 out]
                  n686 = Create Folder(path (use dialog)=w1931, error in=w1930) -> ()  [unwired: 1 in, 3 out]
                }
              }
              n687 = local write "AO output"(w1914) -> ()
            }
            frame #1 {
              # "Delay for DM response"
              # "Apply command to DM"
              n688 = local read "Initial offset"() -> (w1947:bool)
              n689 = case shown="True" w1947 {
                tunnel: [w2035 w2040] -> w1938
                frame False {
                  n690 = Initialize Array(0.0, 52) -> (w2035:dbl[])
                }
                frame True {
                  n691 = local read "Offset command file"() -> (w2039:path)
                  n692 = call-poly <vilib>:"Read From Spreadsheet File.vi"("format (%.3f)"="%.8f", "file path (dialog if empty)"=w2039) -> ("first row"=w2040:dbl[])  [unwired: 5 in, 4 out]
                }
              }
              n693 = local read "Additional Command"() -> (w1953:bool)
              n694 = case shown="True" w1953 {
                tunnel: [w2042 w2065] -> w1939
                tunnel: [w2041 w2064] -> w1950
                tunnel: w1949 -> [w2041 w2063]
                tunnel: w1937 -> [_ w2046]
                frame False {
                  n695 = Initialize Array(0.0, 52) -> (w2042:dbl[])
                }
                frame True {
                  w2047 = 1
                  n696 = local read "Coef value"() -> (w2049:dbl)
                  n697 = local read "Initial haso file"() -> (w2053:path)
                  n698 = Initialize Array(w2046, w2047) -> (w2045:u32[])
                  n699 = Initialize Array(w2049, w2047) -> (w2048:dbl[])
                  n700 = local read "Haso configuration file"() -> (w2054:path)
                  n701 = local read "interaction matrix file"() -> (w2052:path)
                  n702 = local read "idxType"() -> (w2055:enum16{"Wyant", "ANSI"})
                  n703 = call "zern2command.vi"("Haso configuration file"=w2054, "idxType"=w2055, "interaction matrix file"=w2052, "error in (no error)"=w2063, "Zern coef in"=w2048, "Zern index in"=w2045, "Initial haso file"=w2053) -> ("error out"=w2056:errorcluster, "Offset Positions"=w2065:sgl[], "Zern pupil out"=w2057:refnum<class "Pupil.lvclass">, "ModalCoef out"=w2058:refnum<class "ModalCoef.lvclass">)  [unwired: 1 in]
                  n704 = call <userlib>:"LVClass_ModalCoef GetData.vi"("ModalCoef in"=w2058, "Pupil.lvclass"=w2057, "error in (no error)"=w2056) -> ("ModalCoef out"=w2062:refnum<class "ModalCoef.lvclass">, "coef"=w2051:sgl[], "index"=w2050:u32[], "Pupil.lvclass (dup)"=w2061:refnum<class "Pupil.lvclass">, "error out"=w2060:errorcluster)  [unwired: 8 in]
                  n705 = local write "Index out"(w2050) -> ()
                  n706 = call <userlib>:"LVClass_Pupil dtor.vi"("Pupil in"=w2061, "error in (no error)"=w2060) -> ("error out"=w2059:errorcluster)  [unwired: 12 in, 1 out]
                  n707 = local write "Coef out"(w2051) -> ()
                  n708 = call <userlib>:"LVClass_ModalCoef dtor.vi"("ModalCoef in"=w2062, "error in (no error)"=w2059) -> ("error out"=w2064:errorcluster)  [unwired: 12 in, 1 out]
                }
              }
              n709 = local read "File Base Name"() -> (w1940:string)
              n710 = local read "AO output"() -> (w1944:path)
              n711 = local read "Input type"() -> (w1941:T8)
              n712 = local read "Save File"() -> (w1945:bool)
              n713 = local write "Initial Positions"(w1938) -> ()
              n714 = Add(x=w1939, y=w1938) -> (x+y=w1942:dbl[])
              n715 = call <userlib>:"LVClass_WavefrontCorrector Move to Absolute Position.vi"("WavefrontCorrector in"=w1948, "Absolute Positions"=w1942, "error in (no error)"=w1950) -> ("WavefrontCorrector out"=w1951:refnum<class "WavefrontCorrector.lvclass">, "error out"=w1952:errorcluster)  [unwired: 11 in]
              n716 = call <userlib>:"LVClass_WavefrontCorrector Get Current Position.vi"("WavefrontCorrector in"=w1951, "error in (no error)"=w1952) -> ("WavefrontCorrector out"=w1946:refnum<class "WavefrontCorrector.lvclass">, "Wavefront Corrector Position"=w1943:T18, "error out"=w1935:errorcluster)  [unwired: 11 in]
              n717 = case shown="True" w1945 {
                tunnel: w1944 -> [_ w1962]
                tunnel: w1940 -> [_ w1961]
                tunnel: w1938 -> [_ w1960]
                tunnel: w1939 -> [_ w1959]
                tunnel: w1942 -> [_ w1958]
                tunnel: w1941 -> [_ w1957]
                tunnel: w1943 -> [_ w1956]
                frame False {
                }
                frame True {
                  n718 = stacked-sequence {
                    tunnel: w1962 -> [w1967 w1976 w1985 w1994 w2001 w2013 w2025]
                    tunnel: w1961 -> [w1965 w1974 w1983 w1992 w2000 w2012 w2024]
                    tunnel: w1960 -> [w1963 _ _ _ _ _ _]
                    tunnel: w1959 -> [_ w1972 _ _ _ _ _]
                    tunnel: w1958 -> [_ _ w1981 _ _ _ _]
                    tunnel: w1957 -> [_ _ _ _ w1999 w2011 w2023]
                    tunnel: w1956 -> [_ _ _ w1990 _ _ _]
                    frame #0 {
                      n719 = Concatenate Strings(w1965, "_cmdOffset", ".dat") -> (w1968:string)
                      n720 = Build Path(base path=w1967, name or relative path=w1968) -> (appended path=w1969:path)
                      n721 = Array To Spreadsheet String(array=w1963, 3:"%f") -> (spreadsheet string=w1970:string)  [unwired: 1 in]
                      n722 = Write to Text File(file (use dialog)=w1969, text=w1970) -> ()  [unwired: 2 in, 3 out]
                    }
                    frame #1 {
                      n723 = Concatenate Strings(w1974, "_cmdAdd", ".dat") -> (w1977:string)
                      n724 = Build Path(base path=w1976, name or relative path=w1977) -> (appended path=w1978:path)
                      n725 = Array To Spreadsheet String(array=w1972, 3:"%f") -> (spreadsheet string=w1979:string)  [unwired: 1 in]
                      n726 = Write to Text File(file (use dialog)=w1978, text=w1979) -> ()  [unwired: 2 in, 3 out]
                    }
                    frame #2 {
                      n727 = Concatenate Strings(w1983, "_cmdFinal", ".dat") -> (w1986:string)
                      n728 = Build Path(base path=w1985, name or relative path=w1986) -> (appended path=w1987:path)
                      n729 = Array To Spreadsheet String(array=w1981, 3:"%f") -> (spreadsheet string=w1988:string)  [unwired: 1 in]
                      n730 = Write to Text File(file (use dialog)=w1987, text=w1988) -> ()  [unwired: 2 in, 3 out]
                    }
                    frame #3 {
                      n731 = Concatenate Strings(w1992, "_cmdFinalMirror", ".dat") -> (w1995:string)
                      n732 = Build Path(base path=w1994, name or relative path=w1995) -> (appended path=w1996:path)
                      n733 = Array To Spreadsheet String(array=w1990, 3:"%f") -> (spreadsheet string=w1997:string)  [unwired: 1 in]
                      n734 = Write to Text File(file (use dialog)=w1996, text=w1997) -> ()  [unwired: 2 in, 3 out]
                    }
                    frame #4 {
                      n735 = case shown="\"Zernike Coef\", Default" w1999 {
                        tunnel: w2001 -> [_ w2006]
                        tunnel: w2000 -> [_ w2004]
                        frame "Zero Input" {
                        }
                        frame "Zernike Coef", Default {
                          n736 = local read "Zern/DM coef in"() -> (w2002:sgl[])
                          n737 = Concatenate Strings(w2004, "_zernCoef", ".txt") -> (w2007:string)
                          n738 = Build Path(base path=w2006, name or relative path=w2007) -> (appended path=w2008:path)
                          n739 = Array To Spreadsheet String(array=w2002, 3:"%f") -> (spreadsheet string=w2009:string)  [unwired: 1 in]
                          n740 = Write to Text File(file (use dialog)=w2008, text=w2009) -> ()  [unwired: 2 in, 3 out]
                        }
                      }
                    }
                    frame #5 {
                      n741 = case shown="\"Zernike Coef\", Default" w2011 {
                        tunnel: w2013 -> [_ w2018]
                        tunnel: w2012 -> [_ w2016]
                        frame "Zero Input" {
                        }
                        frame "Zernike Coef", Default {
                          n742 = local read "Zern/DM index in"() -> (w2014:i32[])
                          n743 = Concatenate Strings(w2016, "_zernIdx", ".txt") -> (w2019:string)
                          n744 = Build Path(base path=w2018, name or relative path=w2019) -> (appended path=w2020:path)
                          n745 = Array To Spreadsheet String(array=w2014, 3:"%d") -> (spreadsheet string=w2021:string)  [unwired: 1 in]
                          n746 = Write to Text File(file (use dialog)=w2020, text=w2021) -> ()  [unwired: 2 in, 3 out]
                        }
                      }
                    }
                    frame #6 {
                      n747 = case shown="\"Zernike Coef\", Default" w2023 {
                        tunnel: w2025 -> [_ w2030]
                        tunnel: w2024 -> [_ w2028]
                        frame "Zero Input" {
                        }
                        frame "Zernike Coef", Default {
                          n748 = Concatenate Strings(w2028, "_zernCoefWyant", ".txt") -> (w2031:string)
                          n749 = local read "Coef out"() -> (w2026:sgl[])
                          n750 = Build Path(base path=w2030, name or relative path=w2031) -> (appended path=w2032:path)
                          n751 = Array To Spreadsheet String(array=w2026, 3:"%f") -> (spreadsheet string=w2033:string)  [unwired: 1 in]
                          n752 = Write to Text File(file (use dialog)=w2032, text=w2033) -> ()  [unwired: 2 in, 3 out]
                        }
                      }
                    }
                  }
                }
              }
              n753 = local write "Final Positions"(w1942) -> ()
              n754 = local write "DM Actuator Values"(w1943) -> ()
              n755 = flat-sequence {
                tunnel: [w1954] -> w1936
                tunnel: w1935 -> [w1954]
                frame #0 {
                  n756 = Wait (ms)(milliseconds to wait=u32 50) -> ()  [unwired: 1 out]
                }
              }
            }
            frame #2 {
              n757 = local read "HASO ready"() -> (w2071:bool)
              n758 = case shown="True" w2071 {
                tunnel: w2080 -> [_ w2106]
                tunnel: w2078 -> [_ w2105]
                tunnel: w2077 -> [_ w2104]
                tunnel: [w2081 w2103] -> w2067
                tunnel: w2079 -> [_ w2102]
                tunnel: w2072 -> [_ w2089]
                tunnel: w2068 -> [w2081 w2088]
                tunnel: w2075 -> [w2084 w2101]
                tunnel: w2074 -> [w2083 w2100]
                tunnel: [w2084 w2099] -> w2066
                tunnel: [w2083 w2098] -> _
                tunnel: w2076 -> [w2085 w2097]
                tunnel: w2073 -> [w2082 w2096]
                tunnel: [w2085 w2095] -> w2070
                tunnel: [w2082 w2094] -> w2069
                frame False {
                }
                frame True {
                  n759 = property on="nb_images (set)" class="DigNum (strict)"() -> ("Value"=w2107:u32)  [unwired: 2 in, 2 out]
                  n760 = case shown="2, Default" w2107 {
                    tunnel: [w2197 w2199] -> w2087
                    tunnel: w2102 -> [w2196 _]
                    tunnel: w2106 -> [w2197 _]
                    tunnel: [w2196 w2198] -> w2086
                    tunnel: w2105 -> [_ w2199]
                    tunnel: w2104 -> [_ w2198]
                    frame 2, Default {
                    }
                    frame 1 {
                    }
                  }
                  n761 = stacked-sequence {
                    tunnel: w2087 -> [_ w2125]
                    tunnel: w2086 -> [_ w2124]
                    tunnel: [_ w2123] -> w2090
                    tunnel: [_ w2121] -> w2091
                    tunnel: [_ w2120] -> _
                    tunnel: w2089 -> [_ w2117]
                    tunnel: w2088 -> [_ w2116]
                    frame #0 {
                      # "Delay until MD gets stable"
                      n762 = local read "exposure_duration_s (set)"() -> (w2108:dbl)
                      n763 = local read "nb_images (set)"() -> (w2109:u32)
                      n764 = Multiply(x=w2108, y=w2109) -> (x*y=w2110:dbl)
                      n765 = Add(x=w2110, y=3.0) -> (x+y=w2111:dbl)
                      n766 = Multiply(x=w2111, y=1000.0) -> (x*y=w2115:dbl)
                      n767 = To Unsigned Long Integer(number=w2115) -> (unsigned 32bit integer=w2114:u32)
                      n768 = Wait (ms)(milliseconds to wait=w2114) -> ()  [unwired: 1 out]
                    }
                    frame #1 {
                      n769 = while {
                        tunnel: w2117 -> [w2130]
                        tunnel: [w2129] -> w2119
                        tunnel: w2116 -> [w2127]
                        tunnel: [w2126] -> w2118
                        stop <- w2128 stop-if-true
                        n770 = call <userlib>:"LVClass_Camera asynchroneImageReady.vi"("Camera in"=w2130, "error in (no error)"=w2127) -> ("Camera out"=w2129:refnum<class "Camera.lvclass">, "ready"=w2128:bool, "error out"=w2126:errorcluster)  [unwired: 11 in]
                      }
                      n771 = call <userlib>:"LVClass_Camera get image.vi"("Camera in"=w2119, "Image"=w2125, "Image RAW"=w2124, "remove_background"=FALSE, "error in (no error)"=w2118) -> ("Camera out"=w2120:refnum<class "Camera.lvclass">, "Image (dup)"=w2123:refnum<class "Image.lvclass">, "error out"=w2121:errorcluster)  [unwired: 7 in, 1 out]
                    }
                  }
                  n772 = case shown="No Error" w2091 {
                    selector: w2091 -> [w2193 w2194]
                    tunnel: w2090 -> [w2187 w2195]
                    tunnel: [w2190 w2195] -> w2093
                    tunnel: [w2189 w2194] -> w2092
                    frame No Error {
                      # "get image"
                      n773 = call <userlib>:"LVClass_Image get image data.vi"("Image in"=w2187, "error in (no error)"=w2193) -> ("Image out"=w2192:refnum<class "Image.lvclass">, "Image data out"=w2188:u32[][], "error out"=w2191:errorcluster)  [unwired: 11 in]
                      n774 = call <userlib>:"LVClass_Image get image information.vi"("Image in"=w2192, "error in (no error)"=w2191) -> ("Image out"=w2190:refnum<class "Image.lvclass">, "error out"=w2189:errorcluster)  [unwired: 11 in, 1 out]
                      n775 = local write "HASO intensity"(w2188) -> ()
                    }
                    frame Error {
                    }
                  }
                  n776 = case shown="No Error" w2092 {
                    selector: w2092 -> [w2154 w2186]
                    tunnel: [w2160 w2186] -> w2103
                    tunnel: w2093 -> [w2153 _]
                    tunnel: [w2158 w2182] -> w2094
                    tunnel: [w2157 w2185] -> w2095
                    tunnel: w2101 -> [w2150 w2184]
                    tunnel: w2100 -> [w2149 w2183]
                    tunnel: [w2137 w2184] -> w2099
                    tunnel: [w2148 w2183] -> w2098
                    tunnel: w2097 -> [w2146 w2185]
                    tunnel: w2096 -> [w2144 w2182]
                    frame No Error {
                      # "phaseout"
                      n777 = local read "File Base Name"() -> (w2135:string)
                      n778 = local read "Save File"() -> (w2136:bool)
                      n779 = local read "AO output"() -> (w2134:path)
                      n780 = call "image2slopes.vi"("error in (no error)"=w2154, "Image in"=w2153, "HasoEngine in"=w2149, "HasoSlopes in"=w2150) -> ("error out"=w2147:errorcluster, "HasoEngine out"=w2148:refnum<class "HasoEngine.lvclass">, "HasoSlopes out"=w2131:refnum<class "HasoSlopes.lvclass">)  [unwired: 4 in, 1 out]
                      n781 = local read "Filter"() -> (w2143:u8[])
                      n782 = call "slopes2phase.vi"("TypePhase"=WavefrontReconstructionMode."Modal_Zernike", "Number of coefficients"=u8 32, "error in (no error)"=w2147, "Filter"=w2143, "HasoSlopes in"=w2131, "Phase in"=w2146) -> ("error out"=w2139:errorcluster, "HasoSlopes out"=w2140:refnum<class "HasoSlopes.lvclass">, "Phase out"=w2145:refnum<class "Phase.lvclass">)  [unwired: 3 in]
                      n783 = local read "idxType"() -> (w2133:enum16{"Wyant", "ANSI"})
                      n784 = call "slopes2zern.vi"("HasoSlopes in"=w2140, "error in (no error)"=w2139, "idxType"=w2133) -> ("HasoSlopes out"=w2137:refnum<class "HasoSlopes.lvclass">, "Zernike Coefficients"=w2132:dbl[], "error out"=w2138:errorcluster)  [unwired: 3 in, 2 out]
                      n785 = call <userlib>:"LVClass_Pupil ctor from HasoSlopes.vi"("Pupil in"=w2144, "HasoSlopes.lvclass"=w2131, "error in (no error)"=w2138) -> ("Pupil out"=w2155:refnum<class "Pupil.lvclass">, "error out"=w2156:errorcluster)  [unwired: 11 in]
                      n786 = case shown="True" w2136 {
                        tunnel: w2135 -> [_ w2165]
                        tunnel: w2134 -> [_ w2164]
                        tunnel: w2132 -> [_ w2163]
                        tunnel: w2131 -> [_ w2162]
                        frame False {
                        }
                        frame True {
                          n787 = stacked-sequence {
                            tunnel: w2165 -> [w2169 w2175]
                            tunnel: w2164 -> [w2168 w2174]
                            tunnel: w2163 -> [_ w2173]
                            tunnel: w2162 -> [w2166 _]
                            frame #0 {
                              n788 = Concatenate Strings(w2169, "_slopesMeas", ".has") -> (w2172:string)
                              n789 = Build Path(base path=w2168, name or relative path=w2172) -> (appended path=w2167:path)
                              n790 = call <userlib>:"LVClass_HasoSlopes Save.vi"("HasoSlopes in"=w2166, "path"=w2167) -> ()  [unwired: 12 in, 2 out]
                            }
                            frame #1 {
                              n791 = Concatenate Strings(w2175, "_zernCoefMeas", ".txt") -> (w2178:string)
                              n792 = Build Path(base path=w2174, name or relative path=w2178) -> (appended path=w2179:path)
                              n793 = Array To Spreadsheet String(array=w2173, 3:"%f") -> (spreadsheet string=w2180:string)  [unwired: 1 in]
                              n794 = Write to Text File(file (use dialog)=w2179, text=w2180) -> ()  [unwired: 2 in, 3 out]
                            }
                          }
                        }
                      }
                      n795 = call <userlib>:"LVClasse_Phase GetStatisticDatas.vi"("Phase in"=w2145, "error in (no error)"=w2156) -> ("Phase out"=w2161:refnum<class "Phase.lvclass">, "StatisticsData"=w2141:T2, "error out"=w2159:errorcluster)  [unwired: 11 in]
                      n796 = local write "Phase statistics"(w2141) -> ()
                      n797 = call <userlib>:"LVClasse_Phase Get Data.vi"("Phase in"=w2161, "Pupil"=w2155, "error in (no error)"=w2159) -> ("Phase out"=w2157:refnum<class "Phase.lvclass">, "data"=w2142:sgl[][], "Pupil (dup)"=w2158:refnum<class "Pupil.lvclass">, "error out"=w2160:errorcluster)  [unwired: 9 in]
                      n798 = local write "Zernike Measured"(w2132) -> ()
                      n799 = local write "Phase values"(w2142) -> ()
                    }
                    frame Error {
                    }
                  }
                }
              }
            }
            frame #3 {
              # "Apply offset to DM"
              n800 = case shown="True" w2200 {
                tunnel: w2203 -> [_ w2211]
                tunnel: [w2204 w2206] -> w2202
                tunnel: w2201 -> [w2204 w2207]
                frame False {
                }
                frame True {
                  # "Delay for DM response"
                  n801 = local read "Initial offset"() -> (w2210:bool)
                  n802 = case shown="True" w2210 {
                    tunnel: [w2216 w2221] -> w2208
                    frame False {
                      n803 = Initialize Array(0.0, 52) -> (w2216:dbl[])
                    }
                    frame True {
                      n804 = local read "Offset command file"() -> (w2220:path)
                      n805 = call-poly <vilib>:"Read From Spreadsheet File.vi"("format (%.3f)"="%.8f", "file path (dialog if empty)"=w2220) -> ("first row"=w2221:dbl[])  [unwired: 5 in, 4 out]
                    }
                  }
                  n806 = local write "Initial Positions"(w2208) -> ()
                  n807 = call <userlib>:"LVClass_WavefrontCorrector Move to Absolute Position.vi"("WavefrontCorrector in"=w2211, "Absolute Positions"=w2208, "error in (no error)"=w2207) -> ("WavefrontCorrector out"=w2212:refnum<class "WavefrontCorrector.lvclass">, "error out"=w2213:errorcluster)  [unwired: 11 in]
                  n808 = call <userlib>:"LVClass_WavefrontCorrector Get Current Position.vi"("WavefrontCorrector in"=w2212, "error in (no error)"=w2213) -> ("Wavefront Corrector Position"=w2209:T18, "error out"=w2205:errorcluster)  [unwired: 11 in, 1 out]
                  n809 = local write "Initial Positions"(w2209) -> ()
                  n810 = flat-sequence {
                    tunnel: [w2214] -> w2206
                    tunnel: w2205 -> [w2214]
                    frame #0 {
                      n811 = Wait (ms)(milliseconds to wait=u32 50) -> ()  [unwired: 1 out]
                    }
                  }
                }
              }
            }
            frame #4 {
              n812 = case shown="True" w2224 {
                tunnel: w2235 -> [_ w2250]
                tunnel: w2234 -> [_ w2249]
                tunnel: w2233 -> [_ w2248]
                tunnel: w2232 -> [_ w2247]
                tunnel: w2231 -> [_ w2246]
                tunnel: w2223 -> [w2236 w2245]
                tunnel: w2230 -> [_ w2244]
                tunnel: w2229 -> [_ w2243]
                tunnel: w2228 -> [_ w2242]
                tunnel: w2227 -> [w2237 w2240]
                tunnel: [w2237 w2239] -> w2225
                tunnel: [w2236 w2238] -> w2222
                frame False {
                }
                frame True {
                  n813 = local read "HASO ready"() -> (w2241:bool)
                  n814 = case shown="True" w2241 {
                    tunnel: w2250 -> [_ w2278]
                    tunnel: w2248 -> [_ w2277]
                    tunnel: w2247 -> [_ w2276]
                    tunnel: [w2251 w2275] -> w2239
                    tunnel: w2249 -> [_ w2274]
                    tunnel: w2242 -> [_ w2259]
                    tunnel: w2240 -> [w2251 w2258]
                    tunnel: w2245 -> [w2254 w2262]
                    tunnel: w2244 -> [w2253 w2273]
                    tunnel: [w2254 w2264] -> w2238
                    tunnel: [w2253 w2272] -> _
                    tunnel: w2246 -> [w2255 w2271]
                    tunnel: w2243 -> [w2252 w2270]
                    tunnel: [w2255 w2269] -> _
                    tunnel: [w2252 w2268] -> _
                    frame False {
                    }
                    frame True {
                      n815 = property on="nb_images (set)" class="DigNum (strict)"() -> ("Value"=w2279:u32)  [unwired: 2 in, 2 out]
                      n816 = case shown="2, Default" w2279 {
                        tunnel: [w2381 w2383] -> w2261
                        tunnel: w2274 -> [w2380 _]
                        tunnel: w2278 -> [w2381 _]
                        tunnel: [w2380 w2382] -> w2260
                        tunnel: w2277 -> [_ w2383]
                        tunnel: w2276 -> [_ w2382]
                        frame 2, Default {
                        }
                        frame 1 {
                        }
                      }
                      n817 = stacked-sequence {
                        tunnel: w2261 -> [_ w2297]
                        tunnel: w2260 -> [_ w2296]
                        tunnel: [_ w2295] -> w2257
                        tunnel: [_ w2293] -> w2256
                        tunnel: [_ w2292] -> _
                        tunnel: w2259 -> [_ w2289]
                        tunnel: w2258 -> [_ w2288]
                        frame #0 {
                          # "Delay until MD gets stable"
                          n818 = local read "exposure_duration_s (set)"() -> (w2280:dbl)
                          n819 = local read "nb_images (set)"() -> (w2281:u32)
                          n820 = Multiply(x=w2280, y=w2281) -> (x*y=w2282:dbl)
                          n821 = Add(x=w2282, y=3.0) -> (x+y=w2283:dbl)
                          n822 = Multiply(x=w2283, y=1000.0) -> (x*y=w2287:dbl)
                          n823 = To Unsigned Long Integer(number=w2287) -> (unsigned 32bit integer=w2286:u32)
                          n824 = Wait (ms)(milliseconds to wait=w2286) -> ()  [unwired: 1 out]
                        }
                        frame #1 {
                          n825 = while {
                            tunnel: w2289 -> [w2302]
                            tunnel: [w2301] -> w2291
                            tunnel: w2288 -> [w2299]
                            tunnel: [w2298] -> w2290
                            stop <- w2300 stop-if-true
                            n826 = call <userlib>:"LVClass_Camera asynchroneImageReady.vi"("Camera in"=w2302, "error in (no error)"=w2299) -> ("Camera out"=w2301:refnum<class "Camera.lvclass">, "ready"=w2300:bool, "error out"=w2298:errorcluster)  [unwired: 11 in]
                          }
                          n827 = call <userlib>:"LVClass_Camera get image.vi"("Camera in"=w2291, "Image"=w2297, "Image RAW"=w2296, "remove_background"=FALSE, "error in (no error)"=w2290) -> ("Camera out"=w2292:refnum<class "Camera.lvclass">, "Image (dup)"=w2295:refnum<class "Image.lvclass">, "error out"=w2293:errorcluster)  [unwired: 7 in, 1 out]
                        }
                      }
                      n828 = case shown="No Error" w2256 {
                        selector: w2256 -> [w2377 w2378]
                        tunnel: w2257 -> [w2374 w2379]
                        tunnel: [w2373 w2379] -> w2267
                        tunnel: [w2372 w2378] -> w2266
                        frame No Error {
                          # "get image"
                          n829 = call <userlib>:"LVClass_Image get image data.vi"("Image in"=w2374, "error in (no error)"=w2377) -> ("Image out"=w2376:refnum<class "Image.lvclass">, "Image data out"=w2371:u32[][], "error out"=w2375:errorcluster)  [unwired: 11 in]
                          n830 = call <userlib>:"LVClass_Image get image information.vi"("Image in"=w2376, "error in (no error)"=w2375) -> ("Image out"=w2373:refnum<class "Image.lvclass">, "error out"=w2372:errorcluster)  [unwired: 11 in, 1 out]
                          n831 = local write "HASO intensity"(w2371) -> ()
                        }
                        frame Error {
                        }
                      }
                      n832 = case shown="No Error" w2266 {
                        selector: w2266 -> [w2329 w2370]
                        tunnel: [w2335 w2370] -> w2275
                        tunnel: w2267 -> [w2328 _]
                        tunnel: [w2333 w2367] -> w2268
                        tunnel: [w2332 w2369] -> w2269
                        tunnel: refnum<class "HasoSlopes.lvclass"> refnum ("HasoSlopes in") -> [w2325 w2366]
                        tunnel: w2273 -> [w2324 w2368]
                        tunnel: [w2323 w2368] -> w2272
                        tunnel: w2271 -> [w2322 w2369]
                        tunnel: w2270 -> [w2320 w2367]
                        tunnel: [w2305 w2365] -> w2264
                        tunnel: [w2303 w2366] -> w2263
                        tunnel: w2262 -> [w2304 w2365]
                        frame No Error {
                          # "phaseout"
                          n833 = local read "File Base Name"() -> (w2312:string)
                          n834 = local read "Save File"() -> (w2313:bool)
                          n835 = local read "AO output"() -> (w2311:path)
                          n836 = call "image2slopes.vi"("error in (no error)"=w2329, "Image in"=w2328, "HasoEngine in"=w2324, "HasoSlopes in"=w2325) -> ("error out"=w2307:errorcluster, "HasoEngine out"=w2323:refnum<class "HasoEngine.lvclass">, "HasoSlopes out"=w2303:refnum<class "HasoSlopes.lvclass">)  [unwired: 4 in, 1 out]
                          n837 = local read "Filter"() -> (w2319:u8[])
                          n838 = call <userlib>:"LVClass_HasoSlopes Apply Substractor.vi"("HasoSlopes in"=w2304, "HasoSlopes to substract"=w2303, "error in (no error)"=w2307) -> ("HasoSlopes out"=w2308:refnum<class "HasoSlopes.lvclass">, "error out"=w2306:errorcluster)  [unwired: 11 in]
                          n839 = call "slopes2phase.vi"("TypePhase"=WavefrontReconstructionMode."Modal_Zernike", "Number of coefficients"=u8 32, "error in (no error)"=w2306, "Filter"=w2319, "HasoSlopes in"=w2308, "Phase in"=w2322) -> ("error out"=w2315:errorcluster, "HasoSlopes out"=w2316:refnum<class "HasoSlopes.lvclass">, "Phase out"=w2321:refnum<class "Phase.lvclass">)  [unwired: 3 in]
                          n840 = local read "idxType"() -> (w2310:enum16{"Wyant", "ANSI"})
                          n841 = call "slopes2zern.vi"("HasoSlopes in"=w2316, "error in (no error)"=w2315, "idxType"=w2310) -> ("HasoSlopes out"=w2305:refnum<class "HasoSlopes.lvclass">, "Zernike Coefficients"=w2309:dbl[], "error out"=w2314:errorcluster)  [unwired: 3 in, 2 out]
                          n842 = call <userlib>:"LVClass_Pupil ctor from HasoSlopes.vi"("Pupil in"=w2320, "HasoSlopes.lvclass"=w2308, "error in (no error)"=w2314) -> ("Pupil out"=w2330:refnum<class "Pupil.lvclass">, "error out"=w2331:errorcluster)  [unwired: 11 in]
                          n843 = case shown="True" w2313 {
                            tunnel: w2312 -> [_ w2341]
                            tunnel: w2311 -> [_ w2340]
                            tunnel: w2309 -> [_ w2339]
                            tunnel: w2308 -> [_ w2337]
                            tunnel: w2303 -> [_ w2338]
                            frame False {
                            }
                            frame True {
                              n844 = stacked-sequence {
                                tunnel: w2341 -> [w2345 w2352 w2358]
                                tunnel: w2340 -> [w2344 w2351 w2357]
                                tunnel: w2339 -> [_ _ w2356]
                                tunnel: w2338 -> [w2342 _ _]
                                tunnel: w2337 -> [_ w2349 _]
                                frame #0 {
                                n845 = Concatenate Strings(w2345, "_slopesOffset", ".has") -> (w2348:string)
                                n846 = Build Path(base path=w2344, name or relative path=w2348) -> (appended path=w2343:path)
                                n847 = call <userlib>:"LVClass_HasoSlopes Save.vi"("HasoSlopes in"=w2342, "path"=w2343) -> ()  [unwired: 12 in, 2 out]
                                }
                                frame #1 {
                                n848 = Concatenate Strings(w2352, "_slopesNet", ".has") -> (w2355:string)
                                n849 = Build Path(base path=w2351, name or relative path=w2355) -> (appended path=w2350:path)
                                n850 = call <userlib>:"LVClass_HasoSlopes Save.vi"("HasoSlopes in"=w2349, "path"=w2350) -> ()  [unwired: 12 in, 2 out]
                                }
                                frame #2 {
                                n851 = Concatenate Strings(w2358, "_zernCoefNet", ".txt") -> (w2361:string)
                                n852 = Build Path(base path=w2357, name or relative path=w2361) -> (appended path=w2362:path)
                                n853 = Array To Spreadsheet String(array=w2356, 3:"%f") -> (spreadsheet string=w2363:string)  [unwired: 1 in]
                                n854 = Write to Text File(file (use dialog)=w2362, text=w2363) -> ()  [unwired: 2 in, 3 out]
                                }
                              }
                            }
                          }
                          n855 = call <userlib>:"LVClasse_Phase GetStatisticDatas.vi"("Phase in"=w2321, "error in (no error)"=w2331) -> ("Phase out"=w2336:refnum<class "Phase.lvclass">, "StatisticsData"=w2317:T2, "error out"=w2334:errorcluster)  [unwired: 11 in]
                          n856 = local write "Phase statistics"(w2317) -> ()
                          n857 = call <userlib>:"LVClasse_Phase Get Data.vi"("Phase in"=w2336, "Pupil"=w2330, "error in (no error)"=w2334) -> ("Phase out"=w2332:refnum<class "Phase.lvclass">, "data"=w2318:sgl[][], "Pupil (dup)"=w2333:refnum<class "Pupil.lvclass">, "error out"=w2335:errorcluster)  [unwired: 9 in]
                          n858 = local write "Zernike Measured"(w2309) -> ()
                          n859 = local write "Phase values"(w2318) -> ()
                        }
                        frame Error {
                        }
                      }
                      n860 = call <userlib>:"LVClass_HasoSlopes dtor.vi"("HasoSlopes in"=w2263) -> ()  [unwired: 13 in, 2 out]
                    }
                  }
                }
              }
              n861 = Unbundle By Name(w2225) -> ("status"=w2226:bool)
            }
          }
        }
      }
      event "Record Batch Actuator": Mouse Up {
        n862 = local read "Coef value"() -> (w2384:dbl)
        n863 = event-data() -> ()  [unwired: 1 in, 8 out]
        n864 = local read "Idx start"() -> (w2392:u32)
        n865 = Greater Than 0?(x=w2392) -> (x > 0?=w2393:bool)
        n866 = local read "Idx end"() -> (w2390:u32)
        n867 = Less Or Equal?(x=w2390, y=52) -> (x <= y?=w2394:bool)
        n868 = Subtract(x=w2390, y=w2392) -> (x-y=w2395:u32)
        n869 = In Range and Coerce(upper limit=0.8, x=w2384, lower limit=-0.8) -> (In Range?=w2387:bool)  [unwired: 1 out]
        n870 = And(x=w2393, y=w2394) -> (x .and. y?=w2386:bool)
        n871 = Increment(x=w2395) -> (x+1=w2396:u32)
        n872 = And(x=w2386, y=w2387) -> (x .and. y?=w2385:bool)
        n873 = case shown="True" w2385 {
          tunnel: [FALSE w2440] -> w2414
          tunnel: w2413 -> [w2416 w2439]
          tunnel: [w2416 w2438] -> w2412
          tunnel: w2411 -> [w2417 w2437]
          tunnel: [w2417 w2436] -> w2409
          tunnel: w2408 -> [_ w2435]
          tunnel: w2407 -> [_ w2434]
          tunnel: w2406 -> [_ w2433]
          tunnel: w2405 -> [_ w2432]
          tunnel: w2404 -> [w2420 w2431]
          tunnel: w2403 -> [w2419 w2430]
          tunnel: w2402 -> [_ w2429]
          tunnel: w2401 -> [_ w2428]
          tunnel: [w2419 w2427] -> w2400
          tunnel: [w2420 w2426] -> w2399
          tunnel: w2398 -> [w2418 w2425]
          tunnel: [w2418 w2424] -> w2397
          tunnel: w2396 -> [_ w2423]
          tunnel: w2392 -> [_ w2422]
          tunnel: w2384 -> [_ w2421]
          frame False {
          }
          frame True {
            n874 = for {
              N: w2423 -> [_]
              tunnel: [w2462] -> w2440
              tunnel: w2435 -> [w2457]
              tunnel: w2434 -> [w2456]
              tunnel: w2433 -> [w2455]
              tunnel: w2432 -> [w2454]
              tunnel: w2429 -> [w2451]
              tunnel: w2428 -> [w2450]
              shift-right: [w2460] -> w2438
              shift-left: w2439 -> [w2461]
              shift-right: [w2458] -> w2436
              shift-left: w2437 -> [w2459]
              shift-right: [w2449] -> w2426
              shift-left: w2431 -> [w2453]
              shift-right: [w2441] -> w2427
              shift-left: w2430 -> [w2452]
              shift-right: [w2447] -> w2424
              shift-left: w2425 -> [w2448]
              tunnel: w2422 -> [w2445]
              tunnel: w2421 -> [w2443]
              i -> [w2446]
              n875 = Add(x=w2445, y=w2446) -> (x+y=w2444:u32)
              n876 = local read "Net Rp"() -> (w2442:bool)
              n877 = stacked-sequence {
                seq-local: [_ _ _ _ _ _ w2978 _] -> [_ _ _ _ _ _ _ w3001]
                seq-local: [_ _ w2559 _ _ _ _ _] -> [_ _ _ w2693 _ _ _ _]
                seq-local: [_ w2496 _ _ _ _ _ _] -> [_ _ w2560 _ _ _ _ _]
                seq-local: [_ _ w2558 _ _ _ _ _] -> [_ _ _ _ _ w2899 _ _]
                seq-local: [_ _ _ w2692 _ _ _ _] -> [_ _ _ _ w2764 _ _ _]
                seq-local: [_ _ _ _ w2765 _ _ _] -> [_ _ _ _ _ w2897 _ _]
                seq-local: [_ _ _ _ w2763 _ _ _] -> [_ _ _ _ _ w2898 _ _]
                seq-local: [_ _ _ _ _ w2896 _ _] -> [_ _ _ _ _ _ w2976 _]
                tunnel: [_ _ _ _ _ _ _ w3000] -> w2462
                tunnel: w2461 -> [_ w2492 _ _ _ _ _ _]
                tunnel: [_ _ _ _ _ _ _ w2999] -> w2460
                tunnel: w2459 -> [_ w2505 _ w2710 _ _ w2979 _]
                tunnel: [_ w2503 _ _ _ _ _ _] -> w2458
                tunnel: w2457 -> [_ _ w2572 _ w2775 w2907 _ w3009]
                tunnel: w2456 -> [_ _ w2571 _ w2774 w2906 _ w3008]
                tunnel: w2455 -> [_ _ w2570 _ w2773 w2905 _ w3007]
                tunnel: w2454 -> [_ _ w2569 _ w2772 w2904 _ w3006]
                tunnel: w2453 -> [_ _ w2568 _ w2771 w2903 _ w3005]
                tunnel: w2452 -> [_ _ w2567 _ w2770 _ _ _]
                tunnel: w2451 -> [_ _ w2566 _ w2769 _ _ w3004]
                tunnel: w2448 -> [_ _ w2565 _ w2768 w2902 _ w3003]
                tunnel: w2450 -> [_ _ w2564 _ w2767 w2901 _ w3002]
                tunnel: [_ _ w2562 _ _ _ _ _] -> w2449
                tunnel: [_ _ w2561 _ _ _ _ _] -> w2447
                tunnel: w2444 -> [w2465 w2489 _ w2697 _ _ _ _]
                tunnel: w2443 -> [_ w2488 _ w2694 _ _ _ _]
                tunnel: w2442 -> [_ _ _ _ _ _ w2977 w2998]
                tunnel: [_ _ _ _ _ w2895 _ _] -> w2441
                frame #0 {
                  # "Create output folder path"
                  n878 = Number To Decimal String(number=w2465) -> (decimal integer string=w2466:string)  [unwired: 1 in]
                  n879 = local read "Base Path"() -> (w2463:path)
                  n880 = local read "Subfolder"() -> (w2473:string)
                  n881 = Concatenate Strings("A_", w2466) -> (w2464:string)
                  n882 = Build Path(base path=w2463, name or relative path=w2473) -> (appended path=w2471:path)
                  n883 = Build Path(base path=w2471, name or relative path=w2464) -> (appended path=w2468:path)
                  n884 = local write "Current status"(w2464) -> ()
                  n885 = call <vilib>:"Check if File or Folder Exists.vi"("path"=w2471) -> ("error out"=w2470:errorcluster, "file or folder exists?"=w2472:bool)  [unwired: 8 in, 1 out]
                  n886 = case shown="True" w2472 {
                    tunnel: w2471 -> [w2478 _]
                    tunnel: w2470 -> [w2477 w2479]
                    tunnel: [w2476 w2479] -> w2469
                    frame False {
                      n887 = Create Folder(path (use dialog)=w2478, error in=w2477) -> (error out=w2476:errorcluster)  [unwired: 1 in, 2 out]
                    }
                    frame True {
                    }
                  }
                  n888 = call <vilib>:"Check if File or Folder Exists.vi"("error in (no error)"=w2469, "path"=w2468) -> ("error out"=w2474:errorcluster, "file or folder exists?"=w2475:bool)  [unwired: 7 in, 1 out]
                  n889 = case shown="False" w2475 {
                    tunnel: w2468 -> [w2481 w2485]
                    tunnel: w2474 -> [w2480 w2486]
                    frame False {
                      n890 = Create Folder(path (use dialog)=w2481, error in=w2480) -> ()  [unwired: 1 in, 3 out]
                    }
                    frame True {
                      n891 = Delete(path (use dialog)=w2485, entire hierarchy (F)=TRUE, error in=w2486) -> (deleted path=w2483:path, error out=w2482:errorcluster)  [unwired: 2 in, 1 out]
                      n892 = Create Folder(path (use dialog)=w2483, error in=w2482) -> ()  [unwired: 1 in, 3 out]
                    }
                  }
                  n893 = local write "AO output"(w2468) -> ()
                }
                frame #1 {
                  # "Delay for DM response"
                  # "Apply positive command to DM"
                  n894 = local read "Initial offset"() -> (w2504:bool)
                  n895 = case shown="True" w2504 {
                    tunnel: [w2552 w2557] -> w2497
                    frame False {
                      n896 = Initialize Array(0.0, 52) -> (w2552:dbl[])
                    }
                    frame True {
                      n897 = local read "Offset command file"() -> (w2556:path)
                      n898 = call-poly <vilib>:"Read From Spreadsheet File.vi"("format (%.3f)"="%.8f", "file path (dialog if empty)"=w2556) -> ("first row"=w2557:dbl[])  [unwired: 5 in, 4 out]
                    }
                  }
                  n899 = local read "File Base Name"() -> (w2498:string)
                  n900 = local read "AO output"() -> (w2501:path)
                  n901 = Initialize Array(0.0, 52) -> (w2490:dbl[])
                  n902 = local read "Save File"() -> (w2502:bool)
                  n903 = local write "Initial Positions"(w2497) -> ()
                  n904 = Decrement(x=w2489) -> (x-1=w2491:u32)
                  n905 = Replace Array Subset(array=w2490, new element=w2488, index=w2491) -> (w2487:dbl[])
                  n906 = Add(x=w2487, y=w2497) -> (x+y=w2499:dbl[])
                  n907 = call <userlib>:"LVClass_WavefrontCorrector Move to Absolute Position.vi"("WavefrontCorrector in"=w2505, "Absolute Positions"=w2499, "error in (no error)"=w2492) -> ("WavefrontCorrector out"=w2506:refnum<class "WavefrontCorrector.lvclass">, "error out"=w2507:errorcluster)  [unwired: 11 in]
                  n908 = call <userlib>:"LVClass_WavefrontCorrector Get Current Position.vi"("WavefrontCorrector in"=w2506, "error in (no error)"=w2507) -> ("WavefrontCorrector out"=w2503:refnum<class "WavefrontCorrector.lvclass">, "Wavefront Corrector Position"=w2500:T18, "error out"=w2495:errorcluster)  [unwired: 11 in]
                  n909 = case shown="True" w2502 {
                    tunnel: w2501 -> [_ w2515]
                    tunnel: w2498 -> [_ w2514]
                    tunnel: w2497 -> [_ w2513]
                    tunnel: w2487 -> [_ w2512]
                    tunnel: w2499 -> [_ w2511]
                    tunnel: w2500 -> [_ w2510]
                    frame False {
                    }
                    frame True {
                      n910 = stacked-sequence {
                        tunnel: w2515 -> [w2520 w2529 w2538 w2547]
                        tunnel: w2514 -> [w2518 w2527 w2536 w2545]
                        tunnel: w2513 -> [w2516 _ _ _]
                        tunnel: w2512 -> [_ w2525 _ _]
                        tunnel: w2511 -> [_ _ w2534 _]
                        tunnel: w2510 -> [_ _ _ w2543]
                        frame #0 {
                          n911 = Concatenate Strings(w2518, "_cmdOffset_1", ".dat") -> (w2521:string)
                          n912 = Build Path(base path=w2520, name or relative path=w2521) -> (appended path=w2522:path)
                          n913 = Array To Spreadsheet String(array=w2516, 3:"%f") -> (spreadsheet string=w2523:string)  [unwired: 1 in]
                          n914 = Write to Text File(file (use dialog)=w2522, text=w2523) -> ()  [unwired: 2 in, 3 out]
                        }
                        frame #1 {
                          n915 = Concatenate Strings(w2527, "_cmdAdd_1", ".dat") -> (w2530:string)
                          n916 = Build Path(base path=w2529, name or relative path=w2530) -> (appended path=w2531:path)
                          n917 = Array To Spreadsheet String(array=w2525, 3:"%f") -> (spreadsheet string=w2532:string)  [unwired: 1 in]
                          n918 = Write to Text File(file (use dialog)=w2531, text=w2532) -> ()  [unwired: 2 in, 3 out]
                        }
                        frame #2 {
                          n919 = Concatenate Strings(w2536, "_cmdFinal_1", ".dat") -> (w2539:string)
                          n920 = Build Path(base path=w2538, name or relative path=w2539) -> (appended path=w2540:path)
                          n921 = Array To Spreadsheet String(array=w2534, 3:"%f") -> (spreadsheet string=w2541:string)  [unwired: 1 in]
                          n922 = Write to Text File(file (use dialog)=w2540, text=w2541) -> ()  [unwired: 2 in, 3 out]
                        }
                        frame #3 {
                          n923 = Concatenate Strings(w2545, "_cmdFinalMirror_1", ".dat") -> (w2548:string)
                          n924 = Build Path(base path=w2547, name or relative path=w2548) -> (appended path=w2549:path)
                          n925 = Array To Spreadsheet String(array=w2543, 3:"%f") -> (spreadsheet string=w2550:string)  [unwired: 1 in]
                          n926 = Write to Text File(file (use dialog)=w2549, text=w2550) -> ()  [unwired: 2 in, 3 out]
                        }
                      }
                    }
                  }
                  n927 = local write "Final Positions"(w2499) -> ()
                  n928 = local write "DM Actuator Values"(w2500) -> ()
                  n929 = flat-sequence {
                    tunnel: [w2508] -> w2496
                    tunnel: w2495 -> [w2508]
                    frame #0 {
                      n930 = Wait (ms)(milliseconds to wait=u32 50) -> ()  [unwired: 1 out]
                    }
                  }
                }
                frame #2 {
                  n931 = local read "HASO ready"() -> (w2563:bool)
                  n932 = case shown="True" w2563 {
                    tunnel: w2572 -> [_ w2598]
                    tunnel: w2570 -> [_ w2597]
                    tunnel: w2569 -> [_ w2596]
                    tunnel: [w2573 w2595] -> w2559
                    tunnel: w2571 -> [_ w2594]
                    tunnel: w2564 -> [_ w2581]
                    tunnel: w2560 -> [w2573 w2580]
                    tunnel: w2567 -> [w2576 w2593]
                    tunnel: w2566 -> [w2575 w2592]
                    tunnel: [w2576 w2591] -> w2558
                    tunnel: [w2575 w2590] -> _
                    tunnel: w2568 -> [w2577 w2589]
                    tunnel: w2565 -> [w2574 w2588]
                    tunnel: [w2577 w2587] -> w2562
                    tunnel: [w2574 w2586] -> w2561
                    frame False {
                    }
                    frame True {
                      n933 = property on="nb_images (set)" class="DigNum (strict)"() -> ("Value"=w2599:u32)  [unwired: 2 in, 2 out]
                      n934 = case shown="2, Default" w2599 {
                        tunnel: [w2689 w2691] -> w2579
                        tunnel: w2594 -> [w2688 _]
                        tunnel: w2598 -> [w2689 _]
                        tunnel: [w2688 w2690] -> w2578
                        tunnel: w2597 -> [_ w2691]
                        tunnel: w2596 -> [_ w2690]
                        frame 2, Default {
                        }
                        frame 1 {
                        }
                      }
                      n935 = stacked-sequence {
                        tunnel: w2579 -> [_ w2617]
                        tunnel: w2578 -> [_ w2616]
                        tunnel: [_ w2615] -> w2582
                        tunnel: [_ w2613] -> w2583
                        tunnel: [_ w2612] -> _
                        tunnel: w2581 -> [_ w2609]
                        tunnel: w2580 -> [_ w2608]
                        frame #0 {
                          # "Delay until MD gets stable"
                          n936 = local read "exposure_duration_s (set)"() -> (w2600:dbl)
                          n937 = local read "nb_images (set)"() -> (w2601:u32)
                          n938 = Multiply(x=w2600, y=w2601) -> (x*y=w2602:dbl)
                          n939 = Add(x=w2602, y=3.0) -> (x+y=w2603:dbl)
                          n940 = Multiply(x=w2603, y=1000.0) -> (x*y=w2607:dbl)
                          n941 = To Unsigned Long Integer(number=w2607) -> (unsigned 32bit integer=w2606:u32)
                          n942 = Wait (ms)(milliseconds to wait=w2606) -> ()  [unwired: 1 out]
                        }
                        frame #1 {
                          n943 = while {
                            tunnel: w2609 -> [w2622]
                            tunnel: [w2621] -> w2611
                            tunnel: w2608 -> [w2619]
                            tunnel: [w2618] -> w2610
                            stop <- w2620 stop-if-true
                            n944 = call <userlib>:"LVClass_Camera asynchroneImageReady.vi"("Camera in"=w2622, "error in (no error)"=w2619) -> ("Camera out"=w2621:refnum<class "Camera.lvclass">, "ready"=w2620:bool, "error out"=w2618:errorcluster)  [unwired: 11 in]
                          }
                          n945 = call <userlib>:"LVClass_Camera get image.vi"("Camera in"=w2611, "Image"=w2617, "Image RAW"=w2616, "remove_background"=FALSE, "error in (no error)"=w2610) -> ("Camera out"=w2612:refnum<class "Camera.lvclass">, "Image (dup)"=w2615:refnum<class "Image.lvclass">, "error out"=w2613:errorcluster)  [unwired: 7 in, 1 out]
                        }
                      }
                      n946 = case shown="No Error" w2583 {
                        selector: w2583 -> [w2685 w2686]
                        tunnel: w2582 -> [w2679 w2687]
                        tunnel: [w2682 w2687] -> w2585
                        tunnel: [w2681 w2686] -> w2584
                        frame No Error {
                          # "get image"
                          n947 = call <userlib>:"LVClass_Image get image data.vi"("Image in"=w2679, "error in (no error)"=w2685) -> ("Image out"=w2684:refnum<class "Image.lvclass">, "Image data out"=w2680:u32[][], "error out"=w2683:errorcluster)  [unwired: 11 in]
                          n948 = call <userlib>:"LVClass_Image get image information.vi"("Image in"=w2684, "error in (no error)"=w2683) -> ("Image out"=w2682:refnum<class "Image.lvclass">, "error out"=w2681:errorcluster)  [unwired: 11 in, 1 out]
                          n949 = local write "HASO intensity"(w2680) -> ()
                        }
                        frame Error {
                        }
                      }
                      n950 = case shown="No Error" w2584 {
                        selector: w2584 -> [w2646 w2678]
                        tunnel: [w2652 w2678] -> w2595
                        tunnel: w2585 -> [w2645 _]
                        tunnel: [w2650 w2674] -> w2586
                        tunnel: [w2649 w2677] -> w2587
                        tunnel: w2593 -> [w2642 w2676]
                        tunnel: w2592 -> [w2641 w2675]
                        tunnel: [w2629 w2676] -> w2591
                        tunnel: [w2640 w2675] -> w2590
                        tunnel: w2589 -> [w2638 w2677]
                        tunnel: w2588 -> [w2636 w2674]
                        frame No Error {
                          # "phaseout"
                          n951 = local read "File Base Name"() -> (w2627:string)
                          n952 = local read "Save File"() -> (w2628:bool)
                          n953 = local read "AO output"() -> (w2626:path)
                          n954 = call "image2slopes.vi"("error in (no error)"=w2646, "Image in"=w2645, "HasoEngine in"=w2641, "HasoSlopes in"=w2642) -> ("error out"=w2639:errorcluster, "HasoEngine out"=w2640:refnum<class "HasoEngine.lvclass">, "HasoSlopes out"=w2623:refnum<class "HasoSlopes.lvclass">)  [unwired: 4 in, 1 out]
                          n955 = local read "Filter"() -> (w2635:u8[])
                          n956 = call "slopes2phase.vi"("TypePhase"=WavefrontReconstructionMode."Modal_Zernike", "Number of coefficients"=u8 32, "error in (no error)"=w2639, "Filter"=w2635, "HasoSlopes in"=w2623, "Phase in"=w2638) -> ("error out"=w2631:errorcluster, "HasoSlopes out"=w2632:refnum<class "HasoSlopes.lvclass">, "Phase out"=w2637:refnum<class "Phase.lvclass">)  [unwired: 3 in]
                          n957 = local read "idxType"() -> (w2625:enum16{"Wyant", "ANSI"})
                          n958 = call "slopes2zern.vi"("HasoSlopes in"=w2632, "error in (no error)"=w2631, "idxType"=w2625) -> ("HasoSlopes out"=w2629:refnum<class "HasoSlopes.lvclass">, "Zernike Coefficients"=w2624:dbl[], "error out"=w2630:errorcluster)  [unwired: 3 in, 2 out]
                          n959 = call <userlib>:"LVClass_Pupil ctor from HasoSlopes.vi"("Pupil in"=w2636, "HasoSlopes.lvclass"=w2623, "error in (no error)"=w2630) -> ("Pupil out"=w2647:refnum<class "Pupil.lvclass">, "error out"=w2648:errorcluster)  [unwired: 11 in]
                          n960 = case shown="True" w2628 {
                            tunnel: w2627 -> [_ w2657]
                            tunnel: w2626 -> [_ w2656]
                            tunnel: w2624 -> [_ w2655]
                            tunnel: w2623 -> [_ w2654]
                            frame False {
                            }
                            frame True {
                              n961 = stacked-sequence {
                                tunnel: w2657 -> [w2661 w2667]
                                tunnel: w2656 -> [w2660 w2666]
                                tunnel: w2655 -> [_ w2665]
                                tunnel: w2654 -> [w2658 _]
                                frame #0 {
                                n962 = Concatenate Strings(w2661, "_slopesMeas_1", ".has") -> (w2664:string)
                                n963 = Build Path(base path=w2660, name or relative path=w2664) -> (appended path=w2659:path)
                                n964 = call <userlib>:"LVClass_HasoSlopes Save.vi"("HasoSlopes in"=w2658, "path"=w2659) -> ()  [unwired: 12 in, 2 out]
                                }
                                frame #1 {
                                n965 = Concatenate Strings(w2667, "_zernCoefMeas_1", ".txt") -> (w2670:string)
                                n966 = Build Path(base path=w2666, name or relative path=w2670) -> (appended path=w2671:path)
                                n967 = Array To Spreadsheet String(array=w2665, 3:"%f") -> (spreadsheet string=w2672:string)  [unwired: 1 in]
                                n968 = Write to Text File(file (use dialog)=w2671, text=w2672) -> ()  [unwired: 2 in, 3 out]
                                }
                              }
                            }
                          }
                          n969 = call <userlib>:"LVClasse_Phase GetStatisticDatas.vi"("Phase in"=w2637, "error in (no error)"=w2648) -> ("Phase out"=w2653:refnum<class "Phase.lvclass">, "StatisticsData"=w2633:T2, "error out"=w2651:errorcluster)  [unwired: 11 in]
                          n970 = local write "Phase statistics"(w2633) -> ()
                          n971 = call <userlib>:"LVClasse_Phase Get Data.vi"("Phase in"=w2653, "Pupil"=w2647, "error in (no error)"=w2651) -> ("Phase out"=w2649:refnum<class "Phase.lvclass">, "data"=w2634:sgl[][], "Pupil (dup)"=w2650:refnum<class "Pupil.lvclass">, "error out"=w2652:errorcluster)  [unwired: 9 in]
                          n972 = local write "Zernike Measured"(w2624) -> ()
                          n973 = local write "Phase values"(w2634) -> ()
                        }
                        frame Error {
                        }
                      }
                    }
                  }
                }
                frame #3 {
                  # "Delay for DM response"
                  # "Apply negtive command to DM"
                  n974 = local read "Initial offset"() -> (w2709:bool)
                  n975 = case shown="True" w2709 {
                    tunnel: [w2757 w2762] -> w2703
                    frame False {
                      n976 = Initialize Array(0.0, 52) -> (w2757:dbl[])
                    }
                    frame True {
                      n977 = local read "Offset command file"() -> (w2761:path)
                      n978 = call-poly <vilib>:"Read From Spreadsheet File.vi"("format (%.3f)"="%.8f", "file path (dialog if empty)"=w2761) -> ("first row"=w2762:dbl[])  [unwired: 5 in, 4 out]
                    }
                  }
                  n979 = local read "File Base Name"() -> (w2704:string)
                  n980 = local read "AO output"() -> (w2707:path)
                  n981 = Initialize Array(0.0, 52) -> (w2698:dbl[])
                  n982 = local read "Save File"() -> (w2708:bool)
                  n983 = local write "Initial Positions"(w2703) -> ()
                  n984 = Negate(x=w2694) -> (-x=w2695:dbl)
                  n985 = Decrement(x=w2697) -> (x-1=w2699:u32)
                  n986 = Replace Array Subset(array=w2698, new element=w2695, index=w2699) -> (w2696:dbl[])
                  n987 = Add(x=w2696, y=w2703) -> (x+y=w2705:dbl[])
                  n988 = call <userlib>:"LVClass_WavefrontCorrector Move to Absolute Position.vi"("WavefrontCorrector in"=w2710, "Absolute Positions"=w2705, "error in (no error)"=w2693) -> ("WavefrontCorrector out"=w2711:refnum<class "WavefrontCorrector.lvclass">, "error out"=w2712:errorcluster)  [unwired: 11 in]
                  n989 = call <userlib>:"LVClass_WavefrontCorrector Get Current Position.vi"("WavefrontCorrector in"=w2711, "error in (no error)"=w2712) -> ("Wavefront Corrector Position"=w2706:T18, "error out"=w2702:errorcluster)  [unwired: 11 in, 1 out]
                  n990 = case shown="True" w2708 {
                    tunnel: w2707 -> [_ w2720]
                    tunnel: w2704 -> [_ w2719]
                    tunnel: w2703 -> [_ w2718]
                    tunnel: w2696 -> [_ w2717]
                    tunnel: w2705 -> [_ w2716]
                    tunnel: w2706 -> [_ w2715]
                    frame False {
                    }
                    frame True {
                      n991 = stacked-sequence {
                        tunnel: w2720 -> [w2725 w2734 w2743 w2752]
                        tunnel: w2719 -> [w2723 w2732 w2741 w2750]
                        tunnel: w2718 -> [w2721 _ _ _]
                        tunnel: w2717 -> [_ w2730 _ _]
                        tunnel: w2716 -> [_ _ w2739 _]
                        tunnel: w2715 -> [_ _ _ w2748]
                        frame #0 {
                          n992 = Concatenate Strings(w2723, "_cmdOffset_-1", ".dat") -> (w2726:string)
                          n993 = Build Path(base path=w2725, name or relative path=w2726) -> (appended path=w2727:path)
                          n994 = Array To Spreadsheet String(array=w2721, 3:"%f") -> (spreadsheet string=w2728:string)  [unwired: 1 in]
                          n995 = Write to Text File(file (use dialog)=w2727, text=w2728) -> ()  [unwired: 2 in, 3 out]
                        }
                        frame #1 {
                          n996 = Concatenate Strings(w2732, "_cmdAdd_-1", ".dat") -> (w2735:string)
                          n997 = Build Path(base path=w2734, name or relative path=w2735) -> (appended path=w2736:path)
                          n998 = Array To Spreadsheet String(array=w2730, 3:"%f") -> (spreadsheet string=w2737:string)  [unwired: 1 in]
                          n999 = Write to Text File(file (use dialog)=w2736, text=w2737) -> ()  [unwired: 2 in, 3 out]
                        }
                        frame #2 {
                          n1000 = Concatenate Strings(w2741, "_cmdFinal_-1", ".dat") -> (w2744:string)
                          n1001 = Build Path(base path=w2743, name or relative path=w2744) -> (appended path=w2745:path)
                          n1002 = Array To Spreadsheet String(array=w2739, 3:"%f") -> (spreadsheet string=w2746:string)  [unwired: 1 in]
                          n1003 = Write to Text File(file (use dialog)=w2745, text=w2746) -> ()  [unwired: 2 in, 3 out]
                        }
                        frame #3 {
                          n1004 = Concatenate Strings(w2750, "_cmdFinalMirror_-1", ".dat") -> (w2753:string)
                          n1005 = Build Path(base path=w2752, name or relative path=w2753) -> (appended path=w2754:path)
                          n1006 = Array To Spreadsheet String(array=w2748, 3:"%f") -> (spreadsheet string=w2755:string)  [unwired: 1 in]
                          n1007 = Write to Text File(file (use dialog)=w2754, text=w2755) -> ()  [unwired: 2 in, 3 out]
                        }
                      }
                    }
                  }
                  n1008 = local write "Final Positions"(w2705) -> ()
                  n1009 = local write "DM Actuator Values"(w2706) -> ()
                  n1010 = flat-sequence {
                    tunnel: [w2713] -> w2692
                    tunnel: w2702 -> [w2713]
                    frame #0 {
                      n1011 = Wait (ms)(milliseconds to wait=u32 50) -> ()  [unwired: 1 out]
                    }
                  }
                }
                frame #4 {
                  n1012 = local read "HASO ready"() -> (w2766:bool)
                  n1013 = case shown="True" w2766 {
                    tunnel: w2775 -> [_ w2801]
                    tunnel: w2773 -> [_ w2800]
                    tunnel: w2772 -> [_ w2799]
                    tunnel: [w2776 w2798] -> w2765
                    tunnel: w2774 -> [_ w2797]
                    tunnel: w2767 -> [_ w2785]
                    tunnel: w2764 -> [w2776 w2784]
                    tunnel: w2770 -> [w2779 _]
                    tunnel: w2769 -> [w2778 w2796]
                    tunnel: [w2779 w2795] -> w2763
                    tunnel: [w2778 w2794] -> _
                    tunnel: w2771 -> [w2780 w2793]
                    tunnel: w2768 -> [w2777 w2792]
                    tunnel: [w2780 w2791] -> _
                    tunnel: [w2777 w2790] -> _
                    frame False {
                    }
                    frame True {
                      n1014 = property on="nb_images (set)" class="DigNum (strict)"() -> ("Value"=w2802:u32)  [unwired: 2 in, 2 out]
                      n1015 = case shown="2, Default" w2802 {
                        tunnel: [w2892 w2894] -> w2783
                        tunnel: w2797 -> [w2891 _]
                        tunnel: w2801 -> [w2892 _]
                        tunnel: [w2891 w2893] -> w2782
                        tunnel: w2800 -> [_ w2894]
                        tunnel: w2799 -> [_ w2893]
                        frame 2, Default {
                        }
                        frame 1 {
                        }
                      }
                      n1016 = stacked-sequence {
                        tunnel: w2783 -> [_ w2820]
                        tunnel: w2782 -> [_ w2819]
                        tunnel: [_ w2818] -> w2786
                        tunnel: [_ w2816] -> w2787
                        tunnel: [_ w2815] -> _
                        tunnel: w2785 -> [_ w2812]
                        tunnel: w2784 -> [_ w2811]
                        frame #0 {
                          # "Delay until MD gets stable"
                          n1017 = local read "exposure_duration_s (set)"() -> (w2803:dbl)
                          n1018 = local read "nb_images (set)"() -> (w2804:u32)
                          n1019 = Multiply(x=w2803, y=w2804) -> (x*y=w2805:dbl)
                          n1020 = Add(x=w2805, y=3.0) -> (x+y=w2806:dbl)
                          n1021 = Multiply(x=w2806, y=1000.0) -> (x*y=w2810:dbl)
                          n1022 = To Unsigned Long Integer(number=w2810) -> (unsigned 32bit integer=w2809:u32)
                          n1023 = Wait (ms)(milliseconds to wait=w2809) -> ()  [unwired: 1 out]
                        }
                        frame #1 {
                          n1024 = while {
                            tunnel: w2812 -> [w2825]
                            tunnel: [w2824] -> w2814
                            tunnel: w2811 -> [w2822]
                            tunnel: [w2821] -> w2813
                            stop <- w2823 stop-if-true
                            n1025 = call <userlib>:"LVClass_Camera asynchroneImageReady.vi"("Camera in"=w2825, "error in (no error)"=w2822) -> ("Camera out"=w2824:refnum<class "Camera.lvclass">, "ready"=w2823:bool, "error out"=w2821:errorcluster)  [unwired: 11 in]
                          }
                          n1026 = call <userlib>:"LVClass_Camera get image.vi"("Camera in"=w2814, "Image"=w2820, "Image RAW"=w2819, "remove_background"=FALSE, "error in (no error)"=w2813) -> ("Camera out"=w2815:refnum<class "Camera.lvclass">, "Image (dup)"=w2818:refnum<class "Image.lvclass">, "error out"=w2816:errorcluster)  [unwired: 7 in, 1 out]
                        }
                      }
                      n1027 = case shown="No Error" w2787 {
                        selector: w2787 -> [w2888 w2889]
                        tunnel: w2786 -> [w2882 w2890]
                        tunnel: [w2885 w2890] -> w2789
                        tunnel: [w2884 w2889] -> w2788
                        frame No Error {
                          # "get image"
                          n1028 = call <userlib>:"LVClass_Image get image data.vi"("Image in"=w2882, "error in (no error)"=w2888) -> ("Image out"=w2887:refnum<class "Image.lvclass">, "Image data out"=w2883:u32[][], "error out"=w2886:errorcluster)  [unwired: 11 in]
                          n1029 = call <userlib>:"LVClass_Image get image information.vi"("Image in"=w2887, "error in (no error)"=w2886) -> ("Image out"=w2885:refnum<class "Image.lvclass">, "error out"=w2884:errorcluster)  [unwired: 11 in, 1 out]
                          n1030 = local write "HASO intensity"(w2883) -> ()
                        }
                        frame Error {
                        }
                      }
                      n1031 = case shown="No Error" w2788 {
                        selector: w2788 -> [w2849 w2881]
                        tunnel: [w2855 w2881] -> w2798
                        tunnel: w2789 -> [w2848 _]
                        tunnel: [w2853 w2877] -> w2790
                        tunnel: [w2852 w2880] -> w2791
                        tunnel: refnum<class "HasoSlopes.lvclass"> refnum ("HasoSlopes in") -> [w2845 w2879]
                        tunnel: w2796 -> [w2844 w2878]
                        tunnel: [w2832 w2879] -> w2795
                        tunnel: [w2843 w2878] -> w2794
                        tunnel: w2793 -> [w2841 w2880]
                        tunnel: w2792 -> [w2839 w2877]
                        frame No Error {
                          # "phaseout"
                          n1032 = local read "File Base Name"() -> (w2830:string)
                          n1033 = local read "Save File"() -> (w2831:bool)
                          n1034 = local read "AO output"() -> (w2829:path)
                          n1035 = call "image2slopes.vi"("error in (no error)"=w2849, "Image in"=w2848, "HasoEngine in"=w2844, "HasoSlopes in"=w2845) -> ("error out"=w2842:errorcluster, "HasoEngine out"=w2843:refnum<class "HasoEngine.lvclass">, "HasoSlopes out"=w2826:refnum<class "HasoSlopes.lvclass">)  [unwired: 4 in, 1 out]
                          n1036 = local read "Filter"() -> (w2838:u8[])
                          n1037 = call "slopes2phase.vi"("TypePhase"=WavefrontReconstructionMode."Modal_Zernike", "Number of coefficients"=u8 32, "error in (no error)"=w2842, "Filter"=w2838, "HasoSlopes in"=w2826, "Phase in"=w2841) -> ("error out"=w2834:errorcluster, "HasoSlopes out"=w2835:refnum<class "HasoSlopes.lvclass">, "Phase out"=w2840:refnum<class "Phase.lvclass">)  [unwired: 3 in]
                          n1038 = local read "idxType"() -> (w2828:enum16{"Wyant", "ANSI"})
                          n1039 = call "slopes2zern.vi"("HasoSlopes in"=w2835, "error in (no error)"=w2834, "idxType"=w2828) -> ("HasoSlopes out"=w2832:refnum<class "HasoSlopes.lvclass">, "Zernike Coefficients"=w2827:dbl[], "error out"=w2833:errorcluster)  [unwired: 3 in, 2 out]
                          n1040 = call <userlib>:"LVClass_Pupil ctor from HasoSlopes.vi"("Pupil in"=w2839, "HasoSlopes.lvclass"=w2826, "error in (no error)"=w2833) -> ("Pupil out"=w2850:refnum<class "Pupil.lvclass">, "error out"=w2851:errorcluster)  [unwired: 11 in]
                          n1041 = case shown="True" w2831 {
                            tunnel: w2830 -> [_ w2860]
                            tunnel: w2829 -> [_ w2859]
                            tunnel: w2827 -> [_ w2858]
                            tunnel: w2826 -> [_ w2857]
                            frame False {
                            }
                            frame True {
                              n1042 = stacked-sequence {
                                tunnel: w2860 -> [w2864 w2870]
                                tunnel: w2859 -> [w2863 w2869]
                                tunnel: w2858 -> [_ w2868]
                                tunnel: w2857 -> [w2861 _]
                                frame #0 {
                                n1043 = Concatenate Strings(w2864, "_slopesMeas_-1", ".has") -> (w2867:string)
                                n1044 = Build Path(base path=w2863, name or relative path=w2867) -> (appended path=w2862:path)
                                n1045 = call <userlib>:"LVClass_HasoSlopes Save.vi"("HasoSlopes in"=w2861, "path"=w2862) -> ()  [unwired: 12 in, 2 out]
                                }
                                frame #1 {
                                n1046 = Concatenate Strings(w2870, "_zernCoefMeas_-1", ".txt") -> (w2873:string)
                                n1047 = Build Path(base path=w2869, name or relative path=w2873) -> (appended path=w2874:path)
                                n1048 = Array To Spreadsheet String(array=w2868, 3:"%f") -> (spreadsheet string=w2875:string)  [unwired: 1 in]
                                n1049 = Write to Text File(file (use dialog)=w2874, text=w2875) -> ()  [unwired: 2 in, 3 out]
                                }
                              }
                            }
                          }
                          n1050 = call <userlib>:"LVClasse_Phase GetStatisticDatas.vi"("Phase in"=w2840, "error in (no error)"=w2851) -> ("Phase out"=w2856:refnum<class "Phase.lvclass">, "StatisticsData"=w2836:T2, "error out"=w2854:errorcluster)  [unwired: 11 in]
                          n1051 = local write "Phase statistics"(w2836) -> ()
                          n1052 = call <userlib>:"LVClasse_Phase Get Data.vi"("Phase in"=w2856, "Pupil"=w2850, "error in (no error)"=w2854) -> ("Phase out"=w2852:refnum<class "Phase.lvclass">, "data"=w2837:sgl[][], "Pupil (dup)"=w2853:refnum<class "Pupil.lvclass">, "error out"=w2855:errorcluster)  [unwired: 9 in]
                          n1053 = local write "Zernike Measured"(w2827) -> ()
                          n1054 = local write "Phase values"(w2837) -> ()
                        }
                        frame Error {
                        }
                      }
                    }
                  }
                }
                frame #5 {
                  n1055 = local read "HASO ready"() -> (w2900:bool)
                  n1056 = case shown="True" w2900 {
                    tunnel: w2907 -> [_ _]
                    tunnel: w2905 -> [_ _]
                    tunnel: w2904 -> [_ _]
                    tunnel: [w2909 w2921] -> w2896
                    tunnel: w2906 -> [_ _]
                    tunnel: w2901 -> [_ _]
                    tunnel: [w2908 w2916] -> w2895
                    tunnel: w2903 -> [w2911 w2920]
                    tunnel: w2902 -> [w2910 w2919]
                    tunnel: [w2911 w2918] -> _
                    tunnel: [w2910 w2917] -> _
                    tunnel: w2899 -> [w2908 w2914]
                    tunnel: w2898 -> [_ w2913]
                    tunnel: w2897 -> [w2909 w2912]
                    frame False {
                    }
                    frame True {
                      n1057 = case shown="No Error" w2912 {
                        selector: w2912 -> [w2923 w2975]
                        tunnel: [w2949 w2975] -> w2921
                        tunnel: [w2947 w2973] -> w2917
                        tunnel: [w2946 w2974] -> w2918
                        tunnel: w2920 -> [w2941 w2974]
                        tunnel: w2919 -> [w2939 w2973]
                        tunnel: [w2925 w2971] -> w2916
                        tunnel: [w2922 w2972] -> w2915
                        tunnel: w2914 -> [w2924 w2971]
                        tunnel: w2913 -> [w2922 w2972]
                        frame No Error {
                          # "phaseout"
                          n1058 = local read "File Base Name"() -> (w2931:string)
                          n1059 = local read "Save File"() -> (w2932:bool)
                          n1060 = local read "AO output"() -> (w2930:path)
                          n1061 = local read "Filter"() -> (w2938:u8[])
                          n1062 = call <userlib>:"LVClass_HasoSlopes Apply Substractor.vi"("HasoSlopes in"=w2924, "HasoSlopes to substract"=w2922, "error in (no error)"=w2923) -> ("HasoSlopes out"=w2927:refnum<class "HasoSlopes.lvclass">, "error out"=w2926:errorcluster)  [unwired: 11 in]
                          n1063 = call "slopes2phase.vi"("TypePhase"=WavefrontReconstructionMode."Modal_Zernike", "Number of coefficients"=u8 32, "error in (no error)"=w2926, "Filter"=w2938, "HasoSlopes in"=w2927, "Phase in"=w2941) -> ("error out"=w2934:errorcluster, "HasoSlopes out"=w2935:refnum<class "HasoSlopes.lvclass">, "Phase out"=w2940:refnum<class "Phase.lvclass">)  [unwired: 3 in]
                          n1064 = local read "idxType"() -> (w2929:enum16{"Wyant", "ANSI"})
                          n1065 = call "slopes2zern.vi"("HasoSlopes in"=w2935, "error in (no error)"=w2934, "idxType"=w2929) -> ("HasoSlopes out"=w2925:refnum<class "HasoSlopes.lvclass">, "Zernike Coefficients"=w2928:dbl[], "error out"=w2933:errorcluster)  [unwired: 3 in, 2 out]
                          n1066 = call <userlib>:"LVClass_Pupil ctor from HasoSlopes.vi"("Pupil in"=w2939, "HasoSlopes.lvclass"=w2927, "error in (no error)"=w2933) -> ("Pupil out"=w2944:refnum<class "Pupil.lvclass">, "error out"=w2945:errorcluster)  [unwired: 11 in]
                          n1067 = case shown="True" w2932 {
                            tunnel: w2931 -> [_ w2954]
                            tunnel: w2930 -> [_ w2953]
                            tunnel: w2928 -> [_ w2952]
                            tunnel: w2927 -> [_ w2951]
                            frame False {
                            }
                            frame True {
                              n1068 = stacked-sequence {
                                tunnel: w2954 -> [w2958 w2964]
                                tunnel: w2953 -> [w2957 w2963]
                                tunnel: w2952 -> [_ w2962]
                                tunnel: w2951 -> [w2955 _]
                                frame #0 {
                                n1069 = Concatenate Strings(w2958, "_slopesNet", ".has") -> (w2961:string)
                                n1070 = Build Path(base path=w2957, name or relative path=w2961) -> (appended path=w2956:path)
                                n1071 = call <userlib>:"LVClass_HasoSlopes Save.vi"("HasoSlopes in"=w2955, "path"=w2956) -> ()  [unwired: 12 in, 2 out]
                                }
                                frame #1 {
                                n1072 = Concatenate Strings(w2964, "_zernCoefNet", ".txt") -> (w2967:string)
                                n1073 = Build Path(base path=w2963, name or relative path=w2967) -> (appended path=w2968:path)
                                n1074 = Array To Spreadsheet String(array=w2962, 3:"%f") -> (spreadsheet string=w2969:string)  [unwired: 1 in]
                                n1075 = Write to Text File(file (use dialog)=w2968, text=w2969) -> ()  [unwired: 2 in, 3 out]
                                }
                              }
                            }
                          }
                          n1076 = call <userlib>:"LVClasse_Phase GetStatisticDatas.vi"("Phase in"=w2940, "error in (no error)"=w2945) -> ("Phase out"=w2950:refnum<class "Phase.lvclass">, "StatisticsData"=w2936:T2, "error out"=w2948:errorcluster)  [unwired: 11 in]
                          n1077 = local write "Phase statistics"(w2936) -> ()
                          n1078 = call <userlib>:"LVClasse_Phase Get Data.vi"("Phase in"=w2950, "Pupil"=w2944, "error in (no error)"=w2948) -> ("Phase out"=w2946:refnum<class "Phase.lvclass">, "data"=w2937:sgl[][], "Pupil (dup)"=w2947:refnum<class "Pupil.lvclass">, "error out"=w2949:errorcluster)  [unwired: 9 in]
                          n1079 = local write "Zernike Measured"(w2928) -> ()
                          n1080 = local write "Phase values"(w2937) -> ()
                        }
                        frame Error {
                        }
                      }
                      n1081 = call <userlib>:"LVClass_HasoSlopes dtor.vi"("HasoSlopes in"=w2915) -> ()  [unwired: 13 in, 2 out]
                    }
                  }
                }
                frame #6 {
                  # "Apply offset to DM"
                  n1082 = case shown="True" w2977 {
                    tunnel: w2979 -> [_ w2987]
                    tunnel: [w2980 w2982] -> w2978
                    tunnel: w2976 -> [w2980 w2983]
                    frame False {
                    }
                    frame True {
                      # "Delay for DM response"
                      n1083 = local read "Initial offset"() -> (w2986:bool)
                      n1084 = case shown="True" w2986 {
                        tunnel: [w2992 w2997] -> w2984
                        frame False {
                          n1085 = Initialize Array(0.0, 52) -> (w2992:dbl[])
                        }
                        frame True {
                          n1086 = local read "Offset command file"() -> (w2996:path)
                          n1087 = call-poly <vilib>:"Read From Spreadsheet File.vi"("format (%.3f)"="%.8f", "file path (dialog if empty)"=w2996) -> ("first row"=w2997:dbl[])  [unwired: 5 in, 4 out]
                        }
                      }
                      n1088 = local write "Initial Positions"(w2984) -> ()
                      n1089 = call <userlib>:"LVClass_WavefrontCorrector Move to Absolute Position.vi"("WavefrontCorrector in"=w2987, "Absolute Positions"=w2984, "error in (no error)"=w2983) -> ("WavefrontCorrector out"=w2988:refnum<class "WavefrontCorrector.lvclass">, "error out"=w2989:errorcluster)  [unwired: 11 in]
                      n1090 = call <userlib>:"LVClass_WavefrontCorrector Get Current Position.vi"("WavefrontCorrector in"=w2988, "error in (no error)"=w2989) -> ("Wavefront Corrector Position"=w2985:T18, "error out"=w2981:errorcluster)  [unwired: 11 in, 1 out]
                      n1091 = local write "Initial Positions"(w2985) -> ()
                      n1092 = flat-sequence {
                        tunnel: [w2990] -> w2982
                        tunnel: w2981 -> [w2990]
                        frame #0 {
                          n1093 = Wait (ms)(milliseconds to wait=u32 50) -> ()  [unwired: 1 out]
                        }
                      }
                    }
                  }
                }
                frame #7 {
                  n1094 = case shown="True" w2998 {
                    tunnel: w3009 -> [_ w3021]
                    tunnel: w3008 -> [_ w3020]
                    tunnel: w3007 -> [_ w3019]
                    tunnel: w3006 -> [_ w3018]
                    tunnel: w3005 -> [_ w3017]
                    tunnel: w3004 -> [_ w3016]
                    tunnel: w3003 -> [_ w3015]
                    tunnel: w3002 -> [_ w3014]
                    tunnel: w3001 -> [w3010 w3012]
                    tunnel: [w3010 w3011] -> w2999
                    frame False {
                    }
                    frame True {
                      n1095 = local read "HASO ready"() -> (w3013:bool)
                      n1096 = case shown="True" w3013 {
                        tunnel: w3021 -> [_ w3046]
                        tunnel: w3019 -> [_ w3045]
                        tunnel: w3018 -> [_ w3044]
                        tunnel: [w3022 w3043] -> w3011
                        tunnel: w3020 -> [_ w3042]
                        tunnel: w3014 -> [_ w3029]
                        tunnel: w3012 -> [w3022 w3028]
                        tunnel: w3016 -> [w3024 w3041]
                        tunnel: [w3024 w3040] -> _
                        tunnel: w3017 -> [w3025 w3039]
                        tunnel: w3015 -> [w3023 w3038]
                        tunnel: [w3025 w3037] -> _
                        tunnel: [w3023 w3036] -> _
                        frame False {
                        }
                        frame True {
                          n1097 = property on="nb_images (set)" class="DigNum (strict)"() -> ("Value"=w3047:u32)  [unwired: 2 in, 2 out]
                          n1098 = case shown="2, Default" w3047 {
                            tunnel: [w3136 w3138] -> w3031
                            tunnel: w3042 -> [w3135 _]
                            tunnel: w3046 -> [w3136 _]
                            tunnel: [w3135 w3137] -> w3030
                            tunnel: w3045 -> [_ w3138]
                            tunnel: w3044 -> [_ w3137]
                            frame 2, Default {
                            }
                            frame 1 {
                            }
                          }
                          n1099 = stacked-sequence {
                            tunnel: w3031 -> [_ w3065]
                            tunnel: w3030 -> [_ w3064]
                            tunnel: [_ w3063] -> w3027
                            tunnel: [_ w3061] -> w3026
                            tunnel: [_ w3060] -> _
                            tunnel: w3029 -> [_ w3057]
                            tunnel: w3028 -> [_ w3056]
                            frame #0 {
                              # "Delay until MD gets stable"
                              n1100 = local read "exposure_duration_s (set)"() -> (w3048:dbl)
                              n1101 = local read "nb_images (set)"() -> (w3049:u32)
                              n1102 = Multiply(x=w3048, y=w3049) -> (x*y=w3050:dbl)
                              n1103 = Add(x=w3050, y=3.0) -> (x+y=w3051:dbl)
                              n1104 = Multiply(x=w3051, y=1000.0) -> (x*y=w3055:dbl)
                              n1105 = To Unsigned Long Integer(number=w3055) -> (unsigned 32bit integer=w3054:u32)
                              n1106 = Wait (ms)(milliseconds to wait=w3054) -> ()  [unwired: 1 out]
                            }
                            frame #1 {
                              n1107 = while {
                                tunnel: w3057 -> [w3070]
                                tunnel: [w3069] -> w3059
                                tunnel: w3056 -> [w3067]
                                tunnel: [w3066] -> w3058
                                stop <- w3068 stop-if-true
                                n1108 = call <userlib>:"LVClass_Camera asynchroneImageReady.vi"("Camera in"=w3070, "error in (no error)"=w3067) -> ("Camera out"=w3069:refnum<class "Camera.lvclass">, "ready"=w3068:bool, "error out"=w3066:errorcluster)  [unwired: 11 in]
                              }
                              n1109 = call <userlib>:"LVClass_Camera get image.vi"("Camera in"=w3059, "Image"=w3065, "Image RAW"=w3064, "remove_background"=FALSE, "error in (no error)"=w3058) -> ("Camera out"=w3060:refnum<class "Camera.lvclass">, "Image (dup)"=w3063:refnum<class "Image.lvclass">, "error out"=w3061:errorcluster)  [unwired: 7 in, 1 out]
                            }
                          }
                          n1110 = case shown="No Error" w3026 {
                            selector: w3026 -> [w3132 w3133]
                            tunnel: w3027 -> [w3129 w3134]
                            tunnel: [w3128 w3134] -> w3035
                            tunnel: [w3127 w3133] -> w3034
                            frame No Error {
                              # "get image"
                              n1111 = call <userlib>:"LVClass_Image get image data.vi"("Image in"=w3129, "error in (no error)"=w3132) -> ("Image out"=w3131:refnum<class "Image.lvclass">, "Image data out"=w3126:u32[][], "error out"=w3130:errorcluster)  [unwired: 11 in]
                              n1112 = call <userlib>:"LVClass_Image get image information.vi"("Image in"=w3131, "error in (no error)"=w3130) -> ("Image out"=w3128:refnum<class "Image.lvclass">, "error out"=w3127:errorcluster)  [unwired: 11 in, 1 out]
                              n1113 = local write "HASO intensity"(w3126) -> ()
                            }
                            frame Error {
                            }
                          }
                          n1114 = case shown="No Error" w3034 {
                            selector: w3034 -> [w3093 w3125]
                            tunnel: [w3099 w3125] -> w3043
                            tunnel: w3035 -> [w3092 _]
                            tunnel: [w3097 w3122] -> w3036
                            tunnel: [w3096 w3124] -> w3037
                            tunnel: refnum<class "HasoSlopes.lvclass"> refnum ("HasoSlopes in") -> [w3089 w3121]
                            tunnel: w3041 -> [w3088 w3123]
                            tunnel: [w3087 w3123] -> w3040
                            tunnel: w3039 -> [w3086 w3124]
                            tunnel: w3038 -> [w3084 w3122]
                            tunnel: [w3071 w3121] -> w3032
                            frame No Error {
                              # "phaseout"
                              n1115 = local read "File Base Name"() -> (w3076:string)
                              n1116 = local read "Save File"() -> (w3077:bool)
                              n1117 = local read "AO output"() -> (w3075:path)
                              n1118 = call "image2slopes.vi"("error in (no error)"=w3093, "Image in"=w3092, "HasoEngine in"=w3088, "HasoSlopes in"=w3089) -> ("error out"=w3072:errorcluster, "HasoEngine out"=w3087:refnum<class "HasoEngine.lvclass">, "HasoSlopes out"=w3071:refnum<class "HasoSlopes.lvclass">)  [unwired: 4 in, 1 out]
                              n1119 = local read "Filter"() -> (w3083:u8[])
                              n1120 = call "slopes2phase.vi"("TypePhase"=WavefrontReconstructionMode."Modal_Zernike", "Number of coefficients"=u8 32, "error in (no error)"=w3072, "Filter"=w3083, "HasoSlopes in"=w3071, "Phase in"=w3086) -> ("error out"=w3079:errorcluster, "HasoSlopes out"=w3080:refnum<class "HasoSlopes.lvclass">, "Phase out"=w3085:refnum<class "Phase.lvclass">)  [unwired: 3 in]
                              n1121 = local read "idxType"() -> (w3074:enum16{"Wyant", "ANSI"})
                              n1122 = call "slopes2zern.vi"("HasoSlopes in"=w3080, "error in (no error)"=w3079, "idxType"=w3074) -> ("Zernike Coefficients"=w3073:dbl[], "error out"=w3078:errorcluster)  [unwired: 3 in, 3 out]
                              n1123 = call <userlib>:"LVClass_Pupil ctor from HasoSlopes.vi"("Pupil in"=w3084, "HasoSlopes.lvclass"=w3071, "error in (no error)"=w3078) -> ("Pupil out"=w3094:refnum<class "Pupil.lvclass">, "error out"=w3095:errorcluster)  [unwired: 11 in]
                              n1124 = case shown="True" w3077 {
                                tunnel: w3076 -> [_ w3104]
                                tunnel: w3075 -> [_ w3103]
                                tunnel: w3073 -> [_ w3102]
                                tunnel: w3071 -> [_ w3101]
                                frame False {
                                }
                                frame True {
                                n1125 = stacked-sequence {
                                tunnel: w3104 -> [w3108 w3114]
                                tunnel: w3103 -> [w3107 w3113]
                                tunnel: w3102 -> [_ w3112]
                                tunnel: w3101 -> [w3105 _]
                                frame #0 {
                                n1126 = Concatenate Strings(w3108, "_slopesOffset", ".has") -> (w3111:string)
                                n1127 = Build Path(base path=w3107, name or relative path=w3111) -> (appended path=w3106:path)
                                n1128 = call <userlib>:"LVClass_HasoSlopes Save.vi"("HasoSlopes in"=w3105, "path"=w3106) -> ()  [unwired: 12 in, 2 out]
                                }
                                frame #1 {
                                n1129 = Concatenate Strings(w3114, "_zernOffset", ".txt") -> (w3117:string)
                                n1130 = Build Path(base path=w3113, name or relative path=w3117) -> (appended path=w3118:path)
                                n1131 = Array To Spreadsheet String(array=w3112, 3:"%f") -> (spreadsheet string=w3119:string)  [unwired: 1 in]
                                n1132 = Write to Text File(file (use dialog)=w3118, text=w3119) -> ()  [unwired: 2 in, 3 out]
                                }
                                }
                                }
                              }
                              n1133 = call <userlib>:"LVClasse_Phase GetStatisticDatas.vi"("Phase in"=w3085, "error in (no error)"=w3095) -> ("Phase out"=w3100:refnum<class "Phase.lvclass">, "StatisticsData"=w3081:T2, "error out"=w3098:errorcluster)  [unwired: 11 in]
                              n1134 = local write "Phase statistics"(w3081) -> ()
                              n1135 = call <userlib>:"LVClasse_Phase Get Data.vi"("Phase in"=w3100, "Pupil"=w3094, "error in (no error)"=w3098) -> ("Phase out"=w3096:refnum<class "Phase.lvclass">, "data"=w3082:sgl[][], "Pupil (dup)"=w3097:refnum<class "Pupil.lvclass">, "error out"=w3099:errorcluster)  [unwired: 9 in]
                              n1136 = local write "Zernike Measured"(w3073) -> ()
                              n1137 = local write "Phase values"(w3082) -> ()
                            }
                            frame Error {
                            }
                          }
                          n1138 = call <userlib>:"LVClass_HasoSlopes dtor.vi"("HasoSlopes in"=w3032) -> ()  [unwired: 13 in, 2 out]
                        }
                      }
                    }
                  }
                  n1139 = Unbundle By Name(w2999) -> ("status"=w3000:bool)
                }
              }
            }
          }
        }
      }
      event "Record Batch Actuator PD": Mouse Up {
        n1140 = local read "Coef value"() -> (w3144:dbl)
        n1141 = event-data() -> ()  [unwired: 1 in, 8 out]
        n1142 = local read "Idx start"() -> (w3152:u32)
        n1143 = Greater Than 0?(x=w3152) -> (x > 0?=w3153:bool)
        n1144 = local read "Idx end"() -> (w3150:u32)
        n1145 = Less Or Equal?(x=w3150, y=52) -> (x <= y?=w3154:bool)
        n1146 = Subtract(x=w3150, y=w3152) -> (x-y=w3155:u32)
        n1147 = In Range and Coerce(upper limit=0.8, x=w3144, lower limit=-0.8) -> (In Range?=w3147:bool)  [unwired: 1 out]
        n1148 = And(x=w3153, y=w3154) -> (x .and. y?=w3146:bool)
        n1149 = Increment(x=w3155) -> (x+1=w3156:u32)
        n1150 = And(x=w3146, y=w3147) -> (x .and. y?=w3145:bool)
        n1151 = case shown="True" w3145 {
          tunnel: [FALSE w3181] -> w3168
          tunnel: w3167 -> [w3170 w3180]
          tunnel: [w3170 w3179] -> w3166
          tunnel: w3165 -> [w3171 w3178]
          tunnel: [w3171 w3177] -> w3163
          tunnel: w3156 -> [_ w3176]
          tunnel: w3152 -> [_ w3175]
          tunnel: w3144 -> [_ w3174]
          tunnel: w3140 -> [_ w3172]
          tunnel: w3139 -> [_ w3173]
          frame False {
          }
          frame True {
            n1152 = stacked-sequence {
              seq-local: [w3184 _ _] -> [_ _ w3445]
              seq-local: [w3185 _ _] -> [_ _ w3444]
              seq-local: [w3182 _ _] -> [_ w3191 _]
              seq-local: [_ w3190 _] -> [_ _ w3443]
              tunnel: [_ _ w3441] -> w3181
              tunnel: w3180 -> [w3183 _ _]
              tunnel: [_ _ w3442] -> w3179
              tunnel: w3178 -> [_ w3197 _]
              tunnel: [_ w3196 _] -> w3177
              tunnel: w3176 -> [_ w3195 _]
              tunnel: w3175 -> [_ w3194 _]
              tunnel: w3174 -> [_ w3193 _]
              tunnel: w3173 -> [_ w3192 _]
              tunnel: w3172 -> [w3186 _ _]
              frame #0 {
                # "Turn on laser"
                n1153 = invoke class="MG17Motor" method="SC_Enable"(reference=w3186, error in=w3183, "lChanID"=0) -> (reference out=w3185:refnum<k7>, error out=w3182:errorcluster, "lChanID"=w3184:i32)  [unwired: 1 in, 1 out]
                n1154 = Wait (ms)(milliseconds to wait=u32 1000) -> ()  [unwired: 1 out]
                n1155 = local write "EMCCD Status"(TRUE) -> ()
              }
              frame #1 {
                n1156 = for {
                  N: w3195 -> [_]
                  shift-right: [w3206] -> w3190
                  shift-left: w3191 -> [w3207]
                  shift-right: [w3204] -> w3196
                  shift-left: w3197 -> [w3205]
                  tunnel: w3194 -> [w3202]
                  tunnel: w3193 -> [w3200]
                  tunnel: w3192 -> [w3198]
                  i -> [w3203]
                  n1157 = Add(x=w3202, y=w3203) -> (x+y=w3201:u32)
                  n1158 = local read "Net Rp"() -> (w3199:bool)
                  n1159 = stacked-sequence {
                    seq-local: [_ _ _ _ _ w3403 _] -> [_ _ _ _ _ _ w3424]
                    seq-local: [_ _ w3304 _ _ _ _] -> [_ _ _ w3317 _ _ _]
                    seq-local: [_ w3242 _ _ _ _ _] -> [_ _ w3305 _ _ _ _]
                    seq-local: [_ _ _ w3318 _ _ _] -> [_ _ _ _ w3389 _ _]
                    seq-local: [_ _ _ _ w3388 _ _] -> [_ _ _ _ _ w3401 _]
                    tunnel: w3207 -> [w3208 w3239 _ _ _ _ _]
                    tunnel: [_ _ _ _ _ _ w3423] -> w3206
                    tunnel: w3205 -> [_ w3251 _ w3335 _ w3404 _]
                    tunnel: [_ w3249 _ _ _ _ _] -> w3204
                    tunnel: w3201 -> [w3211 w3236 _ w3322 _ _ _]
                    tunnel: w3200 -> [_ w3235 _ w3319 _ _ _]
                    tunnel: w3199 -> [_ _ _ _ _ w3402 w3425]
                    tunnel: w3198 -> [_ _ w3310 _ w3394 _ w3426]
                    frame #0 {
                      # "Create output folder path"
                      n1160 = Number To Decimal String(number=w3211) -> (decimal integer string=w3212:string)  [unwired: 1 in]
                      n1161 = local read "Base Path"() -> (w3209:path)
                      n1162 = local read "Subfolder"() -> (w3219:string)
                      n1163 = Concatenate Strings("A_", w3212) -> (w3210:string)
                      n1164 = Build Path(base path=w3209, name or relative path=w3219) -> (appended path=w3217:path)
                      n1165 = Build Path(base path=w3217, name or relative path=w3210) -> (appended path=w3214:path)
                      n1166 = local write "Current status"(w3210) -> ()
                      n1167 = call <vilib>:"Check if File or Folder Exists.vi"("error in (no error)"=w3208, "path"=w3217) -> ("error out"=w3216:errorcluster, "file or folder exists?"=w3218:bool)  [unwired: 7 in, 1 out]
                      n1168 = case shown="True" w3218 {
                        tunnel: w3217 -> [w3224 _]
                        tunnel: w3216 -> [w3223 w3225]
                        tunnel: [w3222 w3225] -> w3215
                        frame False {
                          n1169 = Create Folder(path (use dialog)=w3224, error in=w3223) -> (error out=w3222:errorcluster)  [unwired: 1 in, 2 out]
                        }
                        frame True {
                        }
                      }
                      n1170 = call <vilib>:"Check if File or Folder Exists.vi"("error in (no error)"=w3215, "path"=w3214) -> ("error out"=w3220:errorcluster, "file or folder exists?"=w3221:bool)  [unwired: 7 in, 1 out]
                      n1171 = case shown="False" w3221 {
                        tunnel: w3214 -> [w3227 w3231]
                        tunnel: w3220 -> [w3226 w3232]
                        frame False {
                          n1172 = Create Folder(path (use dialog)=w3227, error in=w3226) -> ()  [unwired: 1 in, 3 out]
                        }
                        frame True {
                          n1173 = Delete(path (use dialog)=w3231, entire hierarchy (F)=TRUE, error in=w3232) -> (deleted path=w3229:path, error out=w3228:errorcluster)  [unwired: 2 in, 1 out]
                          n1174 = Create Folder(path (use dialog)=w3229, error in=w3228) -> ()  [unwired: 1 in, 3 out]
                        }
                      }
                      n1175 = local write "AO output"(w3214) -> ()
                    }
                    frame #1 {
                      # "Delay for DM response"
                      # "Apply positive command to DM"
                      n1176 = local read "Initial offset"() -> (w3250:bool)
                      n1177 = case shown="True" w3250 {
                        tunnel: [w3298 w3303] -> w3243
                        frame False {
                          n1178 = Initialize Array(0.0, 52) -> (w3298:dbl[])
                        }
                        frame True {
                          n1179 = local read "Offset command file"() -> (w3302:path)
                          n1180 = call-poly <vilib>:"Read From Spreadsheet File.vi"("format (%.3f)"="%.8f", "file path (dialog if empty)"=w3302) -> ("first row"=w3303:dbl[])  [unwired: 5 in, 4 out]
                        }
                      }
                      n1181 = local read "File Base Name"() -> (w3244:string)
                      n1182 = local read "AO output"() -> (w3247:path)
                      n1183 = Initialize Array(0.0, 52) -> (w3237:dbl[])
                      n1184 = local read "Save File"() -> (w3248:bool)
                      n1185 = local write "Initial Positions"(w3243) -> ()
                      n1186 = Decrement(x=w3236) -> (x-1=w3238:u32)
                      n1187 = Replace Array Subset(array=w3237, new element=w3235, index=w3238) -> (w3234:dbl[])
                      n1188 = Add(x=w3234, y=w3243) -> (x+y=w3245:dbl[])
                      n1189 = call <userlib>:"LVClass_WavefrontCorrector Move to Absolute Position.vi"("WavefrontCorrector in"=w3251, "Absolute Positions"=w3245, "error in (no error)"=w3239) -> ("WavefrontCorrector out"=w3252:refnum<class "WavefrontCorrector.lvclass">, "error out"=w3253:errorcluster)  [unwired: 11 in]
                      n1190 = call <userlib>:"LVClass_WavefrontCorrector Get Current Position.vi"("WavefrontCorrector in"=w3252, "error in (no error)"=w3253) -> ("WavefrontCorrector out"=w3249:refnum<class "WavefrontCorrector.lvclass">, "Wavefront Corrector Position"=w3246:T18, "error out"=w3233:errorcluster)  [unwired: 11 in]
                      n1191 = case shown="True" w3248 {
                        tunnel: w3247 -> [_ w3261]
                        tunnel: w3244 -> [_ w3260]
                        tunnel: w3243 -> [_ w3259]
                        tunnel: w3234 -> [_ w3258]
                        tunnel: w3245 -> [_ w3257]
                        tunnel: w3246 -> [_ w3256]
                        frame False {
                        }
                        frame True {
                          n1192 = stacked-sequence {
                            tunnel: w3261 -> [w3266 w3275 w3284 w3293]
                            tunnel: w3260 -> [w3264 w3273 w3282 w3291]
                            tunnel: w3259 -> [w3262 _ _ _]
                            tunnel: w3258 -> [_ w3271 _ _]
                            tunnel: w3257 -> [_ _ w3280 _]
                            tunnel: w3256 -> [_ _ _ w3289]
                            frame #0 {
                              n1193 = Concatenate Strings(w3264, "_cmdOffset_1", ".dat") -> (w3267:string)
                              n1194 = Build Path(base path=w3266, name or relative path=w3267) -> (appended path=w3268:path)
                              n1195 = Array To Spreadsheet String(array=w3262, 3:"%f") -> (spreadsheet string=w3269:string)  [unwired: 1 in]
                              n1196 = Write to Text File(file (use dialog)=w3268, text=w3269) -> ()  [unwired: 2 in, 3 out]
                            }
                            frame #1 {
                              n1197 = Concatenate Strings(w3273, "_cmdAdd_1", ".dat") -> (w3276:string)
                              n1198 = Build Path(base path=w3275, name or relative path=w3276) -> (appended path=w3277:path)
                              n1199 = Array To Spreadsheet String(array=w3271, 3:"%f") -> (spreadsheet string=w3278:string)  [unwired: 1 in]
                              n1200 = Write to Text File(file (use dialog)=w3277, text=w3278) -> ()  [unwired: 2 in, 3 out]
                            }
                            frame #2 {
                              n1201 = Concatenate Strings(w3282, "_cmdFinal_1", ".dat") -> (w3285:string)
                              n1202 = Build Path(base path=w3284, name or relative path=w3285) -> (appended path=w3286:path)
                              n1203 = Array To Spreadsheet String(array=w3280, 3:"%f") -> (spreadsheet string=w3287:string)  [unwired: 1 in]
                              n1204 = Write to Text File(file (use dialog)=w3286, text=w3287) -> ()  [unwired: 2 in, 3 out]
                            }
                            frame #3 {
                              n1205 = Concatenate Strings(w3291, "_cmdFinalMirror_1", ".dat") -> (w3294:string)
                              n1206 = Build Path(base path=w3293, name or relative path=w3294) -> (appended path=w3295:path)
                              n1207 = Array To Spreadsheet String(array=w3289, 3:"%f") -> (spreadsheet string=w3296:string)  [unwired: 1 in]
                              n1208 = Write to Text File(file (use dialog)=w3295, text=w3296) -> ()  [unwired: 2 in, 3 out]
                            }
                          }
                        }
                      }
                      n1209 = local write "Final Positions"(w3245) -> ()
                      n1210 = local write "DM Actuator Values"(w3246) -> ()
                      n1211 = local write "Current error"(w3233) -> ()
                      n1212 = flat-sequence {
                        tunnel: [w3254] -> w3242
                        tunnel: w3233 -> [w3254]
                        frame #0 {
                          n1213 = Wait (ms)(milliseconds to wait=u32 50) -> ()  [unwired: 1 out]
                        }
                      }
                    }
                    frame #2 {
                      n1214 = local read "File Base Name"() -> (w3314:string)
                      n1215 = local read "AO output"() -> (w3313:path)
                      n1216 = local read "Exposure time (s)"() -> (w3307:dbl)
                      n1217 = local read "Z Step Size (um)"() -> (w3309:dbl)
                      n1218 = local read "Z Step Num"() -> (w3308:i32)
                      n1219 = local read "Z Offset (um)"() -> (w3306:dbl)
                      n1220 = Concatenate Strings(w3314, "_1") -> (w3312:string)
                      n1221 = Build Path(base path=w3313, name or relative path=w3312) -> (appended path=w3316:path)
                      n1222 = Path To String(path=w3316) -> (string=w3311:string)
                      n1223 = call "EMCCD_Stack.vi"("VISA Stage"=w3310, "strPath"=w3311, "Z Step Size (um)"=w3309, "Step Num"=w3308, "error in (no error)"=w3305, "Exposure time (s)"=w3307, "Offset"=w3306) -> ("error out"=w3304:errorcluster)  [unwired: 8 in]
                      n1224 = local write "Current error"(w3304) -> ()
                    }
                    frame #3 {
                      # "Delay for DM response"
                      # "Apply negtive command to DM"
                      n1225 = local read "Initial offset"() -> (w3334:bool)
                      n1226 = case shown="True" w3334 {
                        tunnel: [w3382 w3387] -> w3328
                        frame False {
                          n1227 = Initialize Array(0.0, 52) -> (w3382:dbl[])
                        }
                        frame True {
                          n1228 = local read "Offset command file"() -> (w3386:path)
                          n1229 = call-poly <vilib>:"Read From Spreadsheet File.vi"("format (%.3f)"="%.8f", "file path (dialog if empty)"=w3386) -> ("first row"=w3387:dbl[])  [unwired: 5 in, 4 out]
                        }
                      }
                      n1230 = local read "File Base Name"() -> (w3329:string)
                      n1231 = local read "AO output"() -> (w3332:path)
                      n1232 = Initialize Array(0.0, 52) -> (w3323:dbl[])
                      n1233 = local read "Save File"() -> (w3333:bool)
                      n1234 = local write "Initial Positions"(w3328) -> ()
                      n1235 = Negate(x=w3319) -> (-x=w3320:dbl)
                      n1236 = Decrement(x=w3322) -> (x-1=w3324:u32)
                      n1237 = Replace Array Subset(array=w3323, new element=w3320, index=w3324) -> (w3321:dbl[])
                      n1238 = Add(x=w3321, y=w3328) -> (x+y=w3330:dbl[])
                      n1239 = call <userlib>:"LVClass_WavefrontCorrector Move to Absolute Position.vi"("WavefrontCorrector in"=w3335, "Absolute Positions"=w3330, "error in (no error)"=w3317) -> ("WavefrontCorrector out"=w3336:refnum<class "WavefrontCorrector.lvclass">, "error out"=w3337:errorcluster)  [unwired: 11 in]
                      n1240 = call <userlib>:"LVClass_WavefrontCorrector Get Current Position.vi"("WavefrontCorrector in"=w3336, "error in (no error)"=w3337) -> ("Wavefront Corrector Position"=w3331:T18, "error out"=w3327:errorcluster)  [unwired: 11 in, 1 out]
                      n1241 = case shown="True" w3333 {
                        tunnel: w3332 -> [_ w3345]
                        tunnel: w3329 -> [_ w3344]
                        tunnel: w3328 -> [_ w3343]
                        tunnel: w3321 -> [_ w3342]
                        tunnel: w3330 -> [_ w3341]
                        tunnel: w3331 -> [_ w3340]
                        frame False {
                        }
                        frame True {
                          n1242 = stacked-sequence {
                            tunnel: w3345 -> [w3350 w3359 w3368 w3377]
                            tunnel: w3344 -> [w3348 w3357 w3366 w3375]
                            tunnel: w3343 -> [w3346 _ _ _]
                            tunnel: w3342 -> [_ w3355 _ _]
                            tunnel: w3341 -> [_ _ w3364 _]
                            tunnel: w3340 -> [_ _ _ w3373]
                            frame #0 {
                              n1243 = Concatenate Strings(w3348, "_cmdOffset_-1", ".dat") -> (w3351:string)
                              n1244 = Build Path(base path=w3350, name or relative path=w3351) -> (appended path=w3352:path)
                              n1245 = Array To Spreadsheet String(array=w3346, 3:"%f") -> (spreadsheet string=w3353:string)  [unwired: 1 in]
                              n1246 = Write to Text File(file (use dialog)=w3352, text=w3353) -> ()  [unwired: 2 in, 3 out]
                            }
                            frame #1 {
                              n1247 = Concatenate Strings(w3357, "_cmdAdd_-1", ".dat") -> (w3360:string)
                              n1248 = Build Path(base path=w3359, name or relative path=w3360) -> (appended path=w3361:path)
                              n1249 = Array To Spreadsheet String(array=w3355, 3:"%f") -> (spreadsheet string=w3362:string)  [unwired: 1 in]
                              n1250 = Write to Text File(file (use dialog)=w3361, text=w3362) -> ()  [unwired: 2 in, 3 out]
                            }
                            frame #2 {
                              n1251 = Concatenate Strings(w3366, "_cmdFinal_-1", ".dat") -> (w3369:string)
                              n1252 = Build Path(base path=w3368, name or relative path=w3369) -> (appended path=w3370:path)
                              n1253 = Array To Spreadsheet String(array=w3364, 3:"%f") -> (spreadsheet string=w3371:string)  [unwired: 1 in]
                              n1254 = Write to Text File(file (use dialog)=w3370, text=w3371) -> ()  [unwired: 2 in, 3 out]
                            }
                            frame #3 {
                              n1255 = Concatenate Strings(w3375, "_cmdFinalMirror_-1", ".dat") -> (w3378:string)
                              n1256 = Build Path(base path=w3377, name or relative path=w3378) -> (appended path=w3379:path)
                              n1257 = Array To Spreadsheet String(array=w3373, 3:"%f") -> (spreadsheet string=w3380:string)  [unwired: 1 in]
                              n1258 = Write to Text File(file (use dialog)=w3379, text=w3380) -> ()  [unwired: 2 in, 3 out]
                            }
                          }
                        }
                      }
                      n1259 = local write "Final Positions"(w3330) -> ()
                      n1260 = local write "DM Actuator Values"(w3331) -> ()
                      n1261 = flat-sequence {
                        tunnel: [w3338] -> w3318
                        tunnel: w3327 -> [w3338]
                        frame #0 {
                          n1262 = Wait (ms)(milliseconds to wait=u32 50) -> ()  [unwired: 1 out]
                        }
                      }
                    }
                    frame #4 {
                      n1263 = local read "File Base Name"() -> (w3398:string)
                      n1264 = local read "AO output"() -> (w3397:path)
                      n1265 = local read "Exposure time (s)"() -> (w3391:dbl)
                      n1266 = local read "Z Step Size (um)"() -> (w3393:dbl)
                      n1267 = local read "Z Step Num"() -> (w3392:i32)
                      n1268 = local read "Z Offset (um)"() -> (w3390:dbl)
                      n1269 = Concatenate Strings(w3398, "_-1") -> (w3396:string)
                      n1270 = Build Path(base path=w3397, name or relative path=w3396) -> (appended path=w3400:path)
                      n1271 = Path To String(path=w3400) -> (string=w3395:string)
                      n1272 = call "EMCCD_Stack.vi"("VISA Stage"=w3394, "strPath"=w3395, "Z Step Size (um)"=w3393, "Step Num"=w3392, "error in (no error)"=w3389, "Exposure time (s)"=w3391, "Offset"=w3390) -> ("error out"=w3388:errorcluster)  [unwired: 8 in]
                    }
                    frame #5 {
                      # "Apply offset to DM"
                      n1273 = case shown="True" w3402 {
                        tunnel: w3404 -> [_ w3412]
                        tunnel: [w3405 w3408] -> w3403
                        tunnel: w3401 -> [w3405 w3406]
                        frame False {
                        }
                        frame True {
                          # "Delay for DM response"
                          n1274 = local read "Initial offset"() -> (w3411:bool)
                          n1275 = case shown="True" w3411 {
                            tunnel: [w3417 w3422] -> w3409
                            frame False {
                              n1276 = Initialize Array(0.0, 52) -> (w3417:dbl[])
                            }
                            frame True {
                              n1277 = local read "Offset command file"() -> (w3421:path)
                              n1278 = call-poly <vilib>:"Read From Spreadsheet File.vi"("format (%.3f)"="%.8f", "file path (dialog if empty)"=w3421) -> ("first row"=w3422:dbl[])  [unwired: 5 in, 4 out]
                            }
                          }
                          n1279 = local write "Initial Positions"(w3409) -> ()
                          n1280 = call <userlib>:"LVClass_WavefrontCorrector Move to Absolute Position.vi"("WavefrontCorrector in"=w3412, "Absolute Positions"=w3409, "error in (no error)"=w3406) -> ("WavefrontCorrector out"=w3413:refnum<class "WavefrontCorrector.lvclass">, "error out"=w3414:errorcluster)  [unwired: 11 in]
                          n1281 = call <userlib>:"LVClass_WavefrontCorrector Get Current Position.vi"("WavefrontCorrector in"=w3413, "error in (no error)"=w3414) -> ("Wavefront Corrector Position"=w3410:T18, "error out"=w3407:errorcluster)  [unwired: 11 in, 1 out]
                          n1282 = local write "Initial Positions"(w3410) -> ()
                          n1283 = flat-sequence {
                            tunnel: [w3415] -> w3408
                            tunnel: w3407 -> [w3415]
                            frame #0 {
                              n1284 = Wait (ms)(milliseconds to wait=u32 50) -> ()  [unwired: 1 out]
                            }
                          }
                        }
                      }
                    }
                    frame #6 {
                      n1285 = case shown="True" w3425 {
                        tunnel: w3426 -> [_ w3434]
                        tunnel: w3424 -> [w3427 w3429]
                        tunnel: [w3427 w3428] -> w3423
                        frame False {
                        }
                        frame True {
                          n1286 = local read "File Base Name"() -> (w3438:string)
                          n1287 = local read "AO output"() -> (w3437:path)
                          n1288 = local read "Exposure time (s)"() -> (w3431:dbl)
                          n1289 = local read "Z Step Size (um)"() -> (w3433:dbl)
                          n1290 = local read "Z Step Num"() -> (w3432:i32)
                          n1291 = local read "Z Offset (um)"() -> (w3430:dbl)
                          n1292 = Concatenate Strings(w3438, "_0") -> (w3436:string)
                          n1293 = Build Path(base path=w3437, name or relative path=w3436) -> (appended path=w3440:path)
                          n1294 = Path To String(path=w3440) -> (string=w3435:string)
                          n1295 = call "EMCCD_Stack.vi"("VISA Stage"=w3434, "strPath"=w3435, "Z Step Size (um)"=w3433, "Step Num"=w3432, "error in (no error)"=w3429, "Exposure time (s)"=w3431, "Offset"=w3430) -> ("error out"=w3428:errorcluster)  [unwired: 8 in]
                        }
                      }
                    }
                  }
                }
              }
              frame #2 {
                # "Turn off laser and recover EMCCD settings"
                # "Turn off laser"
                n1296 = invoke class="MG17Motor" method="SC_Disable"(reference=w3444, error in=w3443, "lChanID"=w3445) -> (error out=w3450:errorcluster)  [unwired: 1 in, 3 out]
                n1297 = local write "Running Status"(0) -> ()
                n1298 = local read "Aquisition Mode"() -> (w3448:T6)
                n1299 = To Unsigned Word Integer(number=w3448) -> (unsigned 16bit integer=w3452:u16)
                n1300 = local write "EMCCD Status"(FALSE) -> ()
                n1301 = call <userlib>:"SetAcquisitionMode.vi"("error in (no error)"=w3450, "mode"=w3452) -> ("error out"=w3453:errorcluster)  [unwired: 1 out]
                n1302 = local read "Trigger Mode"() -> (w3449:enum16{"Internal", "External"})
                n1303 = To Unsigned Word Integer(number=w3449) -> (unsigned 16bit integer=w3451:u16)
                n1304 = call <userlib>:"SetTriggerMode.vi"("error in (no error)"=w3453, "mode"=w3451) -> ("error out"=w3442:errorcluster)  [unwired: 1 out]
                n1305 = Unbundle By Name(w3442) -> ("status"=w3441:bool)
              }
            }
          }
        }
      }
      event "Exit": Value Change {
        # "STOP AND EXIT"
        n1306 = event-data() -> ()  [unwired: 1 in, 4 out]
        n1307 = case shown="True" w3459 {
          tunnel: w3467 -> [w3470 w3473]
          tunnel: [errorcluster {"status"=FALSE, "code"=0, "source"=""} ("error out") w3472] -> w3466
          tunnel: [w3470 w3471] -> w3465
          frame False {
          }
          frame True {
            n1308 = call <userlib>:"LVClass_Camera stop acquisition.vi"("Camera in"=w3473) -> ("Camera out"=w3471:refnum<class "Camera.lvclass">, "error out"=w3472:errorcluster)  [unwired: 13 in]
          }
        }
      }
      event Panel Close? {
        n1309 = event-data() -> ()  [unwired: 1 in, 1 out]
        n1310 = flat-sequence {
          tunnel: w3489 -> [w3495]
          tunnel: w3482 -> [w3492]
          tunnel: [w3494] -> w3475
          tunnel: [w3493] -> w3474
          tunnel: [w3497] -> w3487
          tunnel: [w3498] -> w3488
          tunnel: w3475 -> [w3498]
          tunnel: w3474 -> [w3497]
          frame #0 {
            n1311 = call <userlib>:"LVClass_Camera stop acquisition.vi"("Camera in"=w3495, "error in (no error)"=w3492) -> ("Camera out"=w3494:refnum<class "Camera.lvclass">, "error out"=w3493:errorcluster)  [unwired: 12 in]
          }
          frame #1 {
            n1312 = local write "HASO ready"(FALSE) -> ()
          }
        }
        n1313 = event-data("Discard?"=TRUE) -> ()  [unwired: 1 in, 1 out]
      }
    }
    n1314 = Wait (ms)(milliseconds to wait=u32 250) -> ()  [unwired: 1 out]
  }
  n1315 = invoke class="MG17Motor" method="StopCtrl"(reference=w11) -> ()  [unwired: 2 in, 3 out]
  n1316 = VISA Close(VISA resource name=w10, error in (no error)=w6) -> (error out=w8:errorcluster)
  n1317 = case shown="True" w39 {
    tunnel: w60 -> [w3499 w3506]
    tunnel: w59 -> [_ w3530]
    tunnel: w58 -> [_ w3529]
    tunnel: w57 -> [_ w3528]
    tunnel: w56 -> [_ w3527]
    tunnel: w55 -> [_ w3526]
    tunnel: w54 -> [_ w3525]
    tunnel: w24 -> [_ w3518]
    tunnel: w20 -> [_ w3517]
    tunnel: w19 -> [_ w3516]
    tunnel: w18 -> [_ w3515]
    tunnel: w16 -> [_ w3512]
    tunnel: w17 -> [_ w3507]
    tunnel: [w3499 w3504] -> w9
    tunnel: w5 -> [_ w3500]
    frame False {
    }
    frame True {
      n1318 = local read "Enable EMCCD"() -> (w3501:bool)
      n1319 = And(x=w3500, y=w3501) -> (x .and. y?=w3502:bool)
      n1320 = flat-sequence {
        tunnel: w3530 -> [w3586]
        tunnel: w3506 -> [w3584]
        tunnel: [w3586] -> w3544
        tunnel: w3525 -> [w3585]
        tunnel: [w3585] -> w3543
        tunnel: [w3584] -> w3542
        tunnel: w3529 -> [w3583]
        tunnel: w3528 -> [w3582]
        tunnel: w3527 -> [w3581]
        tunnel: w3526 -> [w3580]
        tunnel: [w3579] -> w3541
        tunnel: [w3578] -> w3540
        tunnel: [w3577] -> w3539
        tunnel: [w3576] -> w3538
        tunnel: [w3569] -> w3523
        tunnel: [w3570] -> w3521
        tunnel: [w3571] -> w3519
        tunnel: w3518 -> [w3575]
        tunnel: w3517 -> [w3574]
        tunnel: w3516 -> [w3573]
        tunnel: w3515 -> [w3572]
        tunnel: [w3568] -> w3513
        tunnel: w3512 -> [w3567]
        tunnel: [w3566] -> w3511
        tunnel: w3507 -> [w3565]
        tunnel: [w3565] -> w3508
        tunnel: w3544 -> [w3601]
        tunnel: w3543 -> [w3600]
        tunnel: w3542 -> [w3598]
        tunnel: [w3600] -> w3537
        tunnel: [w3599] -> w3536
        tunnel: [w3598] -> w3535
        tunnel: w3541 -> [w3597]
        tunnel: [w3597] -> w3534
        tunnel: w3540 -> [w3596]
        tunnel: [w3596] -> w3533
        tunnel: w3539 -> [w3595]
        tunnel: [w3595] -> w3532
        tunnel: w3538 -> [w3594]
        tunnel: [w3594] -> w3531
        tunnel: [w3593] -> w3524
        tunnel: w3523 -> [w3593]
        tunnel: [w3592] -> w3522
        tunnel: w3521 -> [w3592]
        tunnel: [w3591] -> w3520
        tunnel: w3519 -> [w3591]
        tunnel: [w3590] -> w3514
        tunnel: w3513 -> [w3590]
        tunnel: w3511 -> [w3589]
        tunnel: [w3589] -> w3510
        tunnel: [w3588] -> w3509
        tunnel: w3508 -> [w3587]
        tunnel: w3537 -> [w3617]
        tunnel: w3536 -> [w3615]
        tunnel: w3535 -> [w3614]
        tunnel: w3534 -> [w3613]
        tunnel: w3533 -> [w3612]
        tunnel: w3532 -> [w3611]
        tunnel: w3531 -> [w3610]
        tunnel: w3524 -> [w3609]
        tunnel: w3522 -> [w3608]
        tunnel: w3520 -> [w3607]
        tunnel: w3514 -> [w3606]
        tunnel: w3510 -> [w3605]
        tunnel: w3509 -> [w3604]
        tunnel: [w3602] -> w3503
        frame #0 {
          n1321 = call <userlib>:"LVClass_Image dtor.vi"("Image in"=w3582) -> ("error out"=w3578:errorcluster)  [unwired: 13 in, 1 out]
          n1322 = local write "HASO ready"(FALSE) -> ()
          n1323 = call <userlib>:"LVClass_HasoSlopes dtor.vi"("HasoSlopes in"=w3575) -> ("error out"=w3570:errorcluster)  [unwired: 13 in, 1 out]
          n1324 = call <userlib>:"LVClass_Pupil dtor.vi"("Pupil in"=w3572) -> ("error out"=w3568:errorcluster)  [unwired: 13 in, 1 out]
          n1325 = call <userlib>:"LVClass_Image dtor.vi"("Image in"=w3580) -> ("error out"=w3576:errorcluster)  [unwired: 13 in, 1 out]
          n1326 = call <userlib>:"LVClass_WavefrontCorrector dtor.vi"("WavefrontCorrector in"=w3567) -> ("error out"=w3566:errorcluster)  [unwired: 13 in, 1 out]
          n1327 = call <userlib>:"LVClass_Image dtor.vi"("Image in"=w3583) -> ("error out"=w3579:errorcluster)  [unwired: 13 in, 1 out]
          n1328 = call <userlib>:"LVClass_Image dtor.vi"("Image in"=w3581) -> ("error out"=w3577:errorcluster)  [unwired: 13 in, 1 out]
          n1329 = call <userlib>:"LVClass_HasoEngine dtor.vi"("HasoEngine in"=w3573) -> ("error out"=w3569:errorcluster)  [unwired: 13 in, 1 out]
          n1330 = call <userlib>:"LVClasse_Phase dtor.vi"("Phase in"=w3574) -> ("error out"=w3571:errorcluster)  [unwired: 13 in, 1 out]
        }
        frame #1 {
          n1331 = call <userlib>:"LVClass_Camera dtor.vi"("Camera in"=w3601) -> ("error out"=w3599:errorcluster)  [unwired: 13 in, 1 out]
          n1332 = call <userlib>:"LVClass_WavefrontCorrectorSet dtor.vi"("WavefrontCorrectorSet in"=w3587) -> ("error out"=w3588:errorcluster)  [unwired: 13 in, 1 out]
        }
        frame #2 {
          n1333 = call <userlib>:"LVClass_CameraSet dtor.vi"("CameraSet.lvclass"=w3617) -> ("error out"=w3616:errorcluster)  [unwired: 13 in, 1 out]
          n1334 = local write "Current status"("Shut down") -> ()
          n1335 = Merge Errors(w3616, w3615, w3614, w3613, w3612, w3611, w3610, w3607, w3608, w3609, w3606, w3605, w3604) -> (w3602:errorcluster)
        }
      }
      n1336 = case shown="True" w3502 {
        tunnel: w3506 -> [w3545 w3548]
        tunnel: [w3545 w3547] -> w3505
        frame False {
        }
        frame True {
          # "Turn OFF EMCCD"
          n1337 = case shown="True" "TurnOFFCooler" {
            tunnel: w3548 -> [w3550 w3552]
            tunnel: [w3550 w3551] -> w3549
            frame False {
            }
            frame True {
              n1338 = stacked-sequence {
                tunnel: w3552 -> [w3553 w3555]
                tunnel: [_ w3554] -> w3551
                frame #0 {
                  n1339 = call <userlib>:"CoolerOFF.vi"("error in (no error)"=w3553) -> ()  [unwired: 1 in, 2 out]
                }
                frame #1 {
                  n1340 = while {
                    tunnel: w3555 -> [_]
                    tunnel: [w3557] -> w3554
                    stop <- w3559 continue-if-true
                    n1341 = call <userlib>:"GetTemperature.vi"() -> ("error out"=w3557:errorcluster, "temperature"=w3556:i32)  [unwired: 4 in, 2 out]
                    n1342 = local write "Current Temp"(w3556) -> ()
                    n1343 = Wait Until Next ms Multiple(millisecond multiple=u32 500) -> ()  [unwired: 1 out]
                    n1344 = Less?(x=w3556, y=i16 0) -> (x < y?=w3559:bool)
                  }
                }
              }
            }
          }
          n1345 = case shown="No Error" w3549 {
            tunnel: w3549 -> [w3562 w3563]
            tunnel: [w3561 w3563] -> w3547
            frame No Error {
              n1346 = call <userlib>:"ShutDown.vi"("error in (no error)"=w3562) -> ("error out"=w3561:errorcluster)  [unwired: 1 in, 1 out]
            }
            frame Error {
            }
          }
        }
      }
      n1347 = Merge Errors(w3503, w3505) -> (w3504:errorcluster)
    }
  }
  n1348 = Merge Errors(w9, w8) -> (w7:errorcluster)
  n1349 = property on="Current error" class="Clust (strict)"("Value"=w7) -> ()  [unwired: 2 in, 2 out]
